vi "GainCurveMeasurement.vi"() -> ()   [LabVIEW 2019]
doc: "Main VI for FLS imaging system."
uses:
  <vilib>/event_ctls.llb/usereventprio.ctl
  <instrlib>/niScope/Acquire/Fetch/niScope Multi Fetch Binary 16.vi
  <instrlib>/niScope/Controls/niScope trigger source.ctl
  <vilib>/Utility/file.llb/Write Delimited Spreadsheet (DBL).vi
  LaguerreDeconLib/DeconEngineClass/LaguerreDeconEngineClass.lvclass
  SubVI/GlobalVariables.vi
  SubVI/LabJack/LJ Pin Setting.ctl
  <vilib>/Utility/error.llb/DialogType.ctl
  <vilib>/Analysis/NI_AALBase.lvlib
  <vilib>/Utility/miscctls.llb/LVMinMaxIncTypeDef.ctl
  <vilib>/Analysis/baseanly.llb/Mean (DBL).vi
  <vilib>/Utility/miscctls.llb/LVPointTypeDef.ctl
  <vilib>/Instr/_visa.llb/VISA Configure Serial Port (Instr).vi
  SubVI/DigitizerConfiguration/FLImDAQ.ctl
panel:
  out "Record Backlog":i32
  out "Fetch Record #":i32
  out "error out 2":errorcluster caption="error out"
  out "error out":errorcluster
  out "Sync Success?":bool
  out "Disclamer":picture
  out "Calibration #":i8
  out "BG #":i8
  in  "TCP Connect":bool
  out "Help":string
  in  "355nm Laser toggle":bool caption="355nm 750Hz"
  in  "Cali&iRF alignment":bool
  in  "Background":bool
  in  "Aiming beam toggle":bool caption="445nm 15Hz 20mA"
  out "Lifetime 3":dbl
  out "Lifetime 2":dbl
  in  "Auto gain ch3":bool=TRUE
  in  "Auto gain ch2":bool=TRUE
  in  "Auto gain ch1":bool=TRUE
  out "Run #":i8
  in  "StopButton":bool caption="Stop"
  out "Aquisition Status:":bool
  in  "StartButton":bool caption="Start"
  in  "Gain 3":dbl min=0.0 max=4.6 step=0.1
  in  "Gain 2":dbl min=0.0 max=4.6 step=0.1
  out "Lifetime 1":dbl
  in  "Gain 1":dbl min=0.0 max=4.6 step=0.1 format="%#_4g"
  in  "Video Source":enum32{"Camera", "FrameGrabber"}(radio)
  out "Case #":string
  out "System Hardware Connection Status":T1
  out "Channel 3":dbl[][](graph)
  out "Channel 2":dbl[][](graph)
  out "Channel 1":dbl[][](graph)
  in  "Tab Control":T2(tab)
  out "Aq L?":bool
  out "ML?":bool
  out "display loop timing(ms)":u32
  out "Aquisition loop timing(ms)":u32
  in  "sine offset":dbl min=0.0 max=4.8 step=0.01
  in  "sine amplitude":dbl
  out "DisplayLoop":i32
  out "processing loop":i32
  out "processing loop timing(ms)":dbl
  in  "V target(1.5)":dbl=1.3 format="%#_13g"
  out "comm loop(ms)":u32
  out "laser EM lamp V":dbl format="%0.6f"
  in  "Show BG":bool
  in  "start Idx":i32
  in  "length":i32=50
  out "SysConfigCluster":T3
  out "LJ Pinout":T4={"Ch1 Bias"="DAC0", "Ch2 Bias"="DAC1", "Ch3 Bias"="DAC2", "355 PWM"="FIO0", "AimingBeam PWM"="FIO2", "Laser Ready"="FIO3", "Interlock"="FIO1", "Laser Start/Stop"="FIO1", "Red LED"="FIO1", "Green LED"="DIO3", "Foot Pedal"="DIO15"}
  out "FLImDAQ":T5={"Digitizer 1"="", "Digitizer 2"="", "Channel"=enum."Channel 0", "trigger source"="VAL_EXTERNAL", "trigger level"=0.5, "trigger delay"=1.35e-07, "min sample rate"=12500000000.0, "min record length"=2500, "vertical range"=1.0, "vertical offset"=-0.25, "Waveform to Avg"=2000} caption="FLIm DAQ Configuration" {"trigger delay" format="%^#.4e"; "trigger level" min=0.0 max=3.5 step=0.5 format="%.2f"; "vertical offset" format="%.4f"; "vertical range" format="%.2f"; "min sample rate" format="%#.2p"}
  out "Dig1 Temp":dbl
  out "Dig2 Temp":dbl
  in  "Sys Reconfig":bool
  out "data out(communcation loop)":string
  out "syctimer data out":string
  out "processing Error Out":errorcluster
  out "aquisition loop Error Out":errorcluster
  out "decon error out":errorcluster
  out "V1":dbl[](array[numeric])
  out "V2":dbl[](array[numeric])
  out "V3":dbl[](array[numeric])
  out "V1 Size":i32
  out "V2 Size":i32
  out "V3 Size":i32
  out "data Size":i32[](array[numeric])
  out "State log":string
  in  "Quit":bool
  in  "Radio Buttons":enum32{"No Selection", "Ch1", "Ch2", "Ch3"}(radio)=enum."Ch1" caption="DeCon Chan"
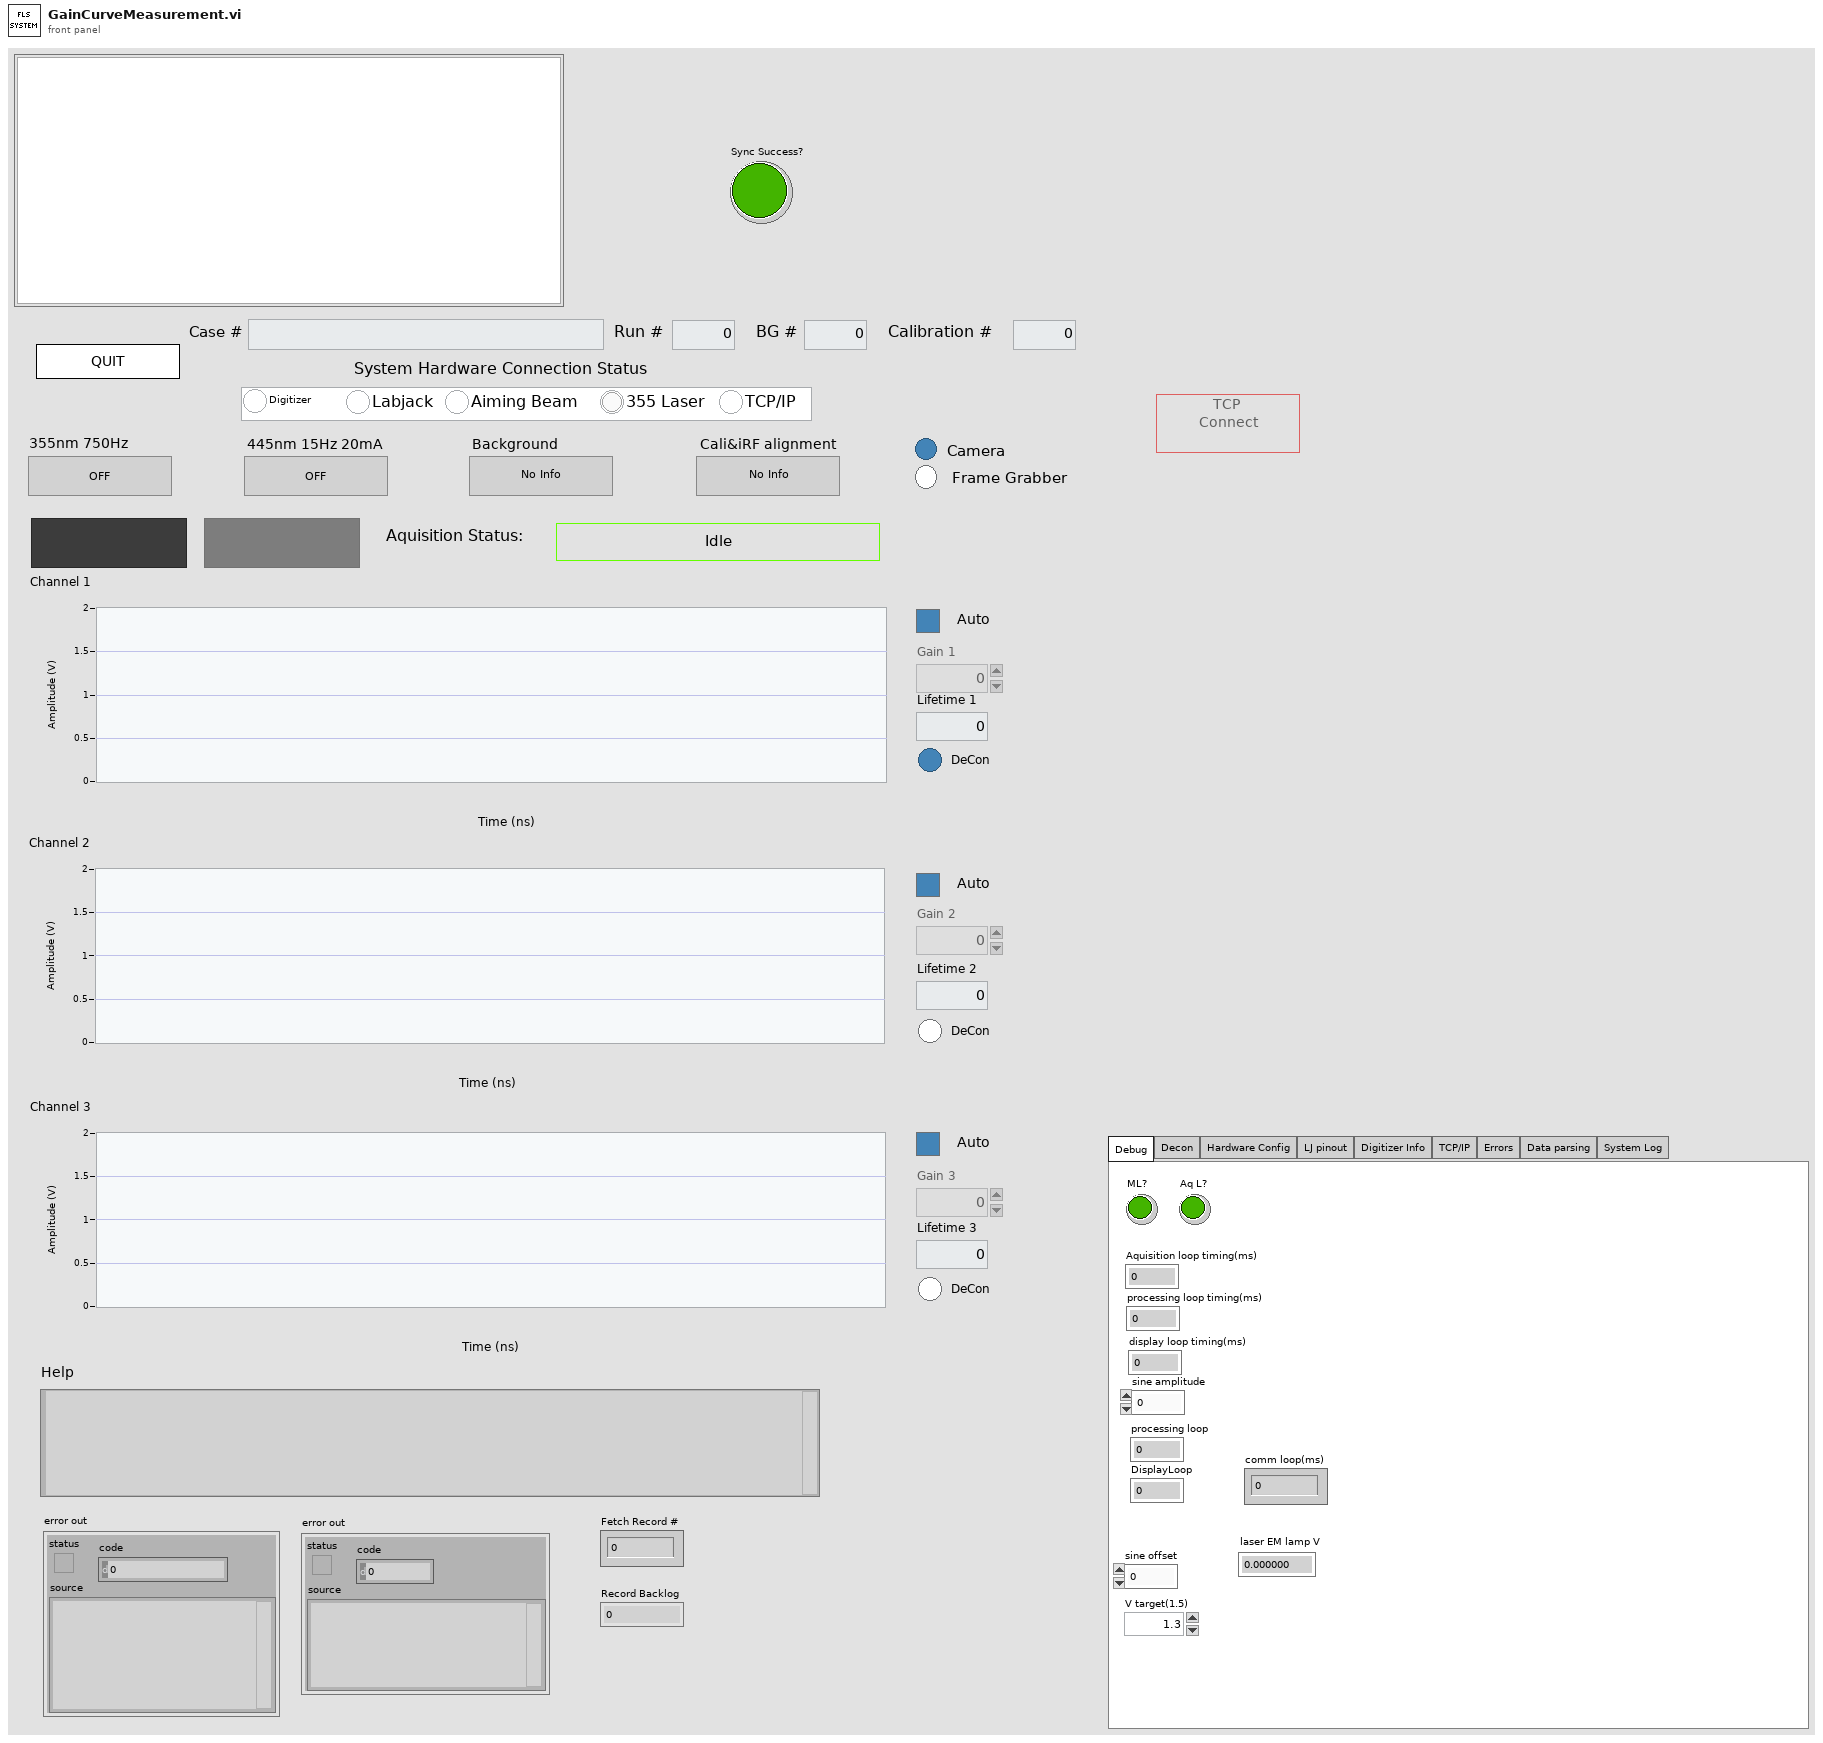
[diagram p1: front panel]
types:
  T1 = cluster{"Digitizer":bool, "Labjack":bool, "Aiming Beam":bool, "355 Laser":bool, "TCP/IP":bool}
  T2 = enum32{"Debug", "Decon", "Hardware Config", "LJ pinout", "Digitizer Info", "TCP/IP", "Errors", "Data parsing", "System Log"}
  T3 = cluster{"Ch1Enable?":bool, "Ch2Enable?":bool, "Ch3Enable?":bool, "Ch1AutoGain?":bool, "Ch2AutoGain?":bool, "Ch3AutoGain?":bool, "AimingBeamEnable?":bool}
  T4 = typedef "LJ Pin Setting.ctl" = cluster{"Ch1 Bias":string, "Ch2 Bias":string, "Ch3 Bias":string, "355 PWM":string, "AimingBeam PWM":string, "Laser Ready":string, "Interlock":string, "Laser Start/Stop":string, "Red LED":string, "Green LED":string, "Foot Pedal":string}
  T5 = typedef "FLImDAQ.ctl" = cluster{"Digitizer 1":refnum<k15>, "Digitizer 2":refnum<k15>, "Channel":enum16{"Channel 0", "Channel 1", "Channel 0&1"}, "trigger source":T6, "trigger level":dbl, "trigger delay":dbl, "min sample rate":dbl, "min record length":i32, "vertical range":dbl, "vertical offset":dbl, "Waveform to Avg":i32}
  T6 = typedef "niScope trigger source.ctl" = string
  T7 = typedef "LVPointTypeDef.ctl" = cluster{"Horizontal":i16, "Vertical":i16}
  T8 = cluster{"CH1":dbl[][], "CH2":dbl[][], "CH3":dbl[][]}
  T9 = cluster{"idx":i32, "CH1&2":dbl[][], "CH3":dbl[][]}
  T10 = enum8{"Enabled", "Disabled", "Disabled and Grayed Out"}
  T11 = enum16{"open", "open or create", "create or replace", "create", "open (read-only)"}
  T12 = enum32{"Invalid", "Standard", "Closed", "Hidden", "Minimized", "Maximized"}
  T13 = enum32{"invalid app kind", "Development System", "Run Time System", "Student Edition", "Embedded LabVIEW", "Evaluation", "Custom"}
  T14 = typedef "usereventprio.ctl" = enum32{"high priority", "normal priority"}
  T15 = enum16{"Standard", "Buffered", "CRLF", "Immediate"}
  T16 = cluster{"Core":cluster{"Current VI Reference":refnum<vi>, "Close Panel on Exit?":bool}, "SysConfigCluster":cluster{"Ch1Enable?":bool, "Ch2Enable?":bool, "Ch3Enable?":bool, "Ch1AutoGain?":bool, "Ch2AutoGain?":bool, "Ch3AutoGain?":bool, "AimingBeamEnable?":bool}, "System Status":cluster{"Digitizer":bool, "Labjack":bool, "Aiming Beam":bool, "355 Laser":bool, "TCP/IP":bool}, "IDs":cluster{"RunID":i8, "BG ID":i8, "Cali ID":i8}, "CaseID":string, "DefaultPath":path, "Pathes":cluster{"DataPath":path, "BG Path":path, "iRFPath":path, "CaliPath":path}, "FLImDAQ":cluster{"resource name":refnum<k15>, "resource name 2":refnum<k15>, "Channel":enum16{"Channel 0", "Channel 1", "Channel 0&1"}, "trigger source":T6, "trigger level":dbl, "trigger delay":dbl, "min sample rate":dbl, "min record length":i32, "vertical range":dbl, "vertical offset":dbl, "Waveform to Avg":i32}, "SysRunning?":bool, "AB Cluster":cluster{"Aiming Beam COM Port":refnum<visa-resource-name>, "Min Current":dbl, "Max Current":dbl, "Default Current":dbl, i32}, "LJ Pinout":T4, "355 PWM setting":cluster{"DIO_EF_CLOCK1_DIVISOR":i16, "DIO_EF_CLOCK1_ROLL_VALUE":i32, "DIO#_EF_INDEX":i16, "DIO#_EF_OPTIONS":i16, "DIO#_EF_CONFIG_A":i32}, "AB PWM setting":cluster{"DIO_EF_CLOCK1_DIVISOR":i16, "DIO_EF_CLOCK1_ROLL_VALUE":i32, "DIO#_EF_INDEX":i16, "DIO#_EF_OPTIONS":i16, "DIO#_EF_CONFIG_A":i32}, "Last Trigger":u32, "niTClk sessions":refnum<k20>[], "Laser start tic":u32, "TCP attempt count":i32, "Ch1Data":dbl[][], "Ch2Data":dbl[][], "Ch3Data":dbl[][], "V1":dbl[], "V2":dbl[], "V3":dbl[], "SlowTimer":u32, "FastTimer":u32, "listener ID":refnum<k5>, "TempPath":path, "LED vi reference":refnum<vi>}
  T17 = typedef "LVCursorListTypeDef.ctl" = cluster{"Name":string, "Color":u32, "Style":u8, "Point Style":u8, "Name Visible":bool, "Allow Drag":bool, "Cursor Mode":u32, "Plot":i32, "Index":i32, "Position":cluster{"X":dbl, "Y":dbl}, "X Scale":u32, "Y Scale":u32, "Watch Plots":i32[], "Watch All Plots":bool, "Plot Area":i32, "Label Offset":cluster{"X":dbl, "Y":dbl}}[]
  T18 = cluster{"Name":string, "Color":u32, "Style":u8, "Point Style":u8, "Name Visible":bool, "Allow Drag":bool, "Cursor Mode":u32, "Plot":i32, "Index":i32, "Position":cluster{"X":dbl, "Y":dbl}, "X Scale":u32, "Y Scale":u32, "Watch Plots":i32[], "Watch All Plots":bool, "Plot Area":i32, "Label Offset":cluster{"X":dbl, "Y":dbl}}
  T19 = cluster{"DataPath":path, "BG Path":path, "iRFPath":path, "CaliPath":path}
  T20 = cluster{"DIO_EF_CLOCK1_DIVISOR":i16, "DIO_EF_CLOCK1_ROLL_VALUE":i32, "DIO#_EF_INDEX":i16, "DIO#_EF_OPTIONS":i16, "DIO#_EF_CONFIG_A":i32}
  T21 = cluster{"Aiming Beam COM Port":refnum<visa-resource-name>, "Min Current":dbl, "Max Current":dbl, "Default Current":dbl, i32}
  T22 = cluster{"resource name":refnum<k15>, "resource name 2":refnum<k15>, "Channel":enum16{"Channel 0", "Channel 1", "Channel 0&1"}, "trigger source":T6, "trigger level":dbl, "trigger delay":dbl, "min sample rate":dbl, "min record length":i32, "vertical range":dbl, "vertical offset":dbl, "Waveform to Avg":i32}
  T23 = cluster{"Current VI Reference":refnum<vi>, "Close Panel on Exit?":bool}
  T24 = cluster{"1D Avg":dbl[], "1D Avg":dbl[], "1D Avg":dbl[]}
  T25 = typedef "DialogType.ctl" = u16
  T26 = cluster{"Ch1 iRF":dbl[], "Ch2 iRF":dbl[], "Ch3 iRF":dbl[]}
  T27 = typedef "LJ PWM Setting.ctl" = cluster{"DIO_EF_CLOCK1_DIVISOR":i16, "DIO_EF_CLOCK1_ROLL_VALUE":i32, "DIO#_EF_INDEX":i16, "DIO#_EF_OPTIONS":i16, "DIO#_EF_CONFIG_A":i32}
  T28 = typedef "AimingBeam.ctl" = cluster{"Aiming Beam COM Port":refnum<visa-resource-name>, "Min Current":dbl, "Max Current":dbl, "Default Current":dbl, "Frequency(Hz)":u32}
  T29 = typedef "LVMinMaxIncTypeDef.ctl" = cluster{"Minimum":dbl, "Maximum":dbl, "Increment":dbl}
  T30 = typedef "LVBoundsTypeDef.ctl" = cluster{"Width":u32, "Height":u32}
  T31 = typedef "imagedata.ctl" = cluster{"image type":i32, "image depth":i32, "image":u8[], "mask":u8[], "colors":u32[], "Rectangle":cluster{"left":i16, "top":i16, "right":i16, "bottom":i16}}
  T32 = cluster{"V1 out":dbl, "V2 out":dbl, "V3 out":dbl}
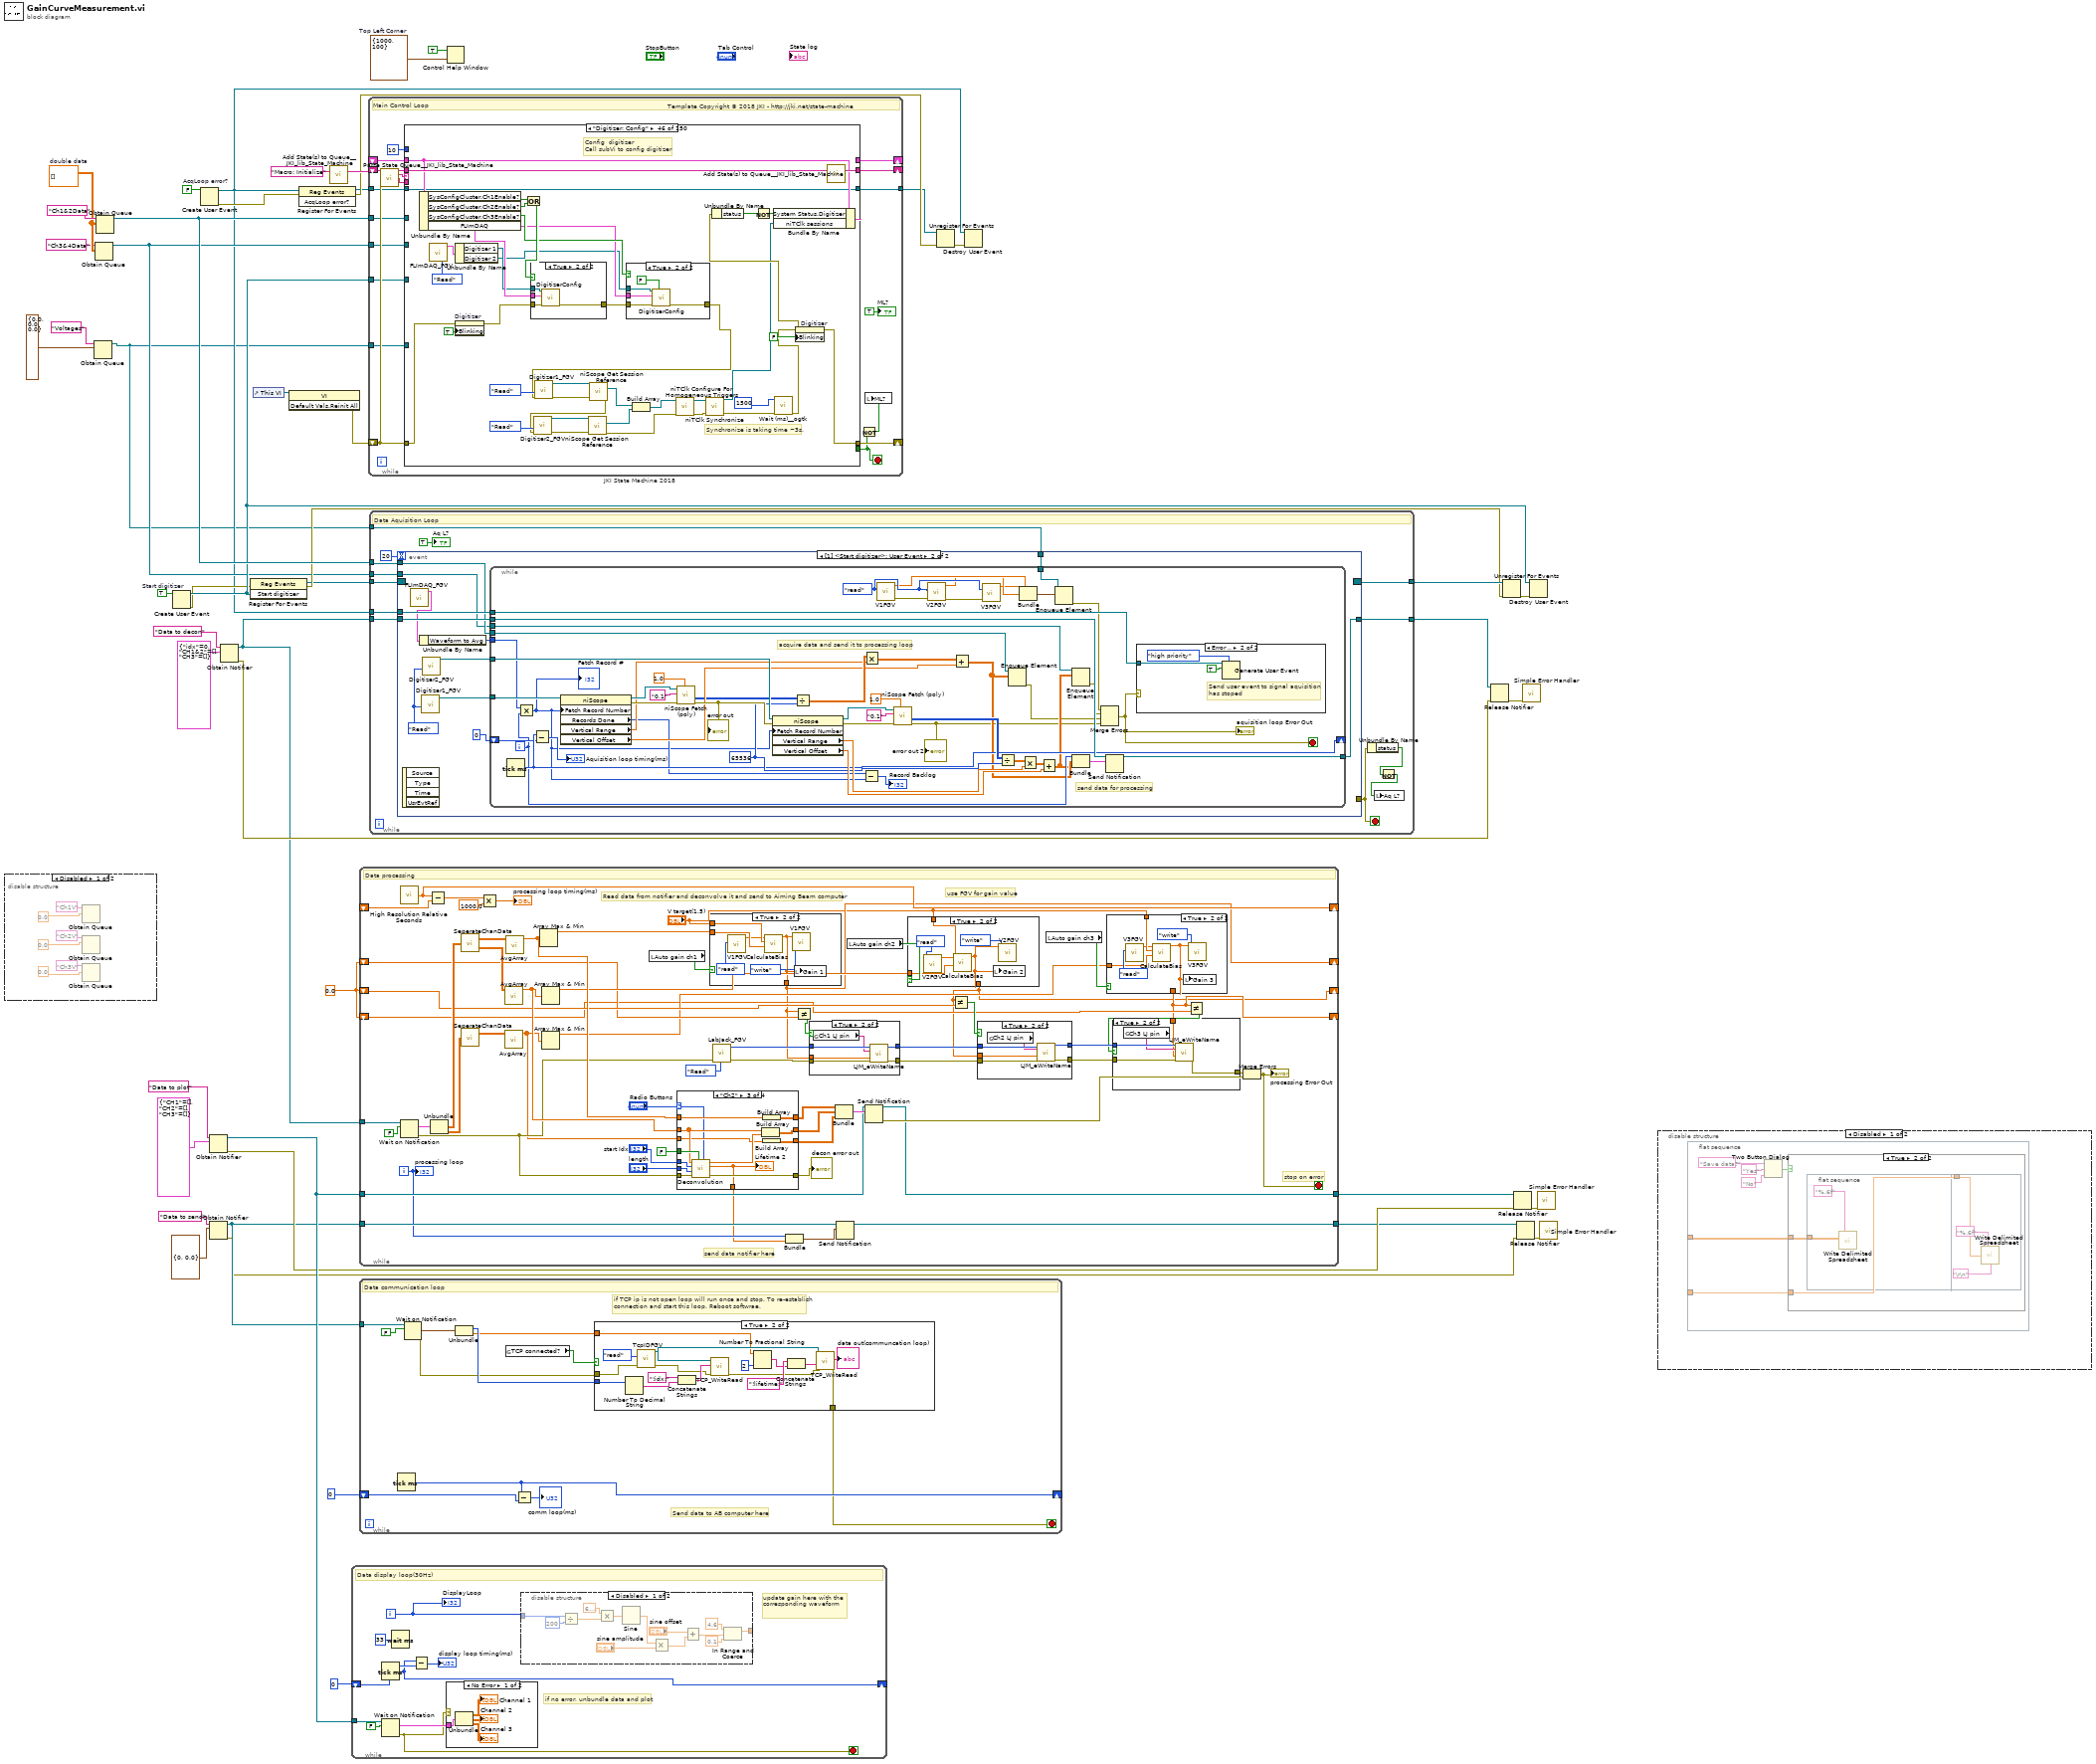
[diagram p0: block diagram]
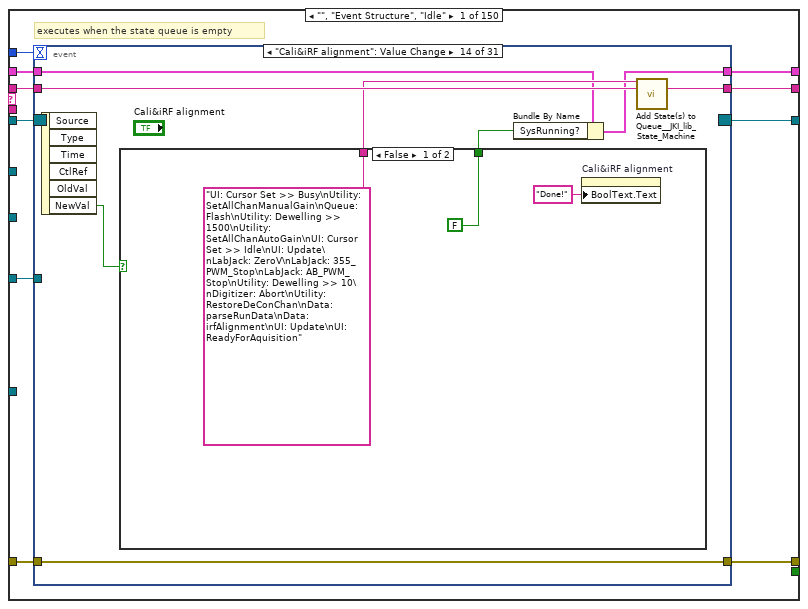
[diagram p3: hidden frame]
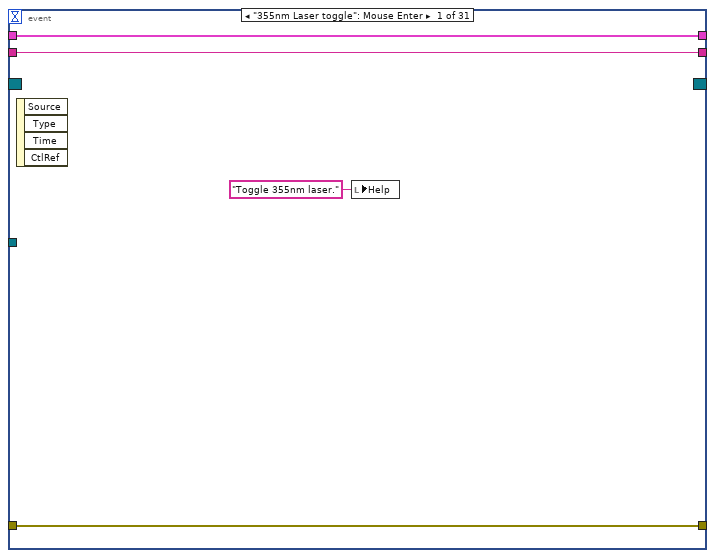
[diagram p4: hidden frame]
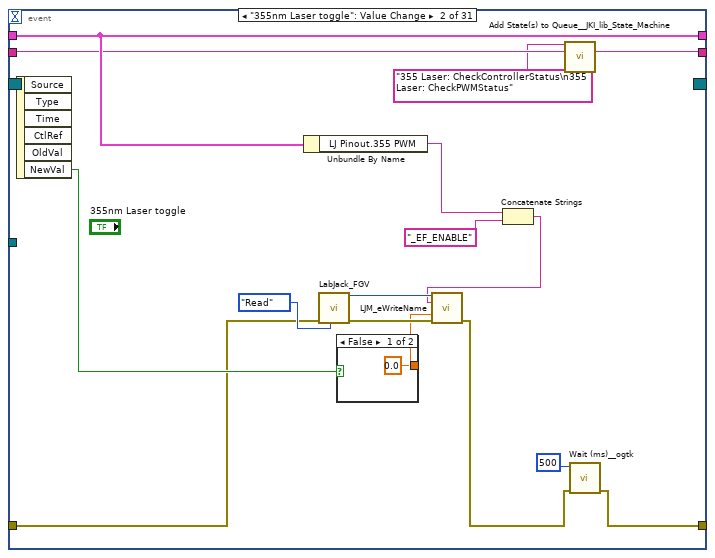
[diagram p5: hidden frame]
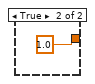
[diagram p6: hidden frame]
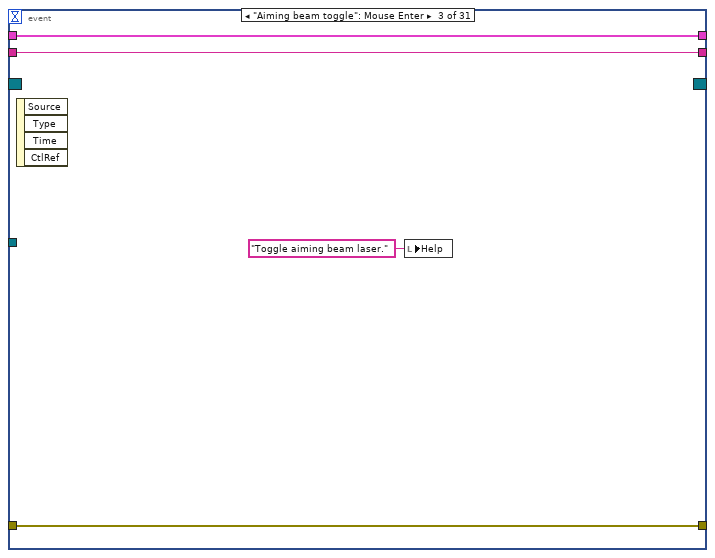
[diagram p7: hidden frame]
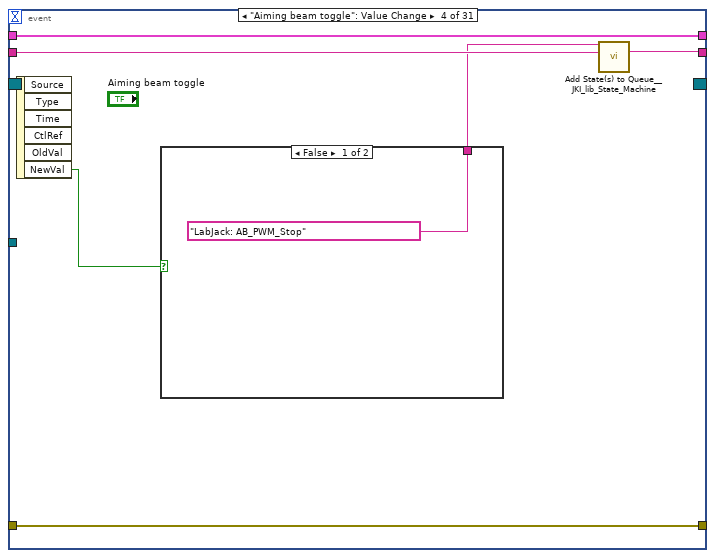
[diagram p8: hidden frame]
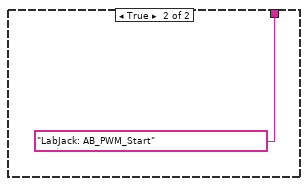
[diagram p9: hidden frame]
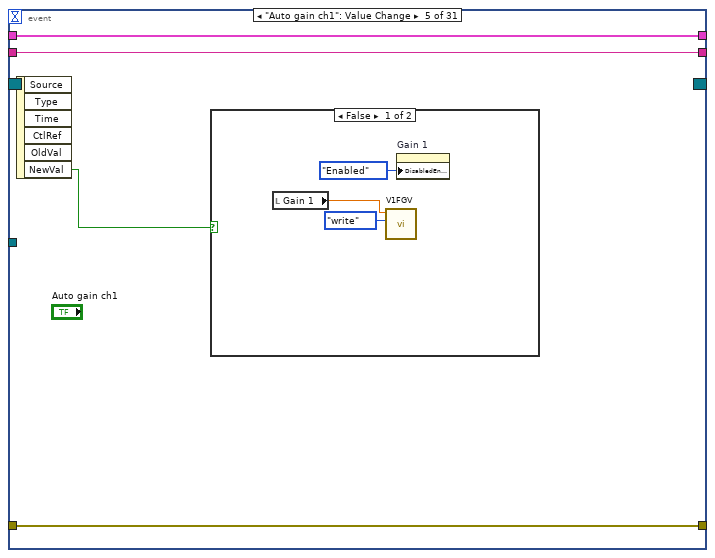
[diagram p10: hidden frame]
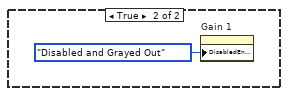
[diagram p11: hidden frame]
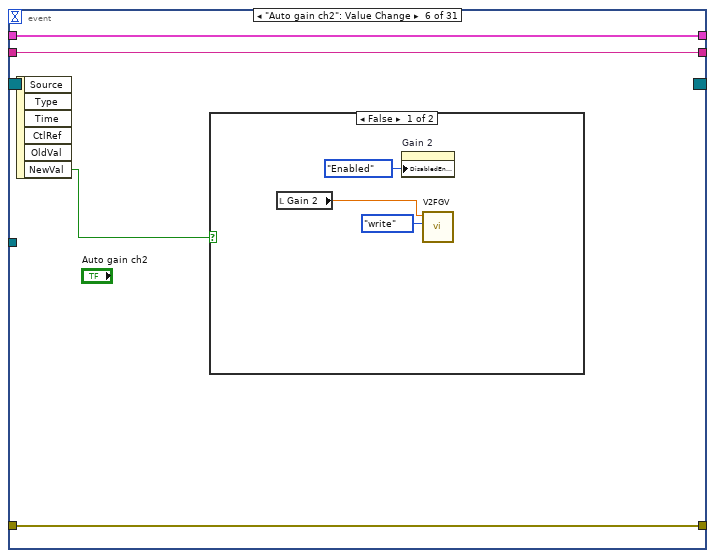
[diagram p12: hidden frame]
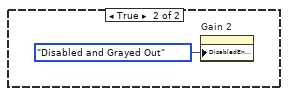
[diagram p13: hidden frame]
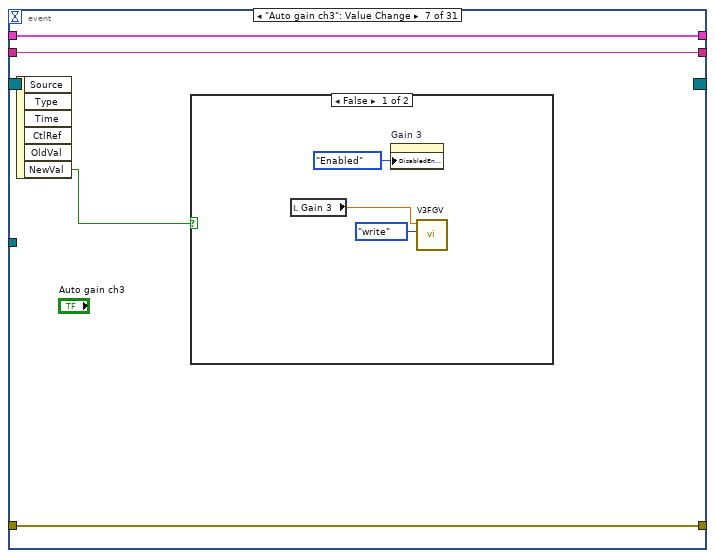
[diagram p14: hidden frame]
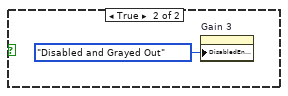
[diagram p15: hidden frame]
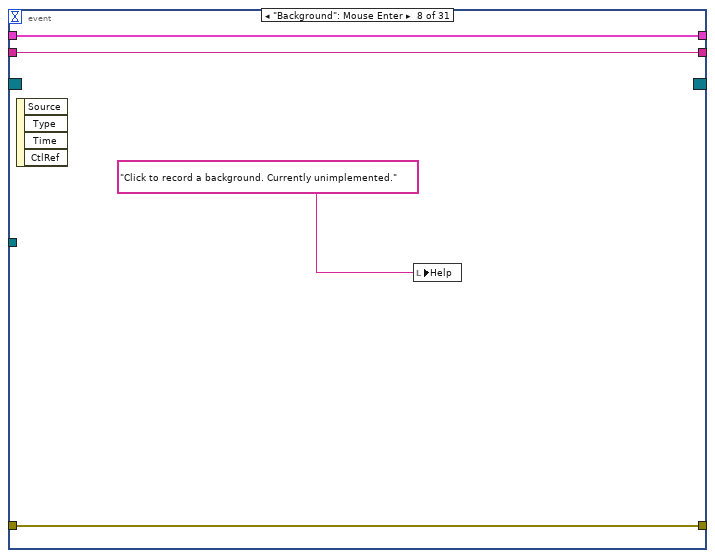
[diagram p16: hidden frame]
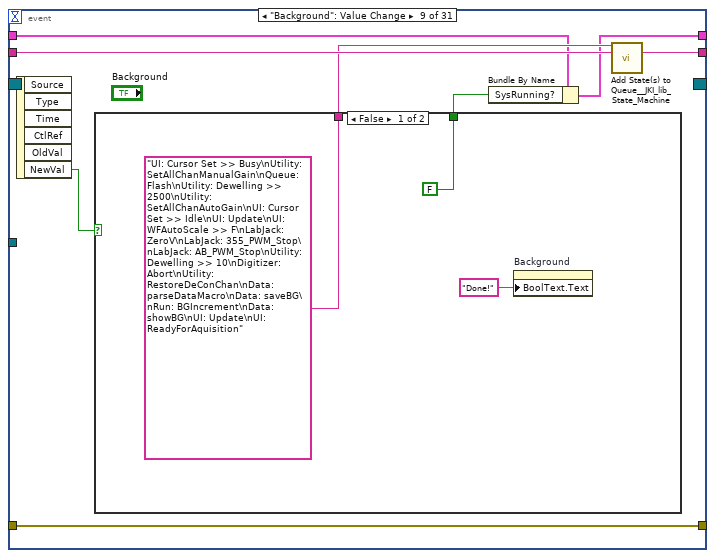
[diagram p17: hidden frame]
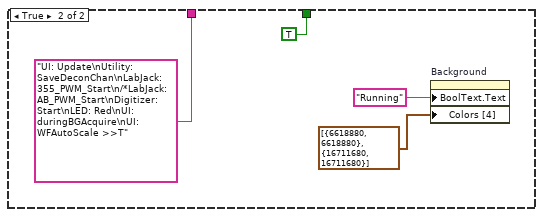
[diagram p18: hidden frame]
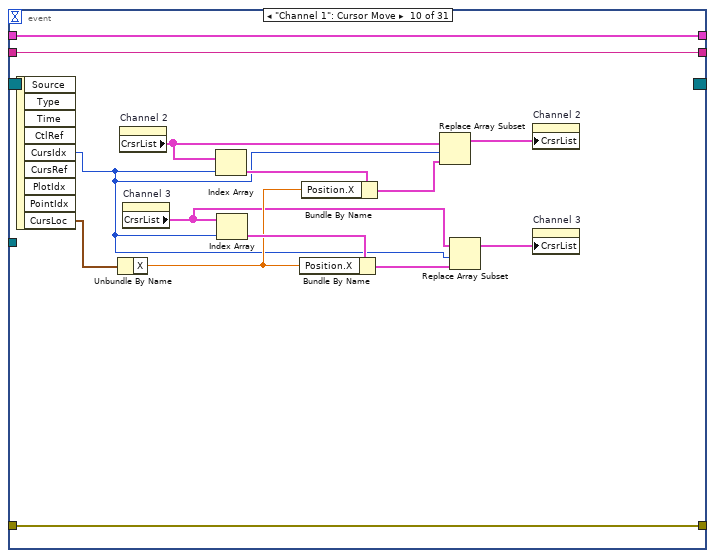
[diagram p19: hidden frame]
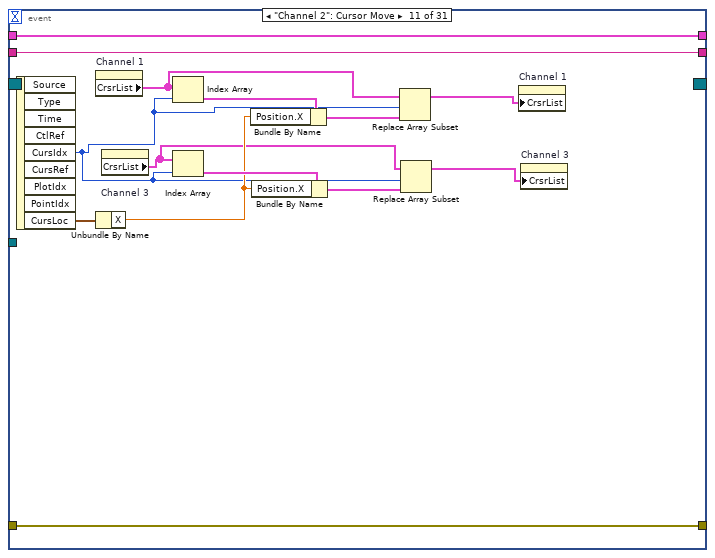
[diagram p20: hidden frame]
diagram:
  w1 = T7 {"Horizontal"=1000, "Vertical"=100}  # Top Left Corner
  w6 = 0.0
  w31 = FALSE  # AcqLoop error?
  w42 = TRUE  # Start digitizer
  w45 = dbl[][] []  # double data
  n1 = disable-structure shown="Disabled" {
    frame Disabled {
      n2 = Obtain Queue(name (unnamed)="Ch1V", element data type=0.0) -> ()  [unwired: 3 in, 3 out]
      n3 = Obtain Queue(name (unnamed)="Ch2V", element data type=0.0) -> ()  [unwired: 3 in, 3 out]
      n4 = Obtain Queue(name (unnamed)="Ch3V", element data type=0.0) -> ()  [unwired: 3 in, 3 out]
    }
    frame Enabled {
    }
  }
  n5 = Obtain Queue(name (unnamed)="Voltages", element data type=cluster{"V1":dbl, "V2":dbl, "V3":dbl} {"V1"=0.0, "V2"=0.0, "V3"=0.0}) -> (queue out=w3:refnum<queue>)  [unwired: 3 in, 2 out]
  n6 = Obtain Queue(name (unnamed)="Ch3&4Data", element data type=w45) -> (queue out=w19:refnum<queue>)  [unwired: 3 in, 2 out]
  n7 = Obtain Queue(name (unnamed)="Ch1&2Data", element data type=w45) -> (queue out=w43:refnum<queue>)  [unwired: 3 in, 2 out]
  n8 = Create User Event(user event datatype=w42) -> (user event=w30:refnum<user-event>, error out=w9:errorcluster)  [unwired: 1 in]
  n9 = Create User Event(user event datatype=w31) -> (user event=w8:refnum<user-event>, error out=w10:errorcluster)  [unwired: 1 in]
  n10 = Obtain Notifier(name (unnamed)="Data to plot", notification data type=T8 {"CH1"=[], "CH2"=[], "CH3"=[]}) -> (notifier out=w23:refnum<notifier>, error out=w20:errorcluster)  [unwired: 2 in, 1 out]
  n11 = Obtain Notifier(name (unnamed)="Data to send", notification data type=cluster{"idx":i32, "lifetime":dbl} {"idx"=0, "lifetime"=0.0}) -> (notifier out=w14:refnum<notifier>, error out=w7:errorcluster)  [unwired: 2 in, 1 out]
  n12 = Obtain Notifier(name (unnamed)="Data to decon", notification data type=T9 {"idx"=0, "CH1&2"=[], "CH3"=[]}) -> (notifier out=w26:refnum<notifier>, error out=w36:errorcluster)  [unwired: 2 in, 1 out]
  n13 = register-events(error in=w9, w30) -> (reference out=w32:refnum<event-registration>, error out=w39:errorcluster)  [unwired: 1 in]
  n14 = control-ref of="This VI"() -> (w47:refnum<vi>)
  n15 = invoke class="VI" method="Default Vals.Reinit All"(reference=w47) -> (error out=w33:errorcluster)  [unwired: 2 in, 2 out]
  n16 = register-events(error in=w10, w8) -> (reference out=w18:refnum<event-registration>, error out=w28:errorcluster)  [unwired: 1 in]
  n17 = call <vilib>:"Add State(s) to Queue__JKI_lib_State_Machine.vi"("State(s) in (\"\")"="Macro: Initialize") -> ("States Out"=w49:string)  [unwired: 14 in]
  n18 = while {
    tunnel: w23 -> [w64]
    shift-right: [w57] -> _
    shift-left: u32 0 ("millisecond timer value") -> [w62]
    i -> [w60]
    stop <- w56 stop-if-true
    # "if no error, unbundle data and plot"
    # "update gain here with the corresponding waveform"
    # "Data display loop(30Hz)"
    n19 = Tick Count (ms)() -> (millisecond timer value=w57:u32)
    n20 = Wait on Notification(notifier=w64, ignore previous (F)=FALSE) -> (notification=w58:T8, error out=w56:errorcluster)  [unwired: 2 in, 2 out]
    n21 = Wait (ms)(milliseconds to wait=u32 33) -> ()  [unwired: 1 out]
    n22 = Subtract(x=w57, y=w62) -> (x-y=→"display loop timing(ms)":u32)
    n23 = case shown="No Error" w56 {
      tunnel: w58 -> [w68 _]
      frame No Error {
        n24 = Unbundle(w68) -> ("CH1"=→"Channel 1":dbl[][], "CH2"=→"Channel 2":dbl[][], "CH3"=→"Channel 3":dbl[][])
      }
      frame Error {
      }
    }
    n25 = disable-structure shown="Disabled" {
      disable-tunnel: w60 -> [w70 _]
      disable-tunnel: [w69 _] -> _
      frame Disabled {
        n26 = Divide(x=w70, y=200) -> (x/y=w80:dbl)
        n27 = Multiply(x=6.283185307179586, y=w80) -> (x*y=w78:dbl)
        n28 = Sine(x=w78) -> (sin(x)=w76:dbl)
        n29 = Multiply(x=w76, y="sine amplitude") -> (x*y=w77:dbl)
        n30 = Add(x="sine offset", y=w77) -> (x+y=w75:dbl)
        n31 = In Range and Coerce(upper limit=4.6, x=w75, lower limit=0.1) -> (coerced(x)=w69:dbl)  [unwired: 1 out]
      }
      frame Enabled {
      }
    }
    "DisplayLoop" <- w60
  }
  n32 = while {
    tunnel: w14 -> [w92]
    shift-right: [w85] -> _
    shift-left: u32 0 -> [w86]
    stop <- w83 stop-if-true
    # "Send data to AB computer here"
    # "if TCP ip is not open loop will run once and stop. To re-establish connection and start this loop. Reboot softwrae."
    # "Data communication loop"
    n33 = Tick Count (ms)() -> (millisecond timer value=w85:u32)
    n34 = Wait on Notification(notifier=w92, ignore previous (F)=FALSE) -> (notification=w90:cluster{"idx":i32, "lifetime":dbl}, error out=w84:errorcluster)  [unwired: 2 in, 2 out]
    n35 = Unbundle(w90) -> ("idx"=w89:i32, "lifetime"=w88:dbl)
    n36 = global read "GlobalVariables.vi" "TCP connected?"() -> (w82:bool)
    n37 = Subtract(x=w85, y=w86) -> (x-y=→"comm loop(ms)":u32)
    n38 = case shown="True" w82 {
      tunnel: w89 -> [_ w101]
      tunnel: w88 -> [_ w100]
      tunnel: w84 -> [w93 w97]
      tunnel: [w93 w94] -> w83
      frame False {
      }
      frame True {
        n39 = Number To Decimal String(number=w101) -> (decimal integer string=w109:string)  [unwired: 1 in]
        n40 = call "TcpIDFGV.vi"("Error In"=w97, "action"=enum16{"write", "read"}."read") -> ("Error Out"=w96:errorcluster, "connection ID out"=w107:refnum<k5>)  [unwired: 8 in]
        n41 = Concatenate Strings("!idx:", w109) -> (w110:string)
        n42 = call "TCP_WriteRead.vi"("error in (no error)"=w96, "data in"=w110, "connectin ID in"=w107) -> ("error out"=w95:errorcluster, "connectin ID out"=w108:refnum<k5>)  [unwired: 4 in, 1 out]
        n43 = Number To Fractional String(number=w100, precision (6)=i16 2) -> (F-format string=w99:string)  [unwired: 2 in]
        n44 = Concatenate Strings("!lifetime:", w99) -> (w106:string)
        n45 = call "TCP_WriteRead.vi"("error in (no error)"=w95, "data in"=w106, "connectin ID in"=w108) -> ("error out"=w94:errorcluster, "data out"=→"data out(communcation loop)":string)  [unwired: 4 in, 1 out]
      }
    }
  }
  n46 = while {
    tunnel: w26 -> [w169]
    shift-right: [w114] -> _
    shift-left: w6 -> [w121]
    tunnel: w23 -> [w161]
    tunnel: [w158] -> w22
    shift-right: [w157] -> _
    shift-left: _ -> [w156]
    shift-right: [w115] -> _
    shift-left: w6 -> [w122]
    shift-right: [w116] -> _
    shift-left: w6 -> [w118]
    tunnel: w14 -> [w134]
    tunnel: [w130] -> w13
    i -> [w133]
    stop <- w129 stop-if-true
    # "use FGV for gain value"
    # "send data notifier here"
    # "stop on error"
    # "Read data from notifier and deconvolve it and send to Aiming Beam computer"
    # "Data processing"
    n47 = call <vilib>:"High Resolution Relative Seconds.vi"() -> ("relative seconds"=w157:dbl)
    n48 = Wait on Notification(notifier=w169, ignore previous (F)=FALSE) -> (notification=w167:T9, error out=w146:errorcluster)  [unwired: 2 in, 2 out]
    n49 = Subtract(x=w157, y=w156) -> (x-y=w155:dbl)
    n50 = Unbundle(w167) -> ("CH1&2"=w136:dbl[][], "CH3"=w135:dbl[][])  [unwired: 1 out]
    n51 = call "SeperateChanData.vi"("Input (Ch1&2)"=w136) -> ("Ch1"=w138:dbl[][], "Ch2"=w143:dbl[][])
    n52 = call "SeperateChanData.vi"("Input (Ch1&2)"=w135) -> ("Ch1"=w166:dbl[][])  [unwired: 1 out]
    n53 = Multiply(x=w155, y=1000.0) -> (x*y=→"processing loop timing(ms)":dbl)
    n54 = call "AvgArray.vi"("2D array"=w143) -> ("1D Avg"=w152:dbl[])  [unwired: 10 in]
    n55 = call "AvgArray.vi"("2D array"=w166) -> ("1D Avg"=w142:dbl[])  [unwired: 10 in]
    n56 = call "AvgArray.vi"("2D array"=w138) -> ("1D Avg"=w159:dbl[])  [unwired: 10 in]
    n57 = Array Max & Min(array=w159) -> (max value=w125:dbl)  [unwired: 3 out]
    n58 = Array Max & Min(array=w152) -> (max value=w123:dbl)  [unwired: 3 out]
    n59 = Array Max & Min(array=w142) -> (max value=w119:dbl)  [unwired: 3 out]
    n60 = local read "Auto gain ch1"() -> (w128:bool)
    n61 = case shown="\"Ch2\"" "Radio Buttons" {
      selector: "Radio Buttons" -> [_ w224 w238 w252]
      tunnel: w159 -> [w223 w232 w244 w257]
      tunnel: w152 -> [w221 w229 w246 w255]
      tunnel: w142 -> [w219 w227 w241 w260]
      tunnel: FALSE -> [_ w237 w251 w265]
      tunnel: w146 -> [w217 w236 w248 w262]
      tunnel: "length" -> [_ w235 w249 w263]
      tunnel: "start Idx" -> [_ w234 w250 w264]
      tunnel: [w217 w233 w247 w261] -> w137
      tunnel: [w222 w230 w242 w256] -> w141
      tunnel: [w220 w228 w243 w254] -> w140
      tunnel: [w218 w226 w240 w258] -> w139
      tunnel: [0.0 ("lifetime (ns)") w225 w239 w253] -> w132
      frame "No Selection", Default {
        n62 = Build Array(w223) -> (w222:dbl[][])
        n63 = Build Array(w221) -> (w220:dbl[][])
        n64 = Build Array(w219) -> (w218:dbl[][])
      }
      frame "Ch1" {
        n65 = call "Deconvolution.vi"("DeconChannel"=w224, "iRF align"=w237, "error in (no error)"=w236, 9:w235, 10:w234, "Waveform"=w232) -> ("error out"=w233:errorcluster, "lifetime (ns)"=w225:dbl, "Fitting"=w231:dbl[])  [unwired: 3 in]
        "Lifetime 1" <- w225
        n66 = Build Array(w232, w231) -> (w230:dbl[][])
        n67 = Build Array(w229) -> (w228:dbl[][])
        n68 = Build Array(w227) -> (w226:dbl[][])
      }
      frame "Ch2" {
        n69 = call "Deconvolution.vi"("DeconChannel"=w238, "iRF align"=w251, "error in (no error)"=w248, 9:w249, 10:w250, "Waveform"=w246) -> ("error out"=w247:errorcluster, "lifetime (ns)"=w239:dbl, "Fitting"=w245:dbl[])  [unwired: 3 in]
        "Lifetime 2" <- w239
        n70 = Build Array(w246, w245) -> (w243:dbl[][])
        n71 = Build Array(w244) -> (w242:dbl[][])
        n72 = Build Array(w241) -> (w240:dbl[][])
      }
      frame "Ch3" {
        n73 = call "Deconvolution.vi"("DeconChannel"=w252, "iRF align"=w265, "error in (no error)"=w262, 9:w263, 10:w264, "Waveform"=w260) -> ("error out"=w261:errorcluster, "lifetime (ns)"=w253:dbl, "Fitting"=w259:dbl[])  [unwired: 3 in]
        "Lifetime 3" <- w253
        n74 = Build Array(w260, w259) -> (w258:dbl[][])
        n75 = Build Array(w257) -> (w256:dbl[][])
        n76 = Build Array(w255) -> (w254:dbl[][])
      }
    }
    "decon error out" <- w137
    n77 = case shown="True" w128 {
      tunnel: [w208 w212] -> w114
      tunnel: w125 -> [_ w214]
      tunnel: "V target(1.5)" -> [_ w213]
      frame False {
        n78 = call "V1FGV.vi"("action"=enum16{"write", "read"}."read") -> ("V1 out"=w208:dbl)  [unwired: 9 in, 1 out]
      }
      frame True {
        n79 = call "V1FGV.vi"("action"=enum16{"write", "read"}."read") -> ("V1 out"=w210:dbl)  [unwired: 9 in, 1 out]
        n80 = call "CalculateBias.vi"("GainV Last"=w214, "Sig Current(V)"=w213, "GainV current"=w210) -> ("V new"=w212:dbl)  [unwired: 8 in]
        n81 = call "V1FGV.vi"("action"=enum16{"write", "read"}."write", "V1 in"=w212) -> ()  [unwired: 8 in, 2 out]
        n82 = local write "Gain 1"(w212) -> ()
      }
    }
    n83 = call "LabJack_FGV.vi"("Operation(Read)"=enum16{"Write", "Read"}."Read" ("Operation"), "error in (no error)"=w146) -> ("error out"=w165:errorcluster, "Read data"=w164:i32)  [unwired: 8 in]
    n84 = Bundle(w133, "lifetime (ns)"=w132) -> (w131:cluster{i32, "lifetime (ns)":dbl})  [unwired: 1 in]
    n85 = Not Equal?(x=w114, y=w121) -> (x != y?=w124:bool)
    n86 = case shown="True" w124 {
      tunnel: w165 -> [w185 w191]
      tunnel: w164 -> [w184 w190]
      tunnel: [w185 w189] -> w151
      tunnel: [w184 w188] -> w148
      tunnel: w114 -> [_ w186]
      frame False {
      }
      frame True {
        n87 = global read "GlobalVariables.vi" "Ch1 LJ pin"() -> (w187:string)
        n88 = call <vilib>:"LJM_eWriteName.vi"("Handle In"=w190, "Name"=w187, "Value"=w186, "error in"=w191) -> ("Handle Out"=w188:i32, "error out"=w189:errorcluster)  [unwired: 10 in]
      }
    }
    n89 = Bundle(w141, w140, w139) -> (w162:cluster{dbl[][], dbl[][], dbl[][]})  [unwired: 1 in]
    n90 = Send Notification(notification=w131, notifier=w134) -> (notifier out=w130:refnum<notifier>)  [unwired: 1 in, 1 out]
    n91 = local read "Auto gain ch2"() -> (w127:bool)
    n92 = Send Notification(notification=w162, notifier=w161) -> (notifier out=w158:refnum<notifier>, error out=w160:errorcluster)  [unwired: 1 in]
    n93 = case shown="True" w127 {
      tunnel: [w200 w202] -> w115
      tunnel: w123 -> [_ w207]
      tunnel: "V target(1.5)" -> [_ w206]
      frame False {
        n94 = call "V2FGV.vi"("action"=enum16{"write", "read"}."read") -> ("V2 out"=w200:dbl)  [unwired: 9 in, 1 out]
      }
      frame True {
        n95 = call "V2FGV.vi"("action"=enum16{"write", "read"}."read") -> ("V2 out"=w204:dbl)  [unwired: 9 in, 1 out]
        n96 = call "CalculateBias.vi"("GainV Last"=w207, "Sig Current(V)"=w206, "GainV current"=w204) -> ("V new"=w202:dbl)  [unwired: 8 in]
        n97 = local write "Gain 2"(w202) -> ()
        n98 = call "V2FGV.vi"("action"=enum16{"write", "read"}."write", "V2 in"=w202) -> ()  [unwired: 8 in, 2 out]
      }
    }
    n99 = Not Equal?(x=w115, y=w122) -> (x != y?=w120:bool)
    n100 = case shown="True" w120 {
      tunnel: w151 -> [w176 w183]
      tunnel: [w176 w182] -> w150
      tunnel: w148 -> [w177 w181]
      tunnel: [w177 w180] -> w147
      tunnel: w115 -> [_ w178]
      frame False {
      }
      frame True {
        n101 = global read "GlobalVariables.vi" "Ch2 LJ pin"() -> (w179:string)
        n102 = call <vilib>:"LJM_eWriteName.vi"("Handle In"=w181, "Name"=w179, "Value"=w178, "error in"=w183) -> ("Handle Out"=w180:i32, "error out"=w182:errorcluster)  [unwired: 10 in]
      }
    }
    n103 = local read "Auto gain ch3"() -> (w126:bool)
    n104 = case shown="True" w126 {
      tunnel: w119 -> [_ w198]
      tunnel: "V target(1.5)" -> [_ w197]
      tunnel: [w192 w194] -> w116
      frame False {
        n105 = call "V3FGV.vi"("action"=enum16{"write", "read"}."read") -> ("V3 out"=w192:dbl)  [unwired: 9 in, 1 out]
      }
      frame True {
        n106 = call "V3FGV.vi"("action"=enum16{"write", "read"}."read") -> ("V3 out"=w196:dbl)  [unwired: 9 in, 1 out]
        n107 = call "CalculateBias.vi"("GainV Last"=w198, "Sig Current(V)"=w197, "GainV current"=w196) -> ("V new"=w194:dbl)  [unwired: 8 in]
        n108 = local write "Gain 3"(w194) -> ()
        n109 = call "V3FGV.vi"("action"=enum16{"write", "read"}."write", "V3 in"=w194) -> ()  [unwired: 8 in, 2 out]
      }
    }
    n110 = Not Equal?(x=w116, y=w118) -> (x != y?=w117:bool)
    n111 = case shown="True" w117 {
      tunnel: w150 -> [w170 w175]
      tunnel: [w170 w174] -> w149
      tunnel: w147 -> [_ w173]
      tunnel: w116 -> [_ w171]
      frame False {
      }
      frame True {
        n112 = global read "GlobalVariables.vi" "Ch3 LJ pin"() -> (w172:string)
        n113 = call <vilib>:"LJM_eWriteName.vi"("Handle In"=w173, "Name"=w172, "Value"=w171, "error in"=w175) -> ("error out"=w174:errorcluster)  [unwired: 10 in, 1 out]
      }
    }
    n114 = Merge Errors(w149, w160) -> (w129:errorcluster)
    "processing Error Out" <- w129
    "processing loop" <- w133
  }
  n115 = while "JKI State Machine 2018" {
    shift-right: [w279] -> _
    shift-left: _ -> [w278]
    shift-right: [w281] -> _
    shift-left: w33 -> [w276]
    shift-right: [w280] -> _
    shift-left: w49 -> [w282]
    tunnel: w43 -> [w275]
    tunnel: w19 -> [w274]
    tunnel: w30 -> [w273]
    tunnel: w18 -> [w272]
    tunnel: [w271] -> w17
    tunnel: w3 -> [w267]
    stop <- w270 stop-if-true
    # "Template Copyright © 2018 JKI - http://jki.net/state-machine"
    # "Main Control Loop"
    n116 = call <vilib>:"Parse State Queue__JKI_lib_State_Machine.vi"("State Queue"=w282, "Error In (no error)"=w276) -> ("Remaining States"=w284:string, "Current State"=w266:string, "Arguments"=w283:string)  [unwired: 11 in]
    n117 = case shown="\"Digitizer: Config\"" w266 {
      selector: w266 -> [_ _ _ _ _ _ _ _ _ _ _ _ _ _ _ _ _ w954 _ _ _ _ _ _ _ _ _ _ _ _ _ _ _ _ _ _ _ _ _ _ _ _ _ _ _ _ _ _ _ _ _ _ _ _ _ _ _ _ _ _ _ _ _ _ _ _ _ _ _ _ _ _ _ _ _ _ _ _ _ _ _ _ _ _ _ _ _ _ _ _ _ _ _ _ _ _ _ _ _ _ _ _ _ _ _ _ _ _ _ _ _ _ _ _ _ _ _ _ _ _ _ _ _ _ _ _ _ _ _ _ _ _ _ _ _ _ _ _ _ _ _ _ _ _ _ _ _ _ _ _]
      tunnel: w284 -> [w294 w570 w603 w609 w635 w661 w685 w708 w724 w759 w787 w822 w827 w896 w938 w947 w952 w958 w983 w991 w1014 w1019 w1028 w1034 w1057 w1072 w1084 w1093 w1115 w1124 w1146 w1153 w1167 w1187 w1210 w1236 w1274 w1279 w1285 w1312 w1339 w1366 w1371 w1376 w1394 w1444 w1466 w1482 w1494 w1510 w1515 w1527 w1569 w1580 w1618 w1629 w1635 w1646 w1658 w1689 w1720 w1733 w1746 w1760 w1774 w1779 w1788 w1795 w1803 w1828 w1843 w1858 w1873 w1878 w1883 w1892 w1904 w1909 w1917 w1925 w1933 w1941 w1946 w1955 w1972 w1988 w2008 w2029 w2037 w2042 w2050 w2058 w2063 w2089 w2122 w2162 w2178 w2192 w2204 w2214 w2227 w2247 w2257 w2273 w2283 w2293 w2307 w2317 w2327 w2337 w2347 w2357 w2362 w2369 w2376 w2386 w2404 w2422 w2430 w2437 w2445 w2450 w2457 w2463 w2469 w2477 w2490 w2497 w2509 w2579 w2590 w2611 w2619 w2625 w2631 w2646 w2691 w2699 w2705 w2710 w2716 w2721 w2731 w2739 w2747 w2752 w2757 w2762 w2775 w2788]
      tunnel: w283 -> [_ _ _ _ _ _ _ _ _ _ _ _ _ _ _ _ _ _ _ _ _ _ _ _ _ _ _ _ _ w1121 _ _ _ _ _ _ _ _ _ _ _ _ _ _ _ _ _ _ _ _ _ _ _ _ _ _ _ _ w1656 _ _ _ _ _ _ _ _ _ w1796 _ _ _ _ _ _ _ _ _ _ _ _ _ _ _ _ _ _ _ _ _ _ _ _ _ _ _ _ _ _ _ _ _ _ _ _ _ _ _ _ _ _ _ _ _ _ w2377 _ _ _ _ _ _ _ _ _ _ _ w2492 w2503 _ _ _ w2615 _ _ _ _ _ _ _ _ _ w2726 _ _ _ _ _ _ _]
      tunnel: w278 -> [w292 w567 _ w606 w627 w651 w676 w700 w720 w756 w777 w819 w824 w854 w935 w942 w949 w956 w976 w988 w1012 w1016 w1024 w1031 w1054 w1069 w1074 w1087 w1113 w1122 w1133 w1150 w1155 w1174 w1199 w1228 w1270 w1276 w1282 w1289 w1317 w1343 w1368 w1373 w1387 w1434 w1463 w1467 w1491 w1507 w1512 w1516 w1558 w1573 w1597 w1627 w1632 w1639 w1654 w1672 w1703 w1728 w1741 w1752 w1765 w1776 w1783 w1789 w1800 w1816 w1831 w1847 w1862 w1875 w1880 w1890 w1902 w1906 w1911 w1918 w1928 w1936 w1943 w1952 w1957 w1975 w2003 w2011 w2034 w2039 w2043 w2051 w2060 w2069 w2120 w2158 w2168 w2190 w2202 w2212 w2225 w2243 w2249 w2269 w2281 w2291 w2305 w2315 w2325 w2335 w2345 w2355 w2359 w2366 w2373 w2383 w2402 w2419 w2427 w2434 w2442 w2447 w2455 w2461 w2466 w2475 w2487 w2495 w2505 w2576 w2587 w2595 w2616 w2622 w2628 w2639 w2687 w2696 w2702 w2707 w2713 w2718 w2728 w2736 w2744 w2749 w2754 w2759 w2772 w2785]
      tunnel: [w291 w568 w601 w607 w624 w659 w674 w697 w722 w737 w764 w800 w825 w889 w904 w943 w950 w960 w980 errorcluster {"status"=FALSE, "code"=0, "source"=""} ("error out") w1011 w1017 w1026 w1032 w1055 w1070 w1078 w1090 w1105 w1118 w1134 w1151 w1165 w1185 w1208 w1227 w1272 w1277 w1283 w1290 w1318 w1344 w1369 w1374 w1384 w1425 w1457 w1471 w1492 w1498 w1513 w1519 w1549 w1571 w1585 w1621 w1633 w1644 w1648 w1663 w1694 w1723 w1736 w1751 w1764 w1777 w1781 w1791 w1798 w1818 w1833 w1848 w1863 w1876 w1881 w1884 w1899 w1907 w1915 w1923 w1931 w1939 w1944 w1948 w1960 w1983 w2002 w2023 w2032 w2040 w2048 w2056 w2061 w2071 w2117 w2160 w2166 w2180 w2196 w2206 w2215 w2245 w2248 w2263 w2275 w2286 w2298 w2309 w2320 w2329 w2339 w2349 w2360 w2367 w2374 w2384 w2401 w2420 w2428 w2435 w2443 w2448 w2453 w2460 w2467 w2473 w2488 w2493 w2506 w2577 w2586 w2597 w2617 w2623 w2629 w2635 w2681 w2697 w2703 w2708 w2714 w2719 w2729 w2737 w2745 w2750 w2755 w2760 w2773 w2786] -> w281
      tunnel: w276 -> [w290 w568 w601 w607 w625 w659 w674 w697 w722 w725 w773 w789 w825 w889 w906 w944 w950 w959 w980 w984 w1011 w1017 w1026 w1032 w1055 w1070 w1079 w1089 w1101 w1117 w1135 w1151 w1165 w1185 w1208 w1226 w1272 w1277 w1283 w1294 w1322 w1348 w1369 w1374 w1382 w1428 w1456 w1470 w1492 w1500 w1513 w1518 w1552 w1578 w1590 w1620 w1633 w1641 w1651 w1662 w1693 w1722 w1735 w1750 w1763 w1777 w1780 w1792 w1797 w1817 w1832 w1849 w1864 w1876 w1881 w1886 w1894 w1907 w1915 w1923 w1931 w1939 w1944 w1949 w1967 w1982 w2001 w2022 w2031 w2040 w2048 w2056 w2061 w2087 w2117 w2160 w2165 w2179 w2195 w2205 w2220 w2245 w2252 w2262 w2274 w2285 w2297 w2308 w2319 w2328 w2338 w2348 w2360 w2367 w2374 w2384 w2401 w2420 w2428 w2435 w2443 w2448 w2453 w2460 w2467 w2473 w2488 w2494 w2507 w2577 w2586 w2609 w2617 w2623 w2629 w2641 w2680 w2697 w2703 w2708 w2714 w2719 w2729 w2737 w2745 w2750 w2755 w2760 w2773 w2786]
      tunnel: [w293 w569 w602 w608 w634 w660 w684 w707 w723 w758 w786 w821 w826 w895 w937 w946 w951 w957 w982 w990 w1013 w1018 w1027 w1033 w1056 w1071 w1083 w1092 w1114 w1123 w1145 w1152 w1166 w1186 w1209 w1235 w1273 w1278 w1284 w1311 w1338 w1365 w1370 w1375 w1393 w1443 w1465 w1481 w1493 w1509 w1514 w1526 w1568 w1579 w1617 w1628 w1634 w1645 w1657 w1688 w1719 w1732 w1745 w1759 w1773 w1778 w1787 w1794 w1802 w1827 w1842 w1857 w1872 w1877 w1882 w1891 w1903 w1908 w1916 w1924 w1932 w1940 w1945 w1954 w1971 w1987 w2007 w2028 w2036 w2041 w2049 w2057 w2062 w2088 w2121 w2161 w2177 w2191 w2203 w2213 w2226 w2246 w2256 w2272 w2282 w2292 w2306 w2316 w2326 w2336 w2346 w2356 w2361 w2368 w2375 w2385 w2403 w2421 w2429 w2436 w2444 w2449 w2456 w2462 w2468 w2476 w2489 w2496 w2508 w2578 w2589 w2610 w2618 w2624 w2630 w2645 w2690 w2698 w2704 w2709 w2715 w2720 w2730 w2738 w2746 w2751 w2756 w2761 w2774 w2787] -> w280
      tunnel: [_ _ _ _ _ _ _ _ _ _ _ _ _ _ _ _ _ _ _ _ TRUE _ _ _ _ _ _ _ _ _ _ _ _ _ _ _ _ _ _ _ _ _ _ _ _ _ _ _ _ _ _ _ _ _ _ _ _ _ _ _ _ _ _ _ _ _ _ _ _ _ _ _ _ _ _ _ _ _ _ _ _ _ _ _ _ _ _ _ _ _ _ _ _ _ _ _ _ _ _ _ _ _ _ _ _ _ _ _ _ _ _ _ _ _ _ _ _ _ _ _ _ _ _ _ _ _ _ _ _ _ _ _ _ _ _ _ _ _ _ _ _ _ _ _ _ _ _ _ _ _] -> w270
      tunnel: [w289 w567 w575 w606 w628 w651 w676 w700 w720 w756 w777 w819 w824 w854 w935 w942 w949 w956 w981 w988 w1012 w1016 w1024 w1031 w1054 w1069 w1075 w1088 w1113 w1122 w1133 w1150 w1156 w1175 w1200 w1229 w1271 w1276 w1282 w1289 w1317 w1343 w1368 w1373 w1387 w1435 w1463 w1468 w1491 w1508 w1512 w1517 w1558 w1577 w1597 w1627 w1632 w1642 w1654 w1672 w1703 w1728 w1741 w1752 w1765 w1776 w1784 w1789 w1800 w1816 w1831 w1847 w1862 w1875 w1880 w1890 w1902 w1906 w1912 w1919 w1929 w1937 w1943 w1953 w1958 w1981 w1990 w2024 w2035 w2039 w2044 w2052 w2060 w2070 w2120 w2158 w2168 w2190 w2202 w2212 w2225 w2243 w2250 w2269 w2281 w2291 w2305 w2315 w2325 w2335 w2345 w2355 w2359 w2366 w2373 w2383 w2402 w2419 w2427 w2434 w2442 w2447 w2455 w2461 w2466 w2475 w2487 w2495 w2505 w2576 w2587 w2596 w2616 w2622 w2628 w2640 w2687 w2696 w2702 w2707 w2713 w2718 w2728 w2736 w2744 w2749 w2754 w2759 w2772 w2785] -> w279
      tunnel: 10 ("Timeout") -> [w288 _ _ _ _ _ _ _ _ _ _ _ _ _ _ _ _ _ _ _ _ _ _ _ _ _ _ _ _ _ _ _ _ _ _ _ _ _ _ _ _ _ _ _ _ _ _ _ _ _ _ _ _ _ _ _ _ _ _ _ _ _ _ _ _ _ _ _ _ _ _ _ _ _ _ _ _ _ _ _ _ _ _ _ _ _ _ _ _ _ _ _ _ _ _ _ _ _ _ _ _ _ _ _ _ _ _ _ _ _ _ _ _ _ _ _ _ _ _ _ _ _ _ _ _ _ _ _ _ _ _ _ _ _ _ _ _ _ _ _ _ _ _ _ _ _ _ _ _ _]
      tunnel: w275 -> [_ _ _ _ w632 _ _ _ _ _ _ _ _ _ _ _ _ _ _ _ _ _ _ _ _ _ _ _ _ _ _ _ _ _ _ _ _ _ _ _ _ _ _ _ _ _ _ _ _ _ _ _ _ _ _ _ _ _ _ _ _ _ _ _ _ _ _ _ _ _ _ _ _ _ _ w1887 w1898 _ _ _ _ _ _ _ _ _ _ _ _ _ _ _ _ _ _ _ _ _ _ _ _ _ _ _ _ _ _ _ _ _ _ _ _ _ _ _ _ _ _ _ _ _ _ _ _ _ _ _ _ _ _ _ _ _ _ _ _ _ _ _ _ _ _ _ _ _ _ _ _ _]
      tunnel: w274 -> [_ _ _ _ w631 _ _ _ _ _ _ _ _ _ _ _ _ _ _ _ _ _ _ _ _ _ _ _ _ _ _ _ _ _ _ _ _ _ _ _ _ _ _ _ _ _ _ _ _ _ _ _ _ _ _ _ _ _ _ _ _ _ _ _ _ _ _ _ _ _ _ _ _ _ _ w1888 w1897 _ _ _ _ _ _ _ _ _ _ _ _ _ _ _ _ _ _ _ _ _ _ _ _ _ _ _ _ _ _ _ _ _ _ _ _ _ _ _ _ _ _ _ _ _ _ _ _ _ _ _ _ _ _ _ _ _ _ _ _ _ _ _ _ _ _ _ _ _ _ _ _ _]
      tunnel: w273 -> [w287 _ _ _ _ _ _ _ _ _ _ _ _ _ _ _ _ _ _ _ _ _ _ _ _ _ _ _ _ _ _ _ _ _ _ _ _ _ _ _ _ _ _ _ _ _ w1459 _ _ _ _ _ _ _ _ _ _ _ _ _ _ _ _ _ _ _ _ _ _ _ _ _ _ _ _ _ _ _ _ _ _ _ _ _ _ _ _ _ _ _ _ _ _ _ _ _ _ _ _ _ _ _ _ _ _ _ _ _ _ _ _ _ _ _ _ _ _ _ _ _ _ _ _ _ _ _ _ _ _ _ _ _ _ _ _ _ _ _ _ _ _ _ _ _ _ _ _ _ _ _]
      tunnel: w272 -> [w286 w566 w586 w605 w633 w658 w683 w706 w721 w757 w785 w820 w823 w894 w936 w941 w948 w953 w968 w987 w1010 w1015 w1025 w1030 w1046 w1068 w1073 w1085 w1100 w1116 w1144 w1149 w1164 w1184 w1207 w1225 w1269 w1275 w1281 w1288 w1316 w1342 w1367 w1372 w1377 w1405 w1464 w1480 w1490 w1495 w1511 w1525 w1567 w1570 w1616 w1619 w1631 w1638 w1647 w1659 w1690 w1721 w1734 w1749 w1762 w1775 w1786 w1793 w1801 w1826 w1841 w1844 w1859 w1874 w1879 w1889 w1896 w1905 w1914 w1922 w1926 w1934 w1942 w1947 w1956 w1976 w1991 w2012 w2030 w2038 w2046 w2054 w2059 w2067 w2119 w2159 w2176 w2189 w2201 w2211 w2224 w2244 w2251 w2271 w2280 w2290 w2304 w2314 w2324 w2334 w2344 w2354 w2358 w2365 w2372 w2382 w2400 w2418 w2426 w2433 w2438 w2446 w2452 w2459 w2465 w2471 w2482 w2491 w2502 w2575 w2588 w2599 w2612 w2620 w2626 w2638 w2689 w2694 w2700 w2706 w2712 w2717 w2727 w2735 w2743 w2748 w2753 w2758 w2771 w2784]
      tunnel: [w285 w566 w586 w605 w633 w658 w683 w706 w721 w757 w785 w820 w823 w894 w936 w941 w948 w953 w968 w987 w1010 w1015 w1025 w1030 w1046 w1068 w1073 w1085 w1100 w1116 w1144 w1149 w1164 w1184 w1207 w1225 w1269 w1275 w1281 w1288 w1316 w1342 w1367 w1372 w1377 w1405 w1464 w1480 w1490 w1495 w1511 w1525 w1567 w1570 w1616 w1619 w1631 w1638 w1647 w1659 w1690 w1721 w1734 w1749 w1762 w1775 w1786 w1793 w1801 w1826 w1841 w1844 w1859 w1874 w1879 w1889 w1896 w1905 w1914 w1922 w1926 w1934 w1942 w1947 w1956 w1976 w1991 w2012 w2030 w2038 w2046 w2054 w2059 w2067 w2119 w2159 w2176 w2189 w2201 w2211 w2224 w2244 w2251 w2271 w2280 w2290 w2304 w2314 w2324 w2334 w2344 w2354 w2358 w2365 w2372 w2382 w2400 w2418 w2426 w2433 w2438 w2446 w2452 w2459 w2465 w2471 w2482 w2491 w2502 w2575 w2588 w2599 w2612 w2620 w2626 w2638 w2689 w2694 w2700 w2706 w2712 w2717 w2727 w2735 w2743 w2748 w2753 w2758 w2771 w2784] -> w271
      tunnel: w267 -> [_ _ _ _ w626 _ _ _ _ _ _ _ _ _ _ _ _ _ _ _ _ _ _ _ _ _ _ _ _ _ _ _ _ _ _ _ _ _ _ _ _ _ _ _ _ _ _ _ _ _ _ _ _ _ _ _ _ _ _ _ _ _ _ _ _ _ _ _ _ _ _ _ _ _ _ _ w1895 _ _ _ _ _ _ _ _ _ _ _ _ _ _ _ _ _ _ _ _ _ _ _ _ _ _ _ _ _ _ _ _ _ _ _ _ _ _ _ _ _ _ _ _ _ _ _ _ _ _ _ _ _ _ _ _ _ _ _ _ _ _ _ _ _ _ _ _ _ _ _ _ _]
      frame "", "Event Structure", "Idle" {
        # "executes when the state queue is empty"
        n118 = event shown="[13] \"Cali&iRF alignment\": Value Change" {
          selector: w286 -> [_ _ _ _ _ _ _ _ _ _ _ _ _ _ _ _ _ _ _ _ _ _ _ _ _ _ _ _ _ _ _]
          dyn-events: [_ _ _ _ _ _ _ _ _ _ _ _ _ _ _ _ _ _ _ _ _ _ _ _ _ _ _ _ _ _ _] -> w285
          timeout: w288 -> [_ _ _ _ _ _ _ _ _ _ _ _ _ _ _ _ _ _ _ _ _ _ _ _ _ _ _ _ _ _ _]
          tunnel: w294 -> [w298 w304 w320 w323 w332 w338 w346 w356 w363 w385 w399 w413 w417 w424 w437 w442 w447 w452 w455 w461 w471 w478 w486 w502 w514 w521 w525 w529 w536 w544 w560]
          tunnel: [w298 w303 w320 w322 w332 w338 w346 w356 w362 w385 w399 w413 w417 w423 w437 w442 w447 w451 w454 w461 w472 w478 w487 w502 w515 w521 w525 w528 w537 w543 w561] -> w293
          tunnel: w292 -> [w296 w307 w318 w325 w331 w339 w347 w354 w358 w383 w397 w411 w415 w419 w435 w440 w445 w448 w456 w459 w467 w476 w479 w500 w509 w519 w523 w530 w535 w541 w558]
          tunnel: [w297 w300 w319 w326 w330 w337 w345 w355 w364 w384 w398 w412 w416 w425 w436 w441 w446 w450 w457 w460 w468 w477 w485 w501 w510 w520 w524 w531 w538 w542 w559] -> w291
          tunnel: w290 -> [w297 w305 w319 w326 w330 w337 w345 w355 w364 w384 w398 w412 w416 w425 w436 w441 w446 w450 w457 w460 w468 w477 w485 w501 w513 w520 w524 w531 w538 w542 w559]
          tunnel: [w296 w307 w318 w325 w331 w339 w347 w354 w359 w383 w397 w411 w415 w420 w435 w440 w445 w448 w456 w459 w469 w476 w480 w500 w516 w519 w523 w530 w535 w541 w558] -> w289
          tunnel: w287 -> [_ _ _ _ _ _ _ _ _ _ _ _ _ _ _ _ _ _ _ _ _ _ _ _ _ _ _ _ _ _ _]
          event "355nm Laser toggle": Mouse Enter {
            n119 = event-data() -> ()  [unwired: 1 in, 4 out]
            n120 = local write "Help"("Toggle 355nm laser." ("Help")) -> ()
          }
          event "355nm Laser toggle": Value Change {
            n121 = event-data() -> ("NewVal"=w306:bool)  [unwired: 1 in, 5 out]
            n122 = Unbundle By Name(w307) -> ("LJ Pinout.355 PWM"=w311:string)
            n123 = call "LabJack_FGV.vi"("Operation(Read)"=enum16{"Write", "Read"}."Read" ("Operation"), "error in (no error)"=w305) -> ("error out"=w312:errorcluster, "Read data"=w313:i32)  [unwired: 8 in]
            n124 = case shown="False" w306 {
              tunnel: [0.0 ("Value") 1.0 ("Value")] -> w309
              frame False {
              }
              frame True {
              }
            }
            n125 = Concatenate Strings(w311, "_EF_ENABLE" ("string")) -> (w308:string)
            n126 = call <vilib>:"LJM_eWriteName.vi"("Handle In"=w313, "Name"=w308, "Value"=w309, "error in"=w312) -> ("error out"=w301:errorcluster)  [unwired: 10 in, 1 out]
            n127 = call <vilib>:"Add State(s) to Queue__JKI_lib_State_Machine.vi"("State(s) in Front (\"\")"="355 Laser: CheckControllerStatus\n355 Laser: CheckPWMStatus" ("State(s) in Front (\"\")"), "State(s) in (\"\")"=w304) -> ("States Out"=w303:string)  [unwired: 13 in]
            n128 = call <userlib>:"Wait (ms)__ogtk.vi"("error in (no error)"=w301, "milliseconds to wait"=u32 500) -> ("error out"=w300:errorcluster)  [unwired: 8 in, 1 out]
          }
          event "Aiming beam toggle": Mouse Enter {
            n129 = event-data() -> ()  [unwired: 1 in, 4 out]
            n130 = local write "Help"("Toggle aiming beam laser." ("Help")) -> ()
          }
          event "Aiming beam toggle": Value Change {
            n131 = event-data() -> ("NewVal"=w324:bool)  [unwired: 1 in, 5 out]
            n132 = case shown="False" w324 {
              tunnel: ["LabJack: AB_PWM_Stop" ("State(s) in Front (\"\")") "LabJack: AB_PWM_Start" ("State(s) in Front (\"\")")] -> w321
              frame False {
              }
              frame True {
              }
            }
            n133 = call <vilib>:"Add State(s) to Queue__JKI_lib_State_Machine.vi"("State(s) in Front (\"\")"=w321, "State(s) in (\"\")"=w323) -> ("States Out"=w322:string)  [unwired: 13 in]
          }
          event "Auto gain ch1": Value Change {
            n134 = event-data() -> ("NewVal"=w329:bool)  [unwired: 1 in, 5 out]
            n135 = case shown="False" w329 {
              frame False {
                n136 = local read "Gain 1"() -> (w333:dbl)
                n137 = call "V1FGV.vi"("action"=enum16{"write", "read"}."write", "V1 in"=w333) -> ()  [unwired: 8 in, 2 out]
                n138 = property on="Gain 1" class="DigNum (strict)"("DisabledEnum"=T10."Enabled" ("Disabled")) -> ()  [unwired: 2 in, 2 out]
              }
              frame True {
                n139 = property on="Gain 1" class="DigNum (strict)"("DisabledEnum"=T10."Disabled and Grayed Out" ("Disabled")) -> ()  [unwired: 2 in, 2 out]
              }
            }
          }
          event "Auto gain ch2": Value Change {
            n140 = event-data() -> ("NewVal"=w340:bool)  [unwired: 1 in, 5 out]
            n141 = case shown="False" w340 {
              frame False {
                n142 = local read "Gain 2"() -> (w341:dbl)
                n143 = property on="Gain 2" class="DigNum (strict)"("DisabledEnum"=T10."Enabled" ("Disabled")) -> ()  [unwired: 2 in, 2 out]
                n144 = call "V2FGV.vi"("action"=enum16{"write", "read"}."write", "V2 in"=w341) -> ()  [unwired: 8 in, 2 out]
              }
              frame True {
                n145 = property on="Gain 2" class="DigNum (strict)"("DisabledEnum"=T10."Disabled and Grayed Out" ("Disabled")) -> ()  [unwired: 2 in, 2 out]
              }
            }
          }
          event "Auto gain ch3": Value Change {
            n146 = event-data() -> ("NewVal"=w348:bool)  [unwired: 1 in, 5 out]
            n147 = case shown="False" w348 {
              frame False {
                n148 = local read "Gain 3"() -> (w349:dbl)
                n149 = property on="Gain 3" class="DigNum (strict)"("DisabledEnum"=T10."Enabled" ("Disabled")) -> ()  [unwired: 2 in, 2 out]
                n150 = call "V3FGV.vi"("action"=enum16{"write", "read"}."write", "V3 in"=w349) -> ()  [unwired: 8 in, 2 out]
              }
              frame True {
                n151 = property on="Gain 3" class="DigNum (strict)"("DisabledEnum"=T10."Disabled and Grayed Out" ("Disabled")) -> ()  [unwired: 2 in, 2 out]
              }
            }
          }
          event "Background": Mouse Enter {
            n152 = event-data() -> ()  [unwired: 1 in, 4 out]
            n153 = local write "Help"("Click to record a background. Currently unimplemented." ("Help")) -> ()
          }
          event "Background": Value Change {
            n154 = event-data() -> ("NewVal"=w360:bool)  [unwired: 1 in, 5 out]
            n155 = case shown="False" w360 {
              tunnel: ["UI: Cursor Set >> Busy\nUtility: SetAllChanManualGain\nQueue: Flash\nUtility: Dewelling >> 2500\nUtility: SetAllChanAutoGain\nUI: Cursor Set >> Idle\nUI: Update\nUI: WFAutoScale >> F\nLabJack: ZeroV\nLabJack: 355_PWM_Stop\nLabJack: AB_PWM_Stop\nUtility: Dewelling >> 10\nDigitizer: Abort\nUtility: RestoreDeConChan\nData: parseDataMacro\nData: saveBG\nRun: BGIncrement\nData: showBG\nUI: Update\nUI: ReadyForAquisition" "UI: Update\nUtility: SaveDeconChan\nLabJack: 355_PWM_Start\n/*LabJack: AB_PWM_Start\nDigitizer: Start\nLED: Red\nUI: duringBGAcquire\nUI: WFAutoScale >>T"] -> w361
              tunnel: [FALSE TRUE] -> w357
              frame False {
                n156 = property on="Background" class="Bool (strict)"("BoolText.Text"="Done!" ("Boolean Text.Text")) -> ()  [unwired: 2 in, 2 out]
              }
              frame True {
                n157 = property on="Background" class="Bool (strict)"("BoolText.Text"="Running" ("Boolean Text.Text"), "Colors [4]"=cluster{u32, u32}[] [{6618880, 6618880}, {16711680, 16711680}]) -> ()  [unwired: 2 in, 2 out]
              }
            }
            n158 = Bundle By Name(cluster=w358, "SysRunning?"=w357) -> (w359:T16)
            n159 = call <vilib>:"Add State(s) to Queue__JKI_lib_State_Machine.vi"("State(s) in Front (\"\")"=w361, "State(s) in (\"\")"=w363) -> ("States Out"=w362:string)  [unwired: 13 in]
          }
          event "Channel 1": Cursor Move {
            n160 = event-data() -> ("CursIdx"=w374:i32, "CursLoc"=w381:cluster{"X":dbl, "Y":dbl})  [unwired: 1 in, 7 out]
            n161 = Unbundle By Name(w381) -> ("X"=w379:dbl)
            n162 = property on="Channel 2" class="WFGraph (strict)"() -> ("CrsrList"=w378:T17)  [unwired: 2 in, 2 out]
            n163 = property on="Channel 3" class="WFGraph (strict)"() -> ("CrsrList"=w375:T17)  [unwired: 2 in, 2 out]
            n164 = Index Array(array=w378, index=w374) -> (element=w382:T18)
            n165 = Index Array(array=w375, index=w374) -> (element=w380:T18)
            n166 = Bundle By Name(cluster=w380, "Position.X"=w379) -> (w373:T18)
            n167 = Bundle By Name(cluster=w382, "Position.X"=w379) -> (w377:T18)
            n168 = Replace Array Subset(array=w378, new element=w377, index=w374) -> (w376:T17)
            n169 = Replace Array Subset(array=w375, new element=w373, index=w374) -> (w372:T17)
            n170 = property on="Channel 2" class="WFGraph (strict)"("CrsrList"=w376) -> ()  [unwired: 2 in, 2 out]
            n171 = property on="Channel 3" class="WFGraph (strict)"("CrsrList"=w372) -> ()  [unwired: 2 in, 2 out]
          }
          event "Channel 2": Cursor Move {
            n172 = event-data() -> ("CursIdx"=w390:i32, "CursLoc"=w396:cluster{"X":dbl, "Y":dbl})  [unwired: 1 in, 7 out]
            n173 = property on="Channel 1" class="WFGraph (strict)"() -> ("CrsrList"=w388:T17)  [unwired: 2 in, 2 out]
            n174 = Unbundle By Name(w396) -> ("X"=w393:dbl)
            n175 = property on="Channel 3" class="WFGraph (strict)"() -> ("CrsrList"=w391:T17)  [unwired: 2 in, 2 out]
            n176 = Index Array(array=w388, index=w390) -> (element=w395:T18)
            n177 = Index Array(array=w391, index=w390) -> (element=w394:T18)
            n178 = Bundle By Name(cluster=w395, "Position.X"=w393) -> (w392:T18)
            n179 = Bundle By Name(cluster=w394, "Position.X"=w393) -> (w389:T18)
            n180 = Replace Array Subset(array=w388, new element=w392, index=w390) -> (w387:T17)
            n181 = Replace Array Subset(array=w391, new element=w389, index=w390) -> (w386:T17)
            n182 = property on="Channel 1" class="WFGraph (strict)"("CrsrList"=w387) -> ()  [unwired: 2 in, 2 out]
            n183 = property on="Channel 3" class="WFGraph (strict)"("CrsrList"=w386) -> ()  [unwired: 2 in, 2 out]
          }
          event "Channel 3": Cursor Move {
            n184 = event-data() -> ("CursIdx"=w403:i32, "CursLoc"=w410:cluster{"X":dbl, "Y":dbl})  [unwired: 1 in, 7 out]
            n185 = Unbundle By Name(w410) -> ("X"=w407:dbl)
            n186 = property on="Channel 1" class="WFGraph (strict)"() -> ("CrsrList"=w406:T17)  [unwired: 2 in, 2 out]
            n187 = property on="Channel 2" class="WFGraph (strict)"() -> ("CrsrList"=w404:T17)  [unwired: 2 in, 2 out]
            n188 = Index Array(array=w406, index=w403) -> (element=w409:T18)
            n189 = Index Array(array=w404, index=w403) -> (element=w408:T18)
            n190 = Bundle By Name(cluster=w409, "Position.X"=w407) -> (w405:T18)
            n191 = Bundle By Name(cluster=w408, "Position.X"=w407) -> (w402:T18)
            n192 = Replace Array Subset(array=w406, new element=w405, index=w403) -> (w401:T17)
            n193 = Replace Array Subset(array=w404, new element=w402, index=w403) -> (w400:T17)
            n194 = property on="Channel 1" class="WFGraph (strict)"("CrsrList"=w401) -> ()  [unwired: 2 in, 2 out]
            n195 = property on="Channel 2" class="WFGraph (strict)"("CrsrList"=w400) -> ()  [unwired: 2 in, 2 out]
          }
          event "Cali&iRF alignment": Mouse Enter {
            n196 = event-data() -> ()  [unwired: 1 in, 4 out]
            n197 = local write "Help"("Click to run system intensity calibration and irf alignment" ("Help")) -> ()
          }
          event "Cali&iRF alignment": Value Change {
            n198 = event-data() -> ("NewVal"=w421:bool)  [unwired: 1 in, 5 out]
            n199 = case shown="False" w421 {
              tunnel: ["UI: Cursor Set >> Busy\nUtility: SetAllChanManualGain\nQueue: Flash\nUtility: Dewelling >> 1500\nUtility: SetAllChanAutoGain\nUI: Cursor Set >> Idle\nUI: Update\nLabJack: ZeroV\nLabJack: 355_PWM_Stop\nLabJack: AB_PWM_Stop\nUtility: Dewelling >> 10\nDigitizer: Abort\nUtility: RestoreDeConChan\nData: parseRunData\nData: irfAlignment\nUI: Update\nUI: ReadyForAquisition" "UI: Update\nUtility: SaveDeconChan\nLabJack: 355_PWM_Start\n/*LabJack: AB_PWM_Start\nDigitizer: Start\nLED: Red\nUI: duringIRFAlign"] -> w422
              tunnel: [FALSE TRUE] -> w418
              frame False {
                n200 = property on="Cali&iRF alignment" class="Bool (strict)"("BoolText.Text"="Done!" ("Boolean Text.Text")) -> ()  [unwired: 2 in, 2 out]
              }
              frame True {
                n201 = property on="Cali&iRF alignment" class="Bool (strict)"("BoolText.Text"="Running" ("Boolean Text.Text"), "Colors [4]"=cluster{u32, u32}[] [{6618880, 6618880}, {16711680, 16711680}]) -> ()  [unwired: 2 in, 2 out]
              }
            }
            n202 = Bundle By Name(cluster=w419, "SysRunning?"=w418) -> (w420:T16)
            n203 = call <vilib>:"Add State(s) to Queue__JKI_lib_State_Machine.vi"("State(s) in Front (\"\")"=w422, "State(s) in (\"\")"=w424) -> ("States Out"=w423:string)  [unwired: 13 in]
          }
          event "Gain 1": Value Change {
            n204 = event-data() -> ()  [unwired: 1 in, 6 out]
            n205 = call "V1FGV.vi"("action"=enum16{"write", "read"}."write", "V1 in"="Gain 1") -> ()  [unwired: 8 in, 2 out]
          }
          event "Gain 2": Value Change {
            n206 = event-data() -> ()  [unwired: 1 in, 6 out]
            n207 = call "V2FGV.vi"("action"=enum16{"write", "read"}."write", "V2 in"="Gain 2") -> ()  [unwired: 8 in, 2 out]
          }
          event "Gain 3": Value Change {
            n208 = event-data() -> ()  [unwired: 1 in, 6 out]
            n209 = call "V3FGV.vi"("action"=enum16{"write", "read"}."write", "V3 in"="Gain 3") -> ()  [unwired: 8 in, 2 out]
          }
          event "Quit": Value Change {
            # "Exit Button Value Change (pressed) Event\n(when pressed.  quite)"
            n210 = event-data() -> ()  [unwired: 1 in, 1 out]
            n211 = call <vilib>:"Add State(s) to Queue__JKI_lib_State_Machine.vi"("State(s) in Front (\"\")"="LED: Off\nMacro: Exit", "State(s) in (\"\")"=w452) -> ("States Out"=w451:string)  [unwired: 13 in]
          }
          event "Show BG": Value Change {
            n212 = event-data() -> ()  [unwired: 1 in, 6 out]
            n213 = call <vilib>:"Add State(s) to Queue__JKI_lib_State_Machine.vi"("State(s) in Front (\"\")"="Data: showBG" ("State(s) in Front (\"\")"), "State(s) in (\"\")"=w455) -> ("States Out"=w454:string)  [unwired: 13 in]
          }
          event "StartButton": Mouse Enter {
            n214 = event-data() -> ()  [unwired: 1 in, 4 out]
            n215 = local write "Help"("Press to start aquisition." ("Help")) -> ()
          }
          event "StartButton": Value Change {
            # "start PWM before acquisition"
            # "Initialize both digitizer aquisition and\n send user event to trigger aquisition loop"
            n216 = event-data() -> ()  [unwired: 1 in, 6 out]
            n217 = Unbundle By Name(w467) -> ("System Status.TCP/IP"=w466:bool)
            n218 = case shown="True" w466 {
              tunnel: ["" "TCP: sendRunNum\nTCP: sendVideoSource\nTCP: startRun"] -> w464
              frame False {
              }
              frame True {
              }
            }
            n219 = local write "StartButton"(FALSE ("StartButton")) -> ()
            n220 = Bundle By Name(cluster=w467, "SysRunning?"=TRUE) -> (w469:T16)
            n221 = call <vilib>:"Add State(s) to Queue__JKI_lib_State_Machine.vi"("State(s) in Front (\"\")"="UI: Update\nLabJack: 355_PWM_Start\nLabJack: AB_PWM_Start\nDigitizer: Start\nUI: DuringAquisition\nLED: Red", "State(s) in (\"\")"=w464) -> ("States Out"=w463:string)  [unwired: 13 in]
            n222 = call <vilib>:"Add State(s) to Queue__JKI_lib_State_Machine.vi"("State(s) in Front (\"\")"=w463, "State(s) in (\"\")"=w471) -> ("States Out"=w472:string)  [unwired: 13 in]
          }
          event "StopButton": Mouse Enter {
            n223 = event-data() -> ()  [unwired: 1 in, 4 out]
            n224 = local write "Help"("Press to stop data aquisition." ("Help")) -> ()
          }
          event "StopButton": Value Change {
            # "if system is running, send stop command, if not do nothing."
            # "stop aquisition\nupdate UI"
            n225 = event-data() -> ()  [unwired: 1 in, 6 out]
            n226 = Unbundle By Name(w479) -> ("SysRunning?"=w481:bool, "System Status.TCP/IP"=w484:bool)
            n227 = case shown="True" w481 {
              tunnel: w484 -> [_ w496]
              tunnel: ["" w495] -> w483
              tunnel: w479 -> [w488 w492]
              tunnel: [w488 w491] -> w480
              frame False {
              }
              frame True {
                n228 = case shown="True" w496 {
                  tunnel: ["" "TCP: stopRun"] -> w494
                  frame False {
                  }
                  frame True {
                  }
                }
                n229 = Bundle By Name(cluster=w492, "SysRunning?"=FALSE) -> (w491:T16)
                n230 = call <vilib>:"Add State(s) to Queue__JKI_lib_State_Machine.vi"("State(s) in Front (\"\")"=w494, "State(s) in (\"\")"="UI: Cursor Set >> Busy\nUI: Update\nUI: ReadyForAquisition\nLabJack: 355_PWM_Stop\nLabJack: AB_PWM_Stop\nDigitizer: Abort\nData: parseDataMacro\nData: saveRunData\nUI: Cursor Set>>Idle") -> ("States Out"=w495:string)  [unwired: 13 in]
              }
            }
            n231 = local write "StopButton"(FALSE ("StopButton")) -> ()
            n232 = call <vilib>:"Add State(s) to Queue__JKI_lib_State_Machine.vi"("State(s) in Front (\"\")"=w483, "State(s) in (\"\")"=w486) -> ("States Out"=w487:string)  [unwired: 13 in]
          }
          event "Sys Reconfig": Mouse Enter {
            n233 = event-data() -> ()  [unwired: 1 in, 4 out]
            n234 = local write "Help"("Click to reconfig digitizer settings." ("Help")) -> ()
          }
          event "Sys Reconfig": Value Change {
            # "everytime the user change data aquisition setting, need to reinitilize decon engine and realign iRF.\ncheck whether data length has changed, if changed, reinitialize Decon engine\nreset BG ready, need a new BG"
            # "update DAQ FGV"
            n235 = event-data() -> ()  [unwired: 1 in, 6 out]
            n236 = call "SystemConfigEditorV6.vi"("error in"=w513) -> ("error out"=w511:errorcluster, "FLImDAQ out"=w506:T5)  [unwired: 1 in]
            n237 = Unbundle By Name(w509) -> ("FLImDAQ.min record length"=w508:i32)
            n238 = Unbundle By Name(w506) -> ("min record length"=w507:i32)
            n239 = call "FLImDAQ_FGV.vi"(6:enum16{"Write", "Read"}."Write" ("Operation"), "error in (no error)"=w511, "Write data"=w506) -> ("error out"=w510:errorcluster, "Read data"=w505:T5)  [unwired: 7 in]
            n240 = Equal?(x=w508, y=w507) -> (x = y?=w504:bool)
            n241 = case shown="False" w504 {
              tunnel: ["UI: Cursor Set >> Busy\nDigitizer: Config\nDeconEngine: InitializeCh1\nDeconEngine: InitializeCh2\nDeconEngine: InitializeCh3\nUI: CaliAndiRFNotReady\n/*UI iRF not ready\nUI: Update\nUI: Cursor Set >> Idle" "UI: Cursor Set >> Busy\nDigitizer: Config\nUI: Update\nUI: Cursor Set >> Idle"] -> w503
              frame False {
              }
              frame True {
              }
            }
            n242 = Bundle By Name(cluster=w509, "FLImDAQ"=w505) -> (w516:T16)
            n243 = call <vilib>:"Add State(s) to Queue__JKI_lib_State_Machine.vi"("State(s) in Front (\"\")"=w503, "State(s) in (\"\")"=w514) -> ("States Out"=w515:string)  [unwired: 13 in]
          }
          event "System Hardware Connection Status", "StartButton", "StopButton", "355nm Laser toggle", "Aiming beam toggle", "Cali&iRF alignment", "Background", "Sys Reconfig": Mouse Leave {
            n244 = event-data() -> ()  [unwired: 1 in, 4 out]
            n245 = invoke on="Help" class="Str" method="Reinit To Default"() -> ()  [unwired: 3 in, 3 out]
          }
          event "System Hardware Connection Status.Digitizer": Mouse Enter {
            n246 = event-data() -> ()  [unwired: 1 in, 4 out]
            n247 = local write "Help"("Status of hardware connections. TCP/IP is optional." ("Help")) -> ()
          }
          event "TCP Connect": Value Change {
            n248 = event-data() -> ("NewVal"=w526:bool)  [unwired: 1 in, 5 out]
            n249 = case shown="False" w526 {
              tunnel: ["TCP: Close\nUI: Update" ("State(s) in Front (\"\")") "TCP: Initialize\nTCP: SendSettingMacro\nUI: Update" ("State(s) in Front (\"\")")] -> w527
              frame False {
              }
              frame True {
              }
            }
            n250 = call <vilib>:"Add State(s) to Queue__JKI_lib_State_Machine.vi"("State(s) in Front (\"\")"=w527, "State(s) in (\"\")"=w529) -> ("States Out"=w528:string)  [unwired: 13 in]
          }
          event User Event {
            # "if aquisition loop is error out. Stop digitizer, update front panel indicator, stop both laser and parse and save data"
            n251 = event-data() -> ()  [unwired: 1 in, 5 out]
            n252 = property on="StopButton" class="Bool (strict)"("Val(Sgnl)"=TRUE ("Value (Signaling)")) -> ()  [unwired: 2 in, 2 out]
            n253 = call <vilib>:"Add State(s) to Queue__JKI_lib_State_Machine.vi"("State(s) in (\"\")"=w536) -> ("States Out"=w537:string)  [unwired: 14 in]
          }
          event Panel Close? {
            # "Discard the event because we'll close the front panel ourselves in Macro: Exit"
            # "Close Panel button (pressed) Event\n(this executes Macro: Exit to terminate the VI)"
            n254 = event-data() -> ()  [unwired: 1 in, 1 out]
            n255 = event-data("Discard?"=TRUE) -> ()  [unwired: 1 in, 1 out]
            n256 = call <vilib>:"Add State(s) to Queue__JKI_lib_State_Machine.vi"("State(s) in Front (\"\")"="Macro: Exit", "State(s) in (\"\")"=w544) -> ("States Out"=w543:string)  [unwired: 13 in]
          }
          event Timeout {
            # "check system status every 2s"
            n257 = event-data() -> ()  [unwired: 1 in, 1 out]
            n258 = Unbundle By Name(w558) -> ("SlowTimer"=w557:u32, "FastTimer"=w545:u32)
            n259 = Tick Count (ms)() -> (millisecond timer value=w546:u32)
            n260 = Subtract(x=w546, y=w557) -> (x-y=w551:u32)
            n261 = Subtract(x=w546, y=w545) -> (x-y=w547:u32)
            n262 = Greater?(x=w551, y=u32 2000) -> (0:w552:bool)
            n263 = Greater?(x=w547, y=u32 100) -> (0:w549:bool)
            n264 = case shown="True" w552 {
              tunnel: ["" "SystemStatus: SlowSysStatusMacro" ("State(s) in Front (\"\")")] -> w553
              frame False {
              }
              frame True {
              }
            }
            n265 = case shown="True" w549 {
              tunnel: ["" "SystemStatus: FastSysStatusMacro" ("State(s) in Front (\"\")")] -> w548
              frame False {
              }
              frame True {
              }
            }
            n266 = call <vilib>:"Add State(s) to Queue__JKI_lib_State_Machine.vi"("State(s) in Front (\"\")"="LabJack: checkPedal" ("State(s) in Front (\"\")"), "State(s) in (\"\")"=w553, "State(s) at Back (\"\")"=w548) -> ("States Out"=w555:string)  [unwired: 12 in]
            n267 = call <vilib>:"Add State(s) to Queue__JKI_lib_State_Machine.vi"("State(s) in Front (\"\")"=w555, "State(s) in (\"\")"=w560) -> ("States Out"=w561:string)  [unwired: 13 in]
          }
        }
      }
      frame "---------- Data ----------" {
        # "Do not put any code in this frame.\n(It is a separator no-op. You can make a copy of this frame to create a new Data frame)"
        n268 = call <vilib>:"Add State(s) to Queue__JKI_lib_State_Machine.vi"("State(s) in (\"\")"=w570) -> ("States Out"=w569:string)  [unwired: 14 in]
      }
      frame "Data: Initialize" {
        w571 = cluster{"RunID":i8, "BG ID":i8, "Cali ID":i8} {"RunID"=1, "BG ID"=1, "Cali ID"=1}  # IDs
        w572 = refnum<vi> refnum  # LED vi reference
        w573 = path ""  # TempPath
        w574 = T19 {"DataPath"=path "", "BG Path"=path "", "iRFPath"=path "", "CaliPath"=path ""}  # Pathes
        w576 = dbl[] []  # V3
        w577 = dbl[] []  # V2
        w578 = dbl[] []  # V1
        w580 = u32 0  # FastTimer
        w581 = u32 0  # SlowTimer
        w582 = dbl[][] []  # Ch3Data
        w583 = dbl[][] []  # Ch2Data
        w584 = dbl[][] []  # Ch1Data
        w587 = T1 {"Digitizer"=FALSE, "Labjack"=FALSE, "Aiming Beam"=FALSE, "355 Laser"=FALSE, "TCP/IP"=FALSE}  # System Status
        w588 = T20 {"DIO_EF_CLOCK1_DIVISOR"=16, "DIO_EF_CLOCK1_ROLL_VALUE"=25000, "DIO#_EF_INDEX"=0, "DIO#_EF_OPTIONS"=1, "DIO#_EF_CONFIG_A"=6250}  # AB PWM setting
        w589 = T4 {"Ch1 Bias"="TDA11", "Ch2 Bias"="DAC10", "Ch3 Bias"="DAC0", "355 PWM"="FIO0", "AimingBeam PWM"="FIO2", "Laser Ready"="FIO3", "Interlock"="FIO1", "Laser Start/Stop"="FIO1", "Red LED"="FIO1", "Green LED"="FIO1", "Foot Pedal"="DIO15"}  # LJ Pinout
        w590 = 0  # TCP attempt count
        w591 = u32 0  # Laser start tic
        w592 = refnum<k20>[] []  # niTClk sessions
        w593 = u32 0  # Last Trigger
        w594 = T20 {"DIO_EF_CLOCK1_DIVISOR"=16, "DIO_EF_CLOCK1_ROLL_VALUE"=25000, "DIO#_EF_INDEX"=0, "DIO#_EF_OPTIONS"=1, "DIO#_EF_CONFIG_A"=6250}  # 355 PWM setting
        w595 = T21 {"Aiming Beam COM Port"="COM3", "Min Current"=0.0, "Max Current"=63.0, "Default Current"=20.0, 0}  # AB Cluster
        w596 = T22 {"resource name"="", "resource name 2"="", "Channel"=enum."Channel 0", "trigger source"="VAL_EXTERNAL", "trigger level"=0.5, "trigger delay"=1.35e-07, "min sample rate"=12500000000.0, "min record length"=2500, "vertical range"=1.0, "vertical offset"=-0.25, "Waveform to Avg"=2000}  # FLImDAQ
        w597 = FALSE  # SysRunning?
        w585 = path ""  # DefaultPath
        w598 = ""  # CaseID
        w599 = T3 {"Ch1Enable?"=FALSE, "Ch2Enable?"=FALSE, "Ch3Enable?"=FALSE, "Ch1AutoGain?"=FALSE, "Ch2AutoGain?"=FALSE, "Ch3AutoGain?"=FALSE, "AimingBeamEnable?"=FALSE}  # SysConfigCluster
        w600 = T23 {"Current VI Reference"=refnum, "Close Panel on Exit?"=FALSE}  # Core
        # "Initialize the shift-register data, here.\n(data names are defined by what you wire into the bundle function)"
        n269 = Bundle("Core"=w600, "SysConfigCluster"=w599, "System Status"=w587, "IDs"=w571, "CaseID"=w598, "DefaultPath"=w585, "Pathes"=w574, "FLImDAQ"=w596, "SysRunning?"=w597, "AB Cluster"=w595, "LJ Pinout"=w589, "355 PWM setting"=w594, "AB PWM setting"=w588, "Last Trigger"=w593, "niTClk sessions"=w592, "Laser start tic"=w591, "TCP attempt count"=w590, "Ch1Data"=w584, "Ch2Data"=w583, "Ch3Data"=w582, "V1"=w578, "V2"=w577, "V3"=w576, "SlowTimer"=w581, "FastTimer"=w580, "listener ID"=refnum<k5> refnum, "TempPath"=w573, "LED vi reference"=w572) -> (w575:T16)  [unwired: 1 in]
        n270 = call <vilib>:"Add State(s) to Queue__JKI_lib_State_Machine.vi"("State(s) in (\"\")"=w603) -> ("States Out"=w602:string)  [unwired: 14 in]
      }
      frame "Data: parseDataMacro" {
        # "Sometimes it takes some time to parse run data"
        # "Parse data macro.\n(Set curse busy, parse data, then set cursor idle)"
        n271 = call <vilib>:"Add State(s) to Queue__JKI_lib_State_Machine.vi"("State(s) in Front (\"\")"="UI: Cursor Set >> Busy\nData: parseRunData\nUI: Cursor Set >> Idle" ("State(s) in Front (\"\")"), "State(s) in (\"\")"=w609) -> ("States Out"=w608:string)  [unwired: 13 in]
      }
      frame "Data: parseRunData" {
        # "flash queue"
        # "Ch3&4"
        # "Ch1&2"
        # "Flash data from queue and save it in structure\n()"
        n272 = Flush Queue(queue=w632, error in (no error)=w625) -> (remaining elements=w630:cluster{"double data":dbl[][]}[], error out=w623:errorcluster)  [unwired: 1 out]
        n273 = Flush Queue(queue=w626, error in (no error)=w625) -> (remaining elements=w620:cluster{"V1":dbl, "V2":dbl, "V3":dbl}[], error out=w621:errorcluster)  [unwired: 1 out]
        n274 = Flush Queue(queue=w631, error in (no error)=w625) -> (remaining elements=w629:cluster{"double data":dbl[][]}[], error out=w622:errorcluster)  [unwired: 1 out]
        n275 = for {
          tunnel: w629 -> [w642] mode=indexing
          tunnel: [w641] -> w610 mode=concatenating
          n276 = Unbundle By Name(w642) -> ("double data"=w640:dbl[][])
          n277 = call "SeperateChanData.vi"("Input (Ch1&2)"=w640) -> ("Ch1"=w641:dbl[][])  [unwired: 1 out]
        }
        n278 = for {
          tunnel: w620 -> [w639] mode=indexing
          tunnel: [w638] -> w615 mode=indexing
          tunnel: [w637] -> w614 mode=indexing
          tunnel: [w636] -> w613 mode=indexing
          n279 = Unbundle By Name(w639) -> ("V1"=w638:dbl, "V2"=w637:dbl, "V3"=w636:dbl)
        }
        "V1" <- w615
        "V2" <- w614
        "V3" <- w613
        n280 = for {
          tunnel: w630 -> [w646] mode=indexing
          tunnel: [w644] -> w612 mode=concatenating
          tunnel: [w643] -> w611 mode=concatenating
          n281 = Unbundle By Name(w646) -> ("double data"=w645:dbl[][])
          n282 = call "SeperateChanData.vi"("Input (Ch1&2)"=w645) -> ("Ch1"=w644:dbl[][], "Ch2"=w643:dbl[][])
        }
        n283 = Array Size(array=w615) -> (size(s)=→"V1 Size":i32)
        n284 = Array Size(array=w614) -> (size(s)=→"V2 Size":i32)
        n285 = Array Size(array=w613) -> (size(s)=→"V3 Size":i32)
        n286 = Bundle By Name(cluster=w627, "Ch1Data"=w612, "Ch2Data"=w611, "Ch3Data"=w610, "V1"=w615, "V2"=w614, "V3"=w613) -> (w628:T16)
        n287 = Array Size(array=w610) -> (size(s)=→"data Size":i32[])
        n288 = Merge Errors(w623, w622, w621) -> (w624:errorcluster)
        n289 = call <vilib>:"Add State(s) to Queue__JKI_lib_State_Machine.vi"("State(s) in (\"\")"=w635) -> ("States Out"=w634:string)  [unwired: 14 in]
      }
      frame "Data: loadLastUseiRF" {
        # "Load last use iRF.\n()"
        n290 = Unbundle By Name(w651) -> ("TempPath"=w650:path)
        n291 = Build Path(base path=w650, name or relative path="iRF.tdms") -> (appended path=w656:path)
        n292 = TDMS Open(11:w656) -> (0:w654:errorcluster, 3:w655:refnum<k34>)  [unwired: 6 in]
        n293 = TDMS Read(0:w655, 11:w654, 12:dbl[][] []) -> (4:w648:refnum<k34>, 10:w652:dbl[][], 15:w647:errorcluster)  [unwired: 5 in, 3 out]
        n294 = case shown="No Error" w647 {
          tunnel: w652 -> [w664 _]
          tunnel: ["UI: CaliAndiRFLoaded" ("State(s) in Front (\"\")") ""] -> w649
          frame No Error {
            n295 = Index Array(array=w664, index (row)=0) -> (element=w667:dbl[])  [unwired: 1 in]
            n296 = Index Array(array=w664, index (row)=1) -> (element=w666:dbl[])  [unwired: 1 in]
            n297 = Index Array(array=w664, index (row)=2) -> (element=w665:dbl[])  [unwired: 1 in]
            n298 = Bundle(w667, w666, w665) -> (w663:cluster{dbl[], dbl[], dbl[]})  [unwired: 1 in]
            n299 = global write "GlobalVariables.vi" "LastUseiRF"(w663) -> ()
          }
          frame Error {
          }
        }
        n300 = TDMS Close(8:w647, 11:w648) -> ()  [unwired: 2 out]
        n301 = call <vilib>:"Add State(s) to Queue__JKI_lib_State_Machine.vi"("State(s) in Front (\"\")"=w649, "State(s) in (\"\")"=w661) -> ("States Out"=w660:string)  [unwired: 13 in]
      }
      frame "Data: loadLastUseCali" {
        # "Load last use calibration.\n()"
        n302 = Unbundle By Name(w676) -> ("TempPath"=w675:path)
        n303 = Build Path(base path=w675, name or relative path="Calibration.tdms") -> (appended path=w681:path)
        n304 = TDMS Open(11:w681) -> (0:w679:errorcluster, 3:w680:refnum<k34>)  [unwired: 6 in]
        n305 = TDMS Read(0:w680, 11:w679, 12:dbl[][] []) -> (4:w672:refnum<k34>, 10:w677:dbl[][], 15:w673:errorcluster)  [unwired: 5 in, 3 out]
        n306 = TDMS Close(8:w673, 11:w672) -> ()  [unwired: 2 out]
        n307 = case shown="Error .." w673 {
          tunnel: w677 -> [w690 _]
          frame No Error {
            n308 = Index Array(array=w690, index (row)=0) -> (element=w689:dbl[])  [unwired: 1 in]
            n309 = Index Array(array=w690, index (row)=1) -> (element=w688:dbl[])  [unwired: 1 in]
            n310 = Index Array(array=w690, index (row)=2) -> (element=w686:dbl[])  [unwired: 1 in]
            n311 = Bundle(w689, w688, w686) -> (w687:cluster{dbl[], dbl[], dbl[]})  [unwired: 1 in]
            n312 = global write "GlobalVariables.vi" "LastUseCaliData"(w687) -> ()
          }
          frame Error {
          }
        }
        n313 = call <vilib>:"Add State(s) to Queue__JKI_lib_State_Machine.vi"("State(s) in (\"\")"=w685) -> ("States Out"=w684:string)  [unwired: 14 in]
      }
      frame "Data: loadLastUseBG" {
        # "check data size here. If not the same as current setting, return error."
        # "Load last use BG.\n()"
        n314 = Unbundle By Name(w700) -> ("TempPath"=w699:path)
        n315 = Build Path(base path=w699, name or relative path="Background.tdms") -> (appended path=w704:path)
        n316 = TDMS Open(11:w704) -> (0:w702:errorcluster, 3:w703:refnum<k34>)  [unwired: 6 in]
        n317 = TDMS Read(0:w703, 11:w702, 12:dbl[][] []) -> (4:w695:refnum<k34>, 10:w698:dbl[][], 15:w694:errorcluster)  [unwired: 5 in, 3 out]
        n318 = TDMS Close(8:w694, 11:w695) -> ()  [unwired: 2 out]
        n319 = case shown="Error .." w694 {
          tunnel: w698 -> [w710 _]
          tunnel: ["UI: BGLoaded" ("State(s) in Front (\"\")") ""] -> w696
          frame No Error {
            w711 = enum16{"write", "read"}."write" ("action")
            # "If no error, check size match"
            n320 = Index Array(array=w710, index (row)=0) -> (element=w714:dbl[])  [unwired: 1 in]
            n321 = Index Array(array=w710, index (row)=1) -> (element=w713:dbl[])  [unwired: 1 in]
            n322 = Index Array(array=w710, index (row)=2) -> (element=w712:dbl[])  [unwired: 1 in]
            n323 = call "BG3FGV.vi"("action"=w711, "BG1 in"=w712) -> ()  [unwired: 8 in, 2 out]
            n324 = call "BG1FGV.vi"("action"=w711, "BG1 in"=w714) -> ()  [unwired: 8 in, 2 out]
            n325 = call "BG2FGV.vi"("action"=w711, "BG1 in"=w713) -> ()  [unwired: 8 in, 2 out]
          }
          frame Error {
            # "If error set BG all 0, update UI"
          }
        }
        n326 = call <vilib>:"Add State(s) to Queue__JKI_lib_State_Machine.vi"("State(s) in Front (\"\")"=w696, "State(s) in (\"\")"=w708) -> ("States Out"=w707:string)  [unwired: 13 in]
      }
      frame "Data: loadLastUseMacro" {
        # "Load last use BG and Cali and iRF.\n(It is a separator no-op. You can make a copy of this frame to create a new Data frame)"
        n327 = call <vilib>:"Add State(s) to Queue__JKI_lib_State_Machine.vi"("State(s) in Front (\"\")"="Data: loadLastUseBG\nData: loadLastUseCali\nData: loadLastUseiRF" ("State(s) in Front (\"\")"), "State(s) in (\"\")"=w724) -> ("States Out"=w723:string)  [unwired: 13 in]
      }
      frame "Data: saveCalibration" {
        w736 = T11."create or replace" ("operation (0:open)")
        w741 = string[] ["Ch1", "Ch2", "Ch3"] ("channel name(s) in (Untitled)")
        w740 = "Calibration" ("group name in (Untitled)")
        w726 = "Calibration" ("default name")
        # "Average data and save calibration file\n(It is a separator no-op. You can make a copy of this frame to create a new Data frame)"
        n328 = Unbundle By Name(w756) -> ("Ch1Data"=w755:dbl[][], "Ch2Data"=w754:dbl[][], "Ch3Data"=w753:dbl[][], "Pathes.CaliPath"=w728:path, "TempPath"=w748:path, "IDs.Cali ID"=w727:i8)
        n329 = Build Path(base path=w748, name or relative path=w726) -> (appended path=w745:path)
        n330 = Format Value(string ("")=w726, format string="%02d", value (0)=w727) -> (output string=w731:string)
        n331 = call "AvgArray.vi"("2D array"=w755) -> ("1D Avg"=w735:dbl[])  [unwired: 10 in]
        n332 = call "AvgArray.vi"("2D array"=w754) -> ("1D Avg"=w734:dbl[])  [unwired: 10 in]
        n333 = call "AvgArray.vi"("2D array"=w753) -> ("1D Avg"=w733:dbl[])  [unwired: 10 in]
        n334 = Build Path(base path=w728, name or relative path=w731) -> (appended path=w729:path)
        n335 = TDMS Open(8:w725, 10:w736, 11:w745) -> (0:w747:errorcluster, 3:w744:refnum<k34>)  [unwired: 4 in]
        n336 = TDMS Open(8:w725, 10:w736, 11:w729) -> (0:w751:errorcluster, 3:w752:refnum<k34>)  [unwired: 4 in]
        n337 = Build Array(w735, w734, w733) -> (w742:dbl[][])
        n338 = Bundle("1D Avg"=w735, "1D Avg"=w734, "1D Avg"=w733) -> (w732:T24)  [unwired: 1 in]
        n339 = TDMS Write(0:w744, 5:w740, 7:w741, 9:w742, 11:w747) -> (4:w743:refnum<k34>, 15:w746:errorcluster)  [unwired: 1 in, 2 out]
        n340 = TDMS Write(0:w752, 5:w740, 7:w741, 9:w742, 11:w751) -> (4:w750:refnum<k34>, 15:w749:errorcluster)  [unwired: 1 in, 2 out]
        n341 = global write "GlobalVariables.vi" "LastUseCaliData"(w732) -> ()
        n342 = TDMS Close(8:w746, 11:w743) -> (0:w738:errorcluster)  [unwired: 1 out]
        n343 = TDMS Close(8:w749, 11:w750) -> (0:w739:errorcluster)  [unwired: 1 out]
        n344 = Merge Errors(w739, w738) -> (w737:errorcluster)
        n345 = call <vilib>:"Add State(s) to Queue__JKI_lib_State_Machine.vi"("State(s) in (\"\")"=w759) -> ("States Out"=w758:string)  [unwired: 14 in]
      }
      frame "Data: saveiRF" {
        w784 = enum16{"write", "read"}."read" ("action")
        # "Get iRF from decon stracture and save it on disk.\n(It is a separator no-op. You can make a copy of this frame to create a new Data frame)"
        n346 = Unbundle By Name(w777) -> ("TempPath"=w776:path)
        n347 = call "Ch1DeconEngineFGV.vi"("action"=w784) -> ("Error Out"=w782:errorcluster, "Ch1DeconEngine out"=w783:refnum<class "LaguerreDeconEngineClass.lvclass">)  [unwired: 9 in]
        n348 = call "Ch2DeconEngineFGV.vi"("action"=w784) -> ("Error Out"=w780:errorcluster, "Ch2DeconEngine out"=w781:refnum<class "LaguerreDeconEngineClass.lvclass">)  [unwired: 9 in]
        n349 = call "Ch3DeconEngineFGV.vi"("action"=w784) -> ("Error Out"=w778:errorcluster, "Ch3DeconEngine out"=w779:refnum<class "LaguerreDeconEngineClass.lvclass">)  [unwired: 9 in]
        n350 = Build Path(base path=w776, name or relative path="iRF" ("default name")) -> (appended path=w774:path)
        n351 = call "getIRF.vi"("error in (no error)"=w782, "LaguerreDeconEngineClass in"=w783) -> ("iRF"=w763:dbl[])  [unwired: 7 in, 2 out]
        n352 = call "getIRF.vi"("error in (no error)"=w780, "LaguerreDeconEngineClass in"=w781) -> ("iRF"=w762:dbl[])  [unwired: 7 in, 2 out]
        n353 = call "getIRF.vi"("error in (no error)"=w778, "LaguerreDeconEngineClass in"=w779) -> ("iRF"=w761:dbl[])  [unwired: 7 in, 2 out]
        n354 = Build Array(w763, w762, w761) -> (w769:dbl[][])
        n355 = TDMS Open(8:w773, 10:T11."create or replace" ("operation (0:open)"), 11:w774) -> (0:w770:errorcluster, 3:w771:refnum<k34>)  [unwired: 4 in]
        n356 = Bundle("iRF"=w763, "iRF"=w762, "iRF"=w761) -> (w760:cluster{"iRF":dbl[], "iRF":dbl[], "iRF":dbl[]})  [unwired: 1 in]
        n357 = global write "GlobalVariables.vi" "LastUseiRF"(w760) -> ()
        n358 = TDMS Write(0:w771, 5:"iRF" ("group name in (Untitled)"), 7:string[] ["Ch1", "Ch2", "Ch3"] ("channel name(s) in (Untitled)"), 9:w769, 11:w770) -> (4:w766:refnum<k34>, 15:w765:errorcluster)  [unwired: 1 in, 2 out]
        n359 = TDMS Close(8:w765, 11:w766) -> (0:w764:errorcluster)  [unwired: 1 out]
        n360 = call <vilib>:"Add State(s) to Queue__JKI_lib_State_Machine.vi"("State(s) in (\"\")"=w787) -> ("States Out"=w786:string)  [unwired: 14 in]
      }
      frame "Data: saveBG" {
        w793 = "Background" ("name or relative path")
        w803 = T11."create or replace" ("operation (0:open)")
        w798 = string[] ["Ch1", "Ch2", "Ch3"] ("channel name(s) in (Untitled)")
        w796 = "Background" ("group name in (Untitled)")
        w816 = enum16{"write", "read"}."write" ("action")
        # "Save BG and pass it to FGV.\n(save BG to disk and set it to FGV)"
        n361 = Unbundle By Name(w819) -> ("Ch1Data"=w818:dbl[][], "Ch2Data"=w817:dbl[][], "Ch3Data"=w815:dbl[][], "Pathes.BG Path"=w788:path, "TempPath"=w791:path, "IDs.BG ID"=w794:i8)
        n362 = Format Value(string ("")=w793, format string="%02d", value (0)=w794) -> (output string=w792:string)
        n363 = Build Path(base path=w788, name or relative path=w792) -> (appended path=w790:path)
        n364 = Build Path(base path=w791, name or relative path=w793) -> (appended path=w799:path)
        n365 = call "AvgArray.vi"("2D array"=w818) -> ("1D Avg"=w812:dbl[])  [unwired: 10 in]
        n366 = call "AvgArray.vi"("2D array"=w817) -> ("1D Avg"=w811:dbl[])  [unwired: 10 in]
        n367 = call "AvgArray.vi"("2D array"=w815) -> ("1D Avg"=w810:dbl[])  [unwired: 10 in]
        n368 = TDMS Open(8:w789, 10:w803, 11:w790) -> (0:w813:errorcluster, 3:w814:refnum<k34>)  [unwired: 4 in]
        n369 = call "BG1FGV.vi"("action"=w816, "BG1 in"=w812) -> ()  [unwired: 8 in, 2 out]
        n370 = call "BG2FGV.vi"("action"=w816, "BG1 in"=w811) -> ()  [unwired: 8 in, 2 out]
        n371 = call "BG3FGV.vi"("action"=w816, "BG1 in"=w810) -> ()  [unwired: 8 in, 2 out]
        n372 = TDMS Open(8:w789, 10:w803, 11:w799) -> (0:w806:errorcluster, 3:w807:refnum<k34>)  [unwired: 4 in]
        n373 = Build Array(w812, w811, w810) -> (w797:dbl[][])
        n374 = TDMS Write(0:w814, 5:w796, 7:w798, 9:w797, 11:w813) -> (4:w809:refnum<k34>, 15:w808:errorcluster)  [unwired: 1 in, 2 out]
        n375 = TDMS Write(0:w807, 5:w796, 7:w798, 9:w797, 11:w806) -> (4:w805:refnum<k34>, 15:w804:errorcluster)  [unwired: 1 in, 2 out]
        n376 = TDMS Close(8:w808, 11:w809) -> (0:w802:errorcluster)  [unwired: 1 out]
        n377 = TDMS Close(8:w804, 11:w805) -> (0:w801:errorcluster)  [unwired: 1 out]
        n378 = Merge Errors(w802, w801) -> (w800:errorcluster)
        n379 = call <vilib>:"Add State(s) to Queue__JKI_lib_State_Machine.vi"("State(s) in (\"\")"=w822) -> ("States Out"=w821:string)  [unwired: 14 in]
      }
      frame "Data: showBG" {
        # "Show BG in seperate window.\n()"
        n380 = call "showBG.vi"() -> ()  [unwired: 12 in]
        n381 = call <vilib>:"Add State(s) to Queue__JKI_lib_State_Machine.vi"("State(s) in (\"\")"=w827) -> ("States Out"=w826:string)  [unwired: 14 in]
      }
      frame "Data: irfAlignment" {
        w876 = enum16{"write", "read"}."write" ("action")
        w890 = enum16{"write", "read"}."read" ("action")
        # "do iRF alignment in this state\n(It is a separator no-op. You can make a copy of this frame to create a new Data frame)"
        n382 = Unbundle By Name(w854) -> ("Ch1Data"=w893:dbl[][], "Ch2Data"=w892:dbl[][], "Ch3Data"=w891:dbl[][])
        n383 = local read "length"() -> (w840:i32)
        n384 = local read "start Idx"() -> (w841:i32)
        n385 = call "Ch3DeconEngineFGV.vi"("Error In"=w889, "action"=w890) -> ("Error Out"=w883:errorcluster, "Ch3DeconEngine out"=w884:refnum<class "LaguerreDeconEngineClass.lvclass">)  [unwired: 8 in]
        n386 = call "Ch1DeconEngineFGV.vi"("Error In"=w889, "action"=w890) -> ("Error Out"=w887:errorcluster, "Ch1DeconEngine out"=w888:refnum<class "LaguerreDeconEngineClass.lvclass">)  [unwired: 8 in]
        n387 = call "Ch2DeconEngineFGV.vi"("Error In"=w889, "action"=w890) -> ("Error Out"=w885:errorcluster, "Ch2DeconEngine out"=w886:refnum<class "LaguerreDeconEngineClass.lvclass">)  [unwired: 8 in]
        n388 = call "AvgArray.vi"("2D array"=w891) -> ("1D Avg"=w828:dbl[])  [unwired: 10 in]
        n389 = call "AvgArray.vi"("2D array"=w892) -> ("1D Avg"=w829:dbl[])  [unwired: 10 in]
        n390 = call "AvgArray.vi"("2D array"=w893) -> ("1D Avg"=w830:dbl[])  [unwired: 10 in]
        n391 = call "RemoveDCBG.vi"(8:w840, "Channel"=w841, "WF in"=w828) -> ("DC"=w833:dbl, "WF out"=w842:dbl[])  [unwired: 6 in, 1 out]
        n392 = call "RemoveDCBG.vi"(8:w840, "Channel"=w841, "WF in"=w829) -> ("DC"=w835:dbl, "WF out"=w843:dbl[])  [unwired: 6 in, 1 out]
        n393 = call "RemoveDCBG.vi"(8:w840, "Channel"=w841, "WF in"=w830) -> ("DC"=w838:dbl, "WF out"=w844:dbl[])  [unwired: 6 in, 1 out]
        n394 = call "computeIRFAlignment.vi"("error in (no error)"=w883, "fIRF temp"=w842, "LaguerreDeconEngineClass in"=w884) -> ("error out"=w881:errorcluster, "LaguerreDeconEngineClass out"=w882:refnum<class "LaguerreDeconEngineClass.lvclass">)  [unwired: 6 in, 1 out]
        n395 = call "computeIRFAlignment.vi"("error in (no error)"=w885, "fIRF temp"=w843, "LaguerreDeconEngineClass in"=w886) -> ("error out"=w877:errorcluster, "LaguerreDeconEngineClass out"=w878:refnum<class "LaguerreDeconEngineClass.lvclass">)  [unwired: 6 in, 1 out]
        n396 = call "computeIRFAlignment.vi"("error in (no error)"=w887, "fIRF temp"=w844, "LaguerreDeconEngineClass in"=w888) -> ("error out"=w879:errorcluster, "LaguerreDeconEngineClass out"=w880:refnum<class "LaguerreDeconEngineClass.lvclass">)  [unwired: 6 in, 1 out]
        n397 = call "Ch1DeconEngineFGV.vi"("Error In"=w879, "action"=w876, "Ch1DeconEngine in"=w880) -> ("Error Out"=w874:errorcluster, "Ch1DeconEngine out"=w875:refnum<class "LaguerreDeconEngineClass.lvclass">)  [unwired: 7 in]
        n398 = call "Ch2DeconEngineFGV.vi"("Error In"=w877, "action"=w876, "Ch2DeconEngine in"=w878) -> ("Error Out"=w864:errorcluster, "Ch2DeconEngine out"=w865:refnum<class "LaguerreDeconEngineClass.lvclass">)  [unwired: 7 in]
        n399 = call "Ch3DeconEngineFGV.vi"("Error In"=w881, "action"=w876, "Ch3DeconEngine in"=w882) -> ("Error Out"=w858:errorcluster, "Ch3DeconEngine out"=w859:refnum<class "LaguerreDeconEngineClass.lvclass">)  [unwired: 7 in]
        n400 = call "setfIRF.vi"("error in (no error)"=w858, "fIRF"=w842, "LaguerreDeconEngineClass in"=w859) -> ("error out"=w862:errorcluster, "LaguerreDeconEngineClass out"=w863:refnum<class "LaguerreDeconEngineClass.lvclass">)  [unwired: 7 in]
        n401 = call "setfIRF.vi"("error in (no error)"=w864, "fIRF"=w843, "LaguerreDeconEngineClass in"=w865) -> ("error out"=w868:errorcluster, "LaguerreDeconEngineClass out"=w869:refnum<class "LaguerreDeconEngineClass.lvclass">)  [unwired: 7 in]
        n402 = call "setfIRF.vi"("error in (no error)"=w874, "fIRF"=w844, "LaguerreDeconEngineClass in"=w875) -> ("error out"=w872:errorcluster, "LaguerreDeconEngineClass out"=w873:refnum<class "LaguerreDeconEngineClass.lvclass">)  [unwired: 7 in]
        n403 = call "computeLCs.vi"("error in (no error)"=w862, "LaguerreDeconClass in"=w863) -> ("error out"=w860:errorcluster, "LaguerreDeconClass out"=w861:refnum<class "LaguerreDeconEngineClass.lvclass">)  [unwired: 8 in]
        n404 = call "computeLCs.vi"("error in (no error)"=w868, "LaguerreDeconClass in"=w869) -> ("error out"=w866:errorcluster, "LaguerreDeconClass out"=w867:refnum<class "LaguerreDeconEngineClass.lvclass">)  [unwired: 8 in]
        n405 = call "computeLCs.vi"("error in (no error)"=w872, "LaguerreDeconClass in"=w873) -> ("error out"=w870:errorcluster, "LaguerreDeconClass out"=w871:refnum<class "LaguerreDeconEngineClass.lvclass">)  [unwired: 8 in]
        n406 = Unbundle By Name(w854) -> ("V1"=w853:dbl[], "V2"=w852:dbl[], "V3"=w851:dbl[])
        n407 = call-poly <vilib>:"Mean.vi"("X"=w853) -> ("mean"=w850:dbl)  [unwired: 1 out]
        n408 = call "getFitting.vi"("error in (no error)"=w860, "LaguerreDeconEngineClass in"=w861) -> ("Fitting"=w831:dbl[])  [unwired: 7 in, 2 out]
        n409 = call "getFitting.vi"("error in (no error)"=w866, "LaguerreDeconEngineClass in"=w867) -> ("Fitting"=w834:dbl[])  [unwired: 7 in, 2 out]
        n410 = call "getFitting.vi"("error in (no error)"=w870, "LaguerreDeconEngineClass in"=w871) -> ("Fitting"=w837:dbl[])  [unwired: 7 in, 2 out]
        n411 = Add(x=w838, y=w837) -> (x+y=w839:dbl[])
        n412 = Add(x=w835, y=w834) -> (x+y=w836:dbl[])
        n413 = call-poly <vilib>:"Mean.vi"("X"=w852) -> ("mean"=w849:dbl)  [unwired: 1 out]
        n414 = Add(x=w833, y=w831) -> (x+y=w832:dbl[])
        n415 = Build Array(w830, w839) -> (w857:dbl[][])
        n416 = Build Array(w829, w836) -> (w856:dbl[][])
        n417 = call-poly <vilib>:"Mean.vi"("X"=w851) -> ("mean"=w848:dbl)  [unwired: 1 out]
        n418 = Build Array(w828, w832) -> (w855:dbl[][])
        n419 = Bundle("mean"=w850, "mean"=w849, "mean"=w848) -> (w847:cluster{"mean":dbl, "mean":dbl, "mean":dbl})  [unwired: 1 in]
        n420 = call "Calib_and_iRFAlign_confirm.vi"("Cluster"=w847, "Ch3 Data"=w855, "Ch2 Data"=w856, "Ch1 Data"=w857) -> ("Save?"=w846:bool)  [unwired: 7 in]
        n421 = case shown="True" w846 {
          tunnel: ["" "Data: saveCalibration\nData: saveiRF\nRun: CaliIncrement"] -> w845
          frame False {
          }
          frame True {
          }
        }
        n422 = call <vilib>:"Add State(s) to Queue__JKI_lib_State_Machine.vi"("State(s) in Front (\"\")"=w845, "State(s) in (\"\")"=w896) -> ("States Out"=w895:string)  [unwired: 13 in]
      }
      frame "Data: saveRunData" {
        (unwired) i16 0 ("width (-)")
        # "Save FLIm data to disk.\n(Save to LV tdms file format)"
        n423 = Unbundle By Name(w935) -> ("Pathes.DataPath"=w934:path, "CaseID"=w902:string, "IDs.RunID"=w901:i8, "Ch1Data"=w928:dbl[][], "Ch2Data"=w924:dbl[][], "Ch3Data"=w920:dbl[][], "V1"=w916:dbl[], "V2"=w913:dbl[], "V3"=w911:dbl[])
        n424 = Format Value(string ("")=w902, format string="%02d", value (0)=w901) -> (output string=w899:string)
        n425 = Build Path(base path=w934, name or relative path=w899) -> (appended path=w933:path)
        n426 = TDMS Open(8:w906, 10:T11."open or create" ("operation (0:open)"), 11:w933) -> (0:w930:errorcluster, 3:w931:refnum<k34>)  [unwired: 4 in]
        n427 = TDMS Write(0:w931, 5:"CH1Data" ("group name in (Untitled)"), 9:w928, 11:w930) -> (4:w927:refnum<k34>, 15:w926:errorcluster)  [unwired: 2 in, 2 out]
        n428 = TDMS Write(0:w927, 5:"Ch2Data" ("group name in (Untitled)"), 9:w924, 11:w926) -> (4:w922:refnum<k34>, 15:w921:errorcluster)  [unwired: 2 in, 2 out]
        n429 = TDMS Write(0:w922, 5:"Ch3Data" ("group name in (Untitled)"), 9:w920, 11:w921) -> (4:w919:refnum<k34>, 15:w918:errorcluster)  [unwired: 2 in, 2 out]
        n430 = TDMS Write(0:w919, 5:"Ch1V" ("group name in (Untitled)"), 9:w916, 11:w918) -> (4:w905:refnum<k34>, 15:w915:errorcluster)  [unwired: 2 in, 2 out]
        n431 = TDMS Write(0:w905, 5:"Ch2V" ("group name in (Untitled)"), 9:w913, 11:w915) -> (4:w910:refnum<k34>, 15:w909:errorcluster)  [unwired: 2 in, 2 out]
        n432 = TDMS Write(0:w910, 5:"Ch3V" ("group name in (Untitled)"), 9:w911, 11:w909) -> (4:w908:refnum<k34>, 15:w907:errorcluster)  [unwired: 2 in, 2 out]
        n433 = TDMS Close(8:w907, 11:w908) -> (0:w904:errorcluster)  [unwired: 1 out]
        n434 = case shown="No Error" w904 {
          tunnel: [w939 ""] -> w903
          frame No Error {
            w939 = "Run: Increment"  # Run: Increment
          }
          frame Error {
          }
        }
        n435 = call <vilib>:"Add State(s) to Queue__JKI_lib_State_Machine.vi"("State(s) in Front (\"\")"=w903, "State(s) in (\"\")"=w938) -> ("States Out"=w937:string)  [unwired: 13 in]
      }
      frame "Data: Cleanup" {
        # "Cleanup any data and references, here.\n(this is called automatically, by the Macro: Exit)"
        n436 = Unbundle By Name(w942) -> ("Core.Current VI Reference"=w945:refnum<vi>)
        n437 = Close Reference(reference=w945, error in (no error)=w944) -> (error out=w943:errorcluster)
        n438 = call <vilib>:"Add State(s) to Queue__JKI_lib_State_Machine.vi"("State(s) in (\"\")"=w947) -> ("States Out"=w946:string)  [unwired: 14 in]
      }
      frame "---------- Core ----------" {
        # "Do not put any code in this frame.\n(it is a separator no-op)"
        n439 = call <vilib>:"Add State(s) to Queue__JKI_lib_State_Machine.vi"("State(s) in (\"\")"=w952) -> ("States Out"=w951:string)  [unwired: 14 in]
      }
      frame Default {
        w963 = 42 items=["No error", "Argument error", "Memory is full", "Out of zone", "End of file", "File already open", "Generic file I/O error", "File not found", "File permission error", "Disk is full", "Duplicate path", "Too many files open", "System feature not enabled", "Resource file not found", "Cannot add resource", "Resource not found", "Image not found", "Image memory error", "Pen does not exist", "Config type invalid", "Config token not found", "Config parse error", "Config memory error", "Bad external code format", "Bad external code offset", "External code not present", "Null window", "Destroy window error", "Null menu", "Print aborted", "Bad print record", "Print driver error", "Windows error during printing", "Memory error during printing", "Print dialog error", "Generic print error", "Invalid device refnum", "Device not found", "Device parameter error", "Device unit error", "Cannot open device", "Device call aborted", "Generic error", "Cancelled by user", "Object ID too low", "Object ID too high", "Object not in heap", "Unknown heap", "Unknown object (invalid DefProc)", "Unknown object (DefProc not in table)", "Message out of range", "Invalid (null) method", "Unknown message", "Manager call not supported", "Bad address", "Network operation in progress", "Network operation timed out", "Connection is busy", "Network attribute not supported", "Network error", "Address in use", "System out of memory", "Connection aborted", "Connection refused", "Not connected", "Already connected", "Connection closed", "Initialization error (interapplication manager)", "Bad occurrence", "Wait on unbound occurrence handler", "Occurrence queue overflow", "Datalog type conflict", "Unused", "Unrecognized type (interapplication manager)", "Memory corrupt", "Failed to make temporary DLL", "Old CIN version", "Drag socket not found", "Failed to load drop-object", "Failed to register OLE object", "Failed to release OLE object", "Format specifier type mismatch", "Unknown format specifier", "Too few format specifiers", "Too many format specifiers", "Scan failed", "Newer CIN version", "Error converting to variant", "Runtime menu error", "Password tampered", "Variant attribute not found", "Incompatible variant data type", "Event data is not available", "Event Store is not present", "Occurrence is not found", "Event Queue is not created", "Event info is not available", "Refnum passed is NULL", "Error retrieving Class GUID", "Error retrieving CoClass GUID", "Error retrieving TypeLib GUID.", "Bad built application magic bytes.", "Specific driver is different from the specific driver associated with the Logical Name.", "There is no session opened to the class driver.", "Max Error", "MAX - Error with config objects", "MAX - Error loading configuration", "MAX - Group not supported"]
        # "Current State"
        # "Do not delete, rename, or modify this frame.\n(this is used to capture unhandled states and typos)"
        # "Handle mistyped state name (developer tool)"
        n440 = Format Into String(format string="Software Exception: Unhandled State \"%s\"." ("message"), error in=w959, w954) -> (resulting string=w962:string, error out=w961:errorcluster)  [unwired: 1 in]
        n441 = call <vilib>:"Error Cluster From Error Code.vi"("show call chain? (False)"=TRUE, "error in (no error)"=w961, "error message (\"\")"=w962, "error code (0)"=w963) -> ("error out"=w960:errorcluster)  [unwired: 5 in]
        n442 = call <vilib>:"Add State(s) to Queue__JKI_lib_State_Machine.vi"("State(s) in (\"\")"=w958) -> ("States Out"=w957:string)  [unwired: 14 in]
      }
      frame "Initialize Core Data" {
        # "Build default path based on the location of project"
        # "Do not delete, rename, or modify this frame.\n(this is used to determine panel behavior on exit)"
        # "originally closed?"
        # "exe?"
        # "If panel starts closed or is an EXE, then close it when we exit"
        n443 = call <vilib>:"Application Directory.vi"() -> ("Application Directory"=w965:path)
        n444 = property class="App"() -> ("App.Kind"=w979:T13)  [unwired: 2 in, 2 out]
        n445 = property class="VI"() -> ("FP.State"=w973:T12)  [unwired: 2 in, 2 out]
        n446 = control-ref of="Current VI Reference"() -> (w974:refnum<vi>)
        n447 = Equal?(x=w973, y=T12."Closed" ("Front Panel Window:State")) -> (x = y?=w971:bool)
        n448 = Equal?(x=w979, y=T13."Run Time System" ("Application:Kind")) -> (x = y?=w977:bool)
        n449 = Build Path(base path=w965, name or relative path="Data") -> (appended path=w969:path)
        n450 = Build Path(base path=w965, name or relative path="SystemTemp") -> (appended path=w966:path)
        n451 = Or(x=w971, y=w977) -> (x .or. y?=w975:bool)
        n452 = Bundle By Name(cluster=w976, "Core.Current VI Reference"=w974, "Core.Close Panel on Exit?"=w975, "DefaultPath"=w969, "TempPath"=w966) -> (w981:T16)
        n453 = call <vilib>:"Add State(s) to Queue__JKI_lib_State_Machine.vi"("State(s) in (\"\")"=w983) -> ("States Out"=w982:string)  [unwired: 14 in]
      }
      frame "Error Handler" {
        # "Unhandled Error -- Display it"
        # "Handle any errors here.\nYou can also output any states to clean-up after errors occur"
        # "Clear error"
        n454 = Unbundle By Name(w984) -> ("code"=w986:i32)
        n455 = case shown="5002" w986 {
          tunnel: ["Macro: Exit" w996 w1002] -> w985
          tunnel: w984 -> [w992 _ _]
          frame Default {
            w994 = T25 2 items=["no dialog", "OK message", "continue or stop message", "OK message + warnings", "continue/stop + warnings"] ("type of dialog (OK msg:1)")
            n456 = call <vilib>:"General Error Handler.vi"("type of dialog (OK msg:1)"=w994, "error in (no error)"=w992) -> ()  [unwired: 9 in, 5 out]
          }
          frame 5002 {
            n457 = Two Button Dialog(message="Laser interlock open! Please close interlock and try again! ", 1:"Safely Shutdown" ("F button name (\"Cancel\")"), 2:"OK" ("T button name (\"OK\")")) -> (T button?=w997:bool)
            n458 = case shown="False" w997 {
              tunnel: ["Macro: Exit" "355 Laser: CheckControllerStatus"] -> w996
              frame False {
              }
              frame True {
              }
            }
          }
          frame 5001 {
            n459 = Two Button Dialog(message="Unable to connect to imaging computer, do you want to run data aquisiton along? ", 1:"No" ("F button name (\"Cancel\")"), 2:"Yes" ("T button name (\"OK\")")) -> (T button?=w1003:bool)
            n460 = case shown="True" w1003 {
              tunnel: ["Macro: Exit" ""] -> w1002
              frame False {
              }
              frame True {
              }
            }
          }
        }
        n461 = call <vilib>:"Add State(s) to Queue__JKI_lib_State_Machine.vi"("State(s) in Front (\"\")"=w985, "State(s) in (\"\")"=w991) -> ("States Out"=w990:string)  [unwired: 13 in]
      }
      frame "Exit" {
        # "Do not put any code in this frame.\n(No errors that occur here will be handled.)"
        n462 = call <vilib>:"Add State(s) to Queue__JKI_lib_State_Machine.vi"("State(s) in (\"\")"=w1014) -> ("States Out"=w1013:string)  [unwired: 14 in]
      }
      frame "---------- Macro ----------" {
        # "Do not put any code in this frame.\n(It is a separator no-op. You can make a copy of this frame to create a new Macro frame)"
        n463 = call <vilib>:"Add State(s) to Queue__JKI_lib_State_Machine.vi"("State(s) in (\"\")"=w1019) -> ("States Out"=w1018:string)  [unwired: 14 in]
      }
      frame "Macro: Initialize" {
        # "load Labjack setting 1st as it contaisn laser pin infortmation"
        # "start laser 1st, need 7.5s for laser to get ready"
        # "Initialization Macro\n(This is called once, when the VI starts)"
        n464 = call <vilib>:"Add State(s) to Queue__JKI_lib_State_Machine.vi"("State(s) in Front (\"\")"="UI: showDisclaimer\nUI: Cursor Set >> Busy\nGraph: AddCursors\nData: Initialize\nInitialize Core Data\nUI: Initialize\nUI: Front Panel State >> Open\nUI: Update\nMacro: LoadSysConfig\nLabJack: Open\nLabJack: SetDefaultSub\nLED: Yellow\nLED: OpenVIRef\nLED: Breath >> True\nUI: Update\n355 Laser: Laser enable/disable\n355 Laser: Dewelling>>500\n355 Laser: CheckControllerStatus\nUI: Update\nLabJack: 355_PWM_Config\nLabJack: AB_PWM_Config\nTCP: Initialize\nTCP: SyncTime\nUI: Update\n", "State(s) in (\"\")"="Digitizer: Initialize\nDigitizer: Config\nUI: Update\nAimingBeam: Initialize\nAimingBeam: Set Status>>Enable\nAimingBeam: Set Current\nUI: Update\n355 Laser: Check Dewelling\nUI: Cursor Set >> Idle\nCase: GetID\nUI: Update\nTCP: SendSettingMacro\nCase: CreatFileStruct\nUI: Update\nData: loadLastUseMacro\nDeconEngine: InitilizeMacro\nUI: ReadyForAquisition\nLED: Breath >> False") -> ("States Out"=w1020:string)  [unwired: 13 in]
        n465 = call <vilib>:"Add State(s) to Queue__JKI_lib_State_Machine.vi"("State(s) in Front (\"\")"=w1020, "State(s) in (\"\")"=w1028) -> ("States Out"=w1027:string)  [unwired: 13 in]
        "Help" <- "Hover over controls to see help!" ("Help")
      }
      frame "Macro: LoadSysConfig" {
        # "System configuration Macro\n(Load configurations for different component of the system)"
        n466 = call <vilib>:"Add State(s) to Queue__JKI_lib_State_Machine.vi"("State(s) in Front (\"\")"="SysConfig: Load Sys Config\nSysConfig: Load Digitizer Setting\nSysConfig: Load AB setting\nSysConfig: Load LJ Pinout\nSysConfig: Load 355 PWM\nSysConfig: Load AB PWM", "State(s) in (\"\")"=w1034) -> ("States Out"=w1033:string)  [unwired: 13 in]
      }
      frame "Macro: Exit" {
        # "close LJ last"
        # "check whether hardware is initilized, if so close, if not do nothing"
        # "Exit Macro, close all hardware\n(This is called once, when the VI exits)"
        n467 = Unbundle By Name(w1054) -> ("System Status.TCP/IP"=w1042:bool, "System Status.Digitizer"=w1050:bool, "System Status.Aiming Beam"=w1049:bool, "System Status.355 Laser"=w1048:bool, "System Status.Labjack"=w1038:bool, "Core.Close Panel on Exit?"=w1043:bool)
        n468 = case shown="True" w1050 {
          tunnel: ["" "Digitizer: Close"] -> w1045
          frame False {
          }
          frame True {
          }
        }
        n469 = case shown="True" w1042 {
          tunnel: ["" "TCP: Close"] -> w1044
          frame False {
          }
          frame True {
          }
        }
        n470 = case shown="True" w1038 {
          tunnel: ["" "LabJack: SetDefaultAndClose"] -> w1035
          frame False {
          }
          frame True {
          }
        }
        n471 = case shown="True" w1049 {
          tunnel: ["" "AimingBeam: Set Status >> Disable\nAimingBeam: Close"] -> w1037
          frame False {
          }
          frame True {
          }
        }
        n472 = case shown="True" w1048 {
          tunnel: ["" "355 Laser: Close\n355 Laser: CheckControllerStatus"] -> w1036
          frame False {
          }
          frame True {
          }
        }
        n473 = Select(t="UI: Front Panel State >> Close", s=w1043, f="") -> (s? t:f=w1039:string)
        n474 = call <vilib>:"Add State(s) to Queue__JKI_lib_State_Machine.vi"("State(s) in Front (\"\")"=w1044, "State(s) in (\"\")"=w1045, "State(s) at Back (\"\")"=w1037) -> ("States Out"=w1047:string)  [unwired: 12 in]
        n475 = call <vilib>:"Add State(s) to Queue__JKI_lib_State_Machine.vi"("State(s) in Front (\"\")"=w1047, "State(s) in (\"\")"=w1036, "State(s) at Back (\"\")"=w1035) -> ("States Out"=w1041:string)  [unwired: 12 in]
        n476 = call <vilib>:"Add State(s) to Queue__JKI_lib_State_Machine.vi"("State(s) in Front (\"\")"=w1041, "State(s) in (\"\")"="UI: Update\nUI: Reset\nLED: CloseVIRef\nQueue: Destory\nData: Cleanup\nExit", "State(s) at Back (\"\")"=w1039) -> ("States Out"=w1051:string)  [unwired: 12 in]
        n477 = call <vilib>:"Add State(s) to Queue__JKI_lib_State_Machine.vi"("State(s) in Front (\"\")"=w1051, "State(s) in (\"\")"=w1057) -> ("States Out"=w1056:string)  [unwired: 13 in]
      }
      frame "---------- AimingBeam ----------" {
        # "Template Separator\n(You can make a copy of, or modify, this frame)"
        n478 = call <vilib>:"Add State(s) to Queue__JKI_lib_State_Machine.vi"("State(s) in (\"\")"=w1072) -> ("States Out"=w1071:string)  [unwired: 14 in]
      }
      frame "AimingBeam: Initialize" {
        # "set aiming beam button color"
        # "Open COM port for Aiming Beam\n(Require USB connection)"
        n479 = Unbundle By Name(w1074) -> ("AB Cluster.Aiming Beam COM Port"=w1082:refnum<visa-resource-name>)
        n480 = call-poly "VISA Configure Serial Port"("VISA resource name"=w1082, "Enable Termination\nChar (T)"=TRUE ("Enable Termination\nChar (T)"), "baud rate (9600)"=u32 9600, "error in (no error)"=w1079) -> ("error out"=w1078:errorcluster)  [unwired: 10 in, 1 out]
        n481 = Unbundle By Name(w1078) -> ("status"=w1077:bool)
        n482 = Not(x=w1077) -> (.not. x?=w1076:bool)
        n483 = Bundle By Name(cluster=w1074, "System Status.Aiming Beam"=w1076) -> (w1075:T16)
        n484 = call <vilib>:"Add State(s) to Queue__JKI_lib_State_Machine.vi"("State(s) in (\"\")"=w1084) -> ("States Out"=w1083:string)  [unwired: 14 in]
      }
      frame "AimingBeam: Close" {
        # "Close Aiming Beam COM port\n(Require USB connection to Aiming Beam Laser)"
        n485 = Unbundle By Name(w1087) -> ("AB Cluster.Aiming Beam COM Port"=w1091:refnum<visa-resource-name>)
        n486 = VISA Close(VISA resource name=w1091, error in (no error)=w1089) -> (error out=w1090:errorcluster)
        n487 = Bundle By Name(cluster=w1087, "System Status.Aiming Beam"=FALSE) -> (w1088:T16)
        n488 = call <vilib>:"Add State(s) to Queue__JKI_lib_State_Machine.vi"("State(s) in (\"\")"=w1093) -> ("States Out"=w1092:string)  [unwired: 14 in]
      }
      frame "AimingBeam: Set Current" {
        # "Set Aiming Beam Current\n(You can make a copy of, or modify, this frame)"
        n489 = Unbundle By Name(w1113) -> ("AB Cluster.Aiming Beam COM Port"=w1106:refnum<visa-resource-name>, "AB Cluster.Max Current"=w1102:dbl, "AB Cluster.Default Current"=w1104:dbl, "AB Cluster.Min Current"=w1103:dbl)
        n490 = In Range and Coerce(upper limit=w1102, x=w1104, lower limit=w1103) -> (coerced(x)=w1099:dbl)  [unwired: 1 out]
        n491 = property on="Aiming beam toggle" class="Bool (strict)"() -> ("Caption.Text"=w1094:string)  [unwired: 2 in, 2 out]
        n492 = Number To Fractional String(number=w1099, precision (6)=i16 2) -> (F-format string=w1107:string)  [unwired: 2 in]
        n493 = Concatenate Strings("slc:", w1107, "\r", "\n") -> (w1110:string)
        n494 = Number To Decimal String(number=w1099, width (-)=i16 2) -> (decimal integer string=w1098:string)
        n495 = VISA Write(VISA resource name=w1106, write buffer=w1110, error in (no error)=w1101) -> (error out=w1105:errorcluster)  [unwired: 2 out]
        n496 = Concatenate Strings(w1094, w1098, "mA" ("string")) -> (w1096:string)
        n497 = property on="Aiming beam toggle" class="Bool (strict)"("Caption.Text"=w1096) -> ()  [unwired: 2 in, 2 out]
        n498 = call <vilib>:"Add State(s) to Queue__JKI_lib_State_Machine.vi"("State(s) in (\"\")"=w1115) -> ("States Out"=w1114:string)  [unwired: 14 in]
      }
      frame "AimingBeam: Set Status" {
        # "Enable Aiming Beam\n(Usage: \"AimingBeam: Set >> Enable|Disable\")"
        n499 = Unbundle By Name(w1122) -> ("AB Cluster.Aiming Beam COM Port"=w1119:refnum<visa-resource-name>)
        n500 = case shown="\"Enable\"" w1121 {
          tunnel: [w1125 w1129] -> w1120
          frame "Disable", Default {
            n501 = Concatenate Strings("cof", "\r", "\n") -> (w1125:string)
          }
          frame "Enable" {
            n502 = Concatenate Strings("con", "\r", "\n") -> (w1129:string)
          }
        }
        n503 = VISA Write(VISA resource name=w1119, write buffer=w1120, error in (no error)=w1117) -> (error out=w1118:errorcluster)  [unwired: 2 out]
        n504 = call <vilib>:"Add State(s) to Queue__JKI_lib_State_Machine.vi"("State(s) in (\"\")"=w1124) -> ("States Out"=w1123:string)  [unwired: 14 in]
      }
      frame "AimingBeam: GetPWMStatus" {
        # "Get aiming beam PWM status\n()"
        n505 = Unbundle By Name(w1133) -> ("LJ Pinout.AimingBeam PWM"=w1142:string)
        n506 = call "LabJack_FGV.vi"("Operation(Read)"=enum16{"Write", "Read"}."Read" ("Operation"), "error in (no error)"=w1135) -> ("error out"=w1139:errorcluster, "Read data"=w1140:i32)  [unwired: 8 in]
        n507 = Concatenate Strings(w1142, "_EF_ENABLE" ("string")) -> (w1138:string)
        n508 = call <vilib>:"LJM_eReadName.vi"("Handle In"=w1140, "Name"=w1138, "error in"=w1139) -> ("Value"=w1137:dbl, "error out"=w1134:errorcluster)  [unwired: 10 in, 1 out]
        n509 = Greater Than 0?(x=w1137) -> (x > 0?=w1136:bool)
        n510 = case shown="False" w1136 {
          frame False {
            # "PWM is off\nset color to dark green"
            n511 = local write "Aiming beam toggle"(FALSE ("Aimging beam")) -> ()
          }
          frame True {
            # "PWM is on\nset color to light green"
            n512 = local write "Aiming beam toggle"(TRUE ("Aimging beam")) -> ()
          }
        }
        n513 = call <vilib>:"Add State(s) to Queue__JKI_lib_State_Machine.vi"("State(s) in (\"\")"=w1146) -> ("States Out"=w1145:string)  [unwired: 14 in]
      }
      frame "---------- Case ----------" {
        # "Template Separator\n(You can make a copy of, or modify, this frame)"
        n514 = call <vilib>:"Add State(s) to Queue__JKI_lib_State_Machine.vi"("State(s) in (\"\")"=w1153) -> ("States Out"=w1152:string)  [unwired: 14 in]
      }
      frame "Case: getCaliID" {
        # "Get Calibration file #\n(You can make a copy of, or modify, this frame)"
        n515 = Unbundle By Name(w1155) -> ("Pathes.CaliPath"=w1158:path)
        n516 = call <vilib>:"Recursive File List.vi"("pattern"="*.tdms", "Treat LLBs as Folders?"=FALSE, "Folder Path"=w1158) -> ("All Files in Dir"=w1163:path[])  [unwired: 4 in, 4 out]
        n517 = for {
          tunnel: w1163 -> [w1173] mode=indexing
          tunnel: [w1172] -> w1162 mode=indexing
          tunnel: "Calibration" -> [w1169]
          n518 = Strip Path(path=w1173) -> (name=w1170:string)  [unwired: 1 out]
          n519 = Search and Replace String(input string=w1170, search string=w1169) -> (result string=w1168:string)  [unwired: 6 in, 3 out]
          n520 = Scan From String(format string="%d" ("string"), input string=w1168) -> (output 1=w1172:i32)  [unwired: 3 in, 3 out]
        }
        n521 = Array Max & Min(array=w1162) -> (max value=w1161:i32)  [unwired: 3 out]
        n522 = Increment(x=w1161) -> (x+1=w1154:i32)
        n523 = Bundle By Name(cluster=w1155, "IDs.Cali ID"=w1154) -> (w1156:T16)
        n524 = call <vilib>:"Add State(s) to Queue__JKI_lib_State_Machine.vi"("State(s) in (\"\")"=w1167) -> ("States Out"=w1166:string)  [unwired: 14 in]
      }
      frame "Case: getBGID" {
        # "Get background #\n(You can make a copy of, or modify, this frame)"
        n525 = Unbundle By Name(w1174) -> ("Pathes.BG Path"=w1182:path)
        n526 = call <vilib>:"Recursive File List.vi"("pattern"="*.tdms", "Treat LLBs as Folders?"=FALSE, "Folder Path"=w1182) -> ("All Files in Dir"=w1178:path[])  [unwired: 4 in, 4 out]
        n527 = for {
          tunnel: w1178 -> [w1193] mode=indexing
          tunnel: [w1192] -> w1179 mode=indexing
          tunnel: "Background" ("name or relative path") -> [w1189]
          n528 = Strip Path(path=w1193) -> (name=w1190:string)  [unwired: 1 out]
          n529 = Search and Replace String(input string=w1190, search string=w1189) -> (result string=w1188:string)  [unwired: 6 in, 3 out]
          n530 = Scan From String(format string="%d" ("string"), input string=w1188) -> (output 1=w1192:i32)  [unwired: 3 in, 3 out]
        }
        n531 = Array Max & Min(array=w1179) -> (max value=w1180:i32)  [unwired: 3 out]
        n532 = Increment(x=w1180) -> (x+1=w1176:i32)
        n533 = Bundle By Name(cluster=w1174, "IDs.BG ID"=w1176) -> (w1175:T16)
        n534 = call <vilib>:"Add State(s) to Queue__JKI_lib_State_Machine.vi"("State(s) in (\"\")"=w1187) -> ("States Out"=w1186:string)  [unwired: 14 in]
      }
      frame "Case: getRunID" {
        # "Check folder for run ID\n(You can make a copy of, or modify, this frame)"
        n535 = Unbundle By Name(w1199) -> ("Pathes.DataPath"=w1198:path, "CaseID"=w1194:string)
        n536 = Build Array("Background" ("name or relative path"), "Calibration") -> (w1206:string[])
        n537 = call <vilib>:"Recursive File List.vi"("Folders to Exclude"=w1206, "pattern"="*.tdms", "Treat LLBs as Folders?"=FALSE, "Folder Path"=w1198) -> ("All Files in Dir"=w1195:path[])  [unwired: 3 in, 4 out]
        n538 = for {
          tunnel: w1195 -> [w1216] mode=indexing
          tunnel: [w1215] -> w1202 mode=indexing
          tunnel: w1194 -> [w1212]
          n539 = Strip Path(path=w1216) -> (name=w1213:string)  [unwired: 1 out]
          n540 = Search and Replace String(input string=w1213, search string=w1212) -> (result string=w1211:string)  [unwired: 6 in, 3 out]
          n541 = Scan From String(format string="%d" ("string"), input string=w1211) -> (output 1=w1215:i32)  [unwired: 3 in, 3 out]
        }
        n542 = Array Max & Min(array=w1202) -> (max value=w1203:i32)  [unwired: 3 out]
        n543 = Increment(x=w1203) -> (x+1=w1201:i32)
        n544 = Bundle By Name(cluster=w1199, "IDs.RunID"=w1201) -> (w1200:T16)
        n545 = call <vilib>:"Add State(s) to Queue__JKI_lib_State_Machine.vi"("State(s) in (\"\")"=w1210) -> ("States Out"=w1209:string)  [unwired: 14 in]
      }
      frame "Case: CreatFileStruct" {
        # "Creat case file structure"
        n546 = Unbundle By Name(w1228) -> ("DefaultPath"=w1234:path, "CaseID"=w1219:string)
        n547 = Build Path(base path=w1234, name or relative path=w1219) -> (appended path=w1233:path)
        n548 = call <vilib>:"Check if File or Folder Exists.vi"("error in (no error)"=w1226, "path"=w1233) -> ("error out"=w1230:errorcluster, "file or folder exists?"=w1232:bool, "dup path"=w1231:path)  [unwired: 7 in]
        n549 = case shown="True" w1232 {
          tunnel: w1231 -> [w1251 w1259]
          tunnel: w1230 -> [w1249 w1254]
          tunnel: [w1243 w1259] -> w1224
          tunnel: [w1247 w1261] -> w1227
          tunnel: [u32 1 u32 0] -> w1218
          tunnel: [w1245 w1264] -> w1223
          tunnel: "Background" ("name or relative path") -> [w1244 w1256]
          tunnel: "Calibration" -> [w1242 w1255]
          tunnel: [w1238 w1257] -> w1220
          tunnel: w1219 -> [_ _]
          tunnel: ["" "Case: getRunID\nCase: getBGID\nCase: getCaliID"] -> w1217
          frame False {
            # "Folder not exist. Creat folders."
            n550 = Create Folder(path (use dialog)=w1251, error in=w1249) -> (created path=w1243:path, error out=w1240:errorcluster)  [unwired: 1 in, 1 out]
            n551 = Build Path(base path=w1243, name or relative path=w1242) -> (appended path=w1241:path)
            n552 = Build Path(base path=w1243, name or relative path=w1244) -> (appended path=w1250:path)
            n553 = Create Folder(path (use dialog)=w1250, error in=w1240) -> (created path=w1245:path, error out=w1246:errorcluster)  [unwired: 1 in, 1 out]
            n554 = Create Folder(path (use dialog)=w1241, error in=w1240) -> (created path=w1238:path, error out=w1239:errorcluster)  [unwired: 1 in, 1 out]
            n555 = Merge Errors(w1246, w1239) -> (w1247:errorcluster)
          }
          frame True {
            # "Folder exsit, check file #"
            n556 = Build Path(base path=w1259, name or relative path=w1255) -> (appended path=w1260:path)
            n557 = Build Path(base path=w1259, name or relative path=w1256) -> (appended path=w1265:path)
            n558 = call <vilib>:"Check if File or Folder Exists.vi"("path"=w1260) -> ("file or folder exists?"=w1258:bool, "dup path"=w1257:path)  [unwired: 8 in, 1 out]
            n559 = call <vilib>:"Check if File or Folder Exists.vi"("path"=w1265) -> ("file or folder exists?"=w1263:bool, "dup path"=w1264:path)  [unwired: 8 in, 1 out]
            n560 = And(x=w1263, y=w1258) -> (x .and. y?=w1262:bool)
            n561 = case shown="False" w1262 {
              tunnel: w1254 -> [_ w1267]
              tunnel: [errorcluster {"status"=TRUE, "code"=5003, "source"="File structure error."} ("error out") w1267] -> w1261
              frame False {
              }
              frame True {
              }
            }
          }
        }
        n562 = Bundle By Name(cluster=w1228, "Pathes.DataPath"=w1224, "Pathes.BG Path"=w1223, "Pathes.CaliPath"=w1220, "IDs.RunID"=w1218, "IDs.BG ID"=w1218, "IDs.Cali ID"=w1218) -> (w1229:T16)
        n563 = call <vilib>:"Add State(s) to Queue__JKI_lib_State_Machine.vi"("State(s) in Front (\"\")"=w1217, "State(s) in (\"\")"=w1236) -> ("States Out"=w1235:string)  [unwired: 13 in]
      }
      frame "Case: GetID" {
        # "Template Separator\n(You can make a copy of, or modify, this frame)"
        n564 = call "set_subjectID.vi"() -> ("subject_id"=w1268:string)  [unwired: 10 in]
        n565 = Bundle By Name(cluster=w1270, "CaseID"=w1268) -> (w1271:T16)
        n566 = call <vilib>:"Add State(s) to Queue__JKI_lib_State_Machine.vi"("State(s) in (\"\")"=w1274) -> ("States Out"=w1273:string)  [unwired: 14 in]
      }
      frame "---------- DeconEngine ----------" {
        # "start data aquisition and then set irfAligh to ture and decon channel to 1,2 and 3."
        # "Template Separator\n(You can make a copy of, or modify, this frame)"
        n567 = call <vilib>:"Add State(s) to Queue__JKI_lib_State_Machine.vi"("State(s) in (\"\")"=w1279) -> ("States Out"=w1278:string)  [unwired: 14 in]
      }
      frame "DeconEngine: InitilizeMacro" {
        # "start data aquisition and then set irfAligh to ture and decon channel to 1,2 and 3."
        # "Initilize Decon Engine for all channel\n(You can make a copy of, or modify, this frame)"
        n568 = call <vilib>:"Add State(s) to Queue__JKI_lib_State_Machine.vi"("State(s) in Front (\"\")"="DeconEngine: InitializeCh1\nDeconEngine: InitializeCh2\nDeconEngine: InitializeCh3" ("State(s) in Front (\"\")"), "State(s) in (\"\")"=w1285) -> ("States Out"=w1284:string)  [unwired: 13 in]
      }
      frame "DeconEngine: InitializeCh1" {
        w1310 = refnum<class "LaguerreDeconEngineClass.lvclass"> refnum  # Ch1DeconObj
        # "Initilize Laguerre Deconvolution engine Object\n(You can make a copy of, or modify, this frame)"
        n569 = global read "GlobalVariables.vi" "LastUseiRF"() -> (w1287:T26)
        n570 = call "FLImDAQ_FGV.vi"(6:enum16{"Write", "Read"}."Read" ("Operation"), "error in (no error)"=w1294) -> ("error out"=w1305:errorcluster, "Read data"=w1304:T5)  [unwired: 8 in]
        n571 = call "setLaguerreOrder.vi"("error in (no error)"=w1305, "LaguerreOrder"=u32 12, "LaguerreDeconClass in"=w1310) -> ("error out"=w1307:errorcluster, "LaguerreDeconClass out"=w1308:refnum<class "LaguerreDeconEngineClass.lvclass">)  [unwired: 7 in]
        n572 = Unbundle By Name(w1304) -> ("min record length"=w1303:i32)
        n573 = Unbundle By Name(w1287) -> ("Ch1 iRF"=w1286:dbl[])
        n574 = call "setDataLength.vi"("error in (no error)"=w1307, "dataLength"=w1303, "LaguerreDeconClass in"=w1308) -> ("error out"=w1302:errorcluster, "LaguerreDeconClass out"=w1301:refnum<class "LaguerreDeconEngineClass.lvclass">)  [unwired: 7 in]
        n575 = call "setIRF.vi"("error in (no error)"=w1302, "iRF"=w1286, "LaguerreDeconClass in"=w1301) -> ("error out"=w1299:errorcluster, "LaguerreDeconClass out"=w1300:refnum<class "LaguerreDeconEngineClass.lvclass">)  [unwired: 7 in]
        n576 = call "computeAlpha.vi"("error in (no error)"=w1299, "LaguerreDeconClass in"=w1300) -> ("error out"=w1297:errorcluster, "LaguerreDeconClass out"=w1298:refnum<class "LaguerreDeconEngineClass.lvclass">)  [unwired: 8 in]
        n577 = call "dataInitilize.vi"("error in (no error)"=w1297, "LaguerreDeconClass in"=w1298) -> ("error out"=w1295:errorcluster, "LaguerreDeconClass out"=w1296:refnum<class "LaguerreDeconEngineClass.lvclass">)  [unwired: 8 in]
        n578 = call "computeDeconMatrix.vi"("error in (no error)"=w1295, "LaguerreDeconClass in"=w1296) -> ("error out"=w1291:errorcluster, "LaguerreDeconClass out"=w1293:refnum<class "LaguerreDeconEngineClass.lvclass">)  [unwired: 8 in]
        n579 = call "Ch1DeconEngineFGV.vi"("Error In"=w1291, "action"=enum16{"write", "read"}."write", "Ch1DeconEngine in"=w1293) -> ("Error Out"=w1290:errorcluster)  [unwired: 7 in, 1 out]
        n580 = call <vilib>:"Add State(s) to Queue__JKI_lib_State_Machine.vi"("State(s) in (\"\")"=w1312) -> ("States Out"=w1311:string)  [unwired: 14 in]
      }
      frame "DeconEngine: InitializeCh2" {
        w1337 = refnum<class "LaguerreDeconEngineClass.lvclass"> refnum  # Ch2DeconObj
        # "Initilize Laguerre Deconvolution engine Object\n(You can make a copy of, or modify, this frame)"
        n581 = global read "GlobalVariables.vi" "LastUseiRF"() -> (w1314:T26)
        n582 = call "FLImDAQ_FGV.vi"(6:enum16{"Write", "Read"}."Read" ("Operation"), "error in (no error)"=w1322) -> ("error out"=w1315:errorcluster, "Read data"=w1332:T5)  [unwired: 8 in]
        n583 = call "setLaguerreOrder.vi"("error in (no error)"=w1315, "LaguerreOrder"=u32 12, "LaguerreDeconClass in"=w1337) -> ("error out"=w1334:errorcluster, "LaguerreDeconClass out"=w1335:refnum<class "LaguerreDeconEngineClass.lvclass">)  [unwired: 7 in]
        n584 = Unbundle By Name(w1332) -> ("min record length"=w1331:i32)
        n585 = Unbundle By Name(w1314) -> ("Ch2 iRF"=w1313:dbl[])
        n586 = call "setDataLength.vi"("error in (no error)"=w1334, "dataLength"=w1331, "LaguerreDeconClass in"=w1335) -> ("error out"=w1330:errorcluster, "LaguerreDeconClass out"=w1329:refnum<class "LaguerreDeconEngineClass.lvclass">)  [unwired: 7 in]
        n587 = call "setIRF.vi"("error in (no error)"=w1330, "iRF"=w1313, "LaguerreDeconClass in"=w1329) -> ("error out"=w1327:errorcluster, "LaguerreDeconClass out"=w1328:refnum<class "LaguerreDeconEngineClass.lvclass">)  [unwired: 7 in]
        n588 = call "computeAlpha.vi"("error in (no error)"=w1327, "LaguerreDeconClass in"=w1328) -> ("error out"=w1325:errorcluster, "LaguerreDeconClass out"=w1326:refnum<class "LaguerreDeconEngineClass.lvclass">)  [unwired: 8 in]
        n589 = call "dataInitilize.vi"("error in (no error)"=w1325, "LaguerreDeconClass in"=w1326) -> ("error out"=w1323:errorcluster, "LaguerreDeconClass out"=w1324:refnum<class "LaguerreDeconEngineClass.lvclass">)  [unwired: 8 in]
        n590 = call "computeDeconMatrix.vi"("error in (no error)"=w1323, "LaguerreDeconClass in"=w1324) -> ("error out"=w1319:errorcluster, "LaguerreDeconClass out"=w1321:refnum<class "LaguerreDeconEngineClass.lvclass">)  [unwired: 8 in]
        n591 = call "Ch2DeconEngineFGV.vi"("Error In"=w1319, "action"=enum16{"write", "read"}."write", "Ch2DeconEngine in"=w1321) -> ("Error Out"=w1318:errorcluster)  [unwired: 7 in, 1 out]
        n592 = call <vilib>:"Add State(s) to Queue__JKI_lib_State_Machine.vi"("State(s) in (\"\")"=w1339) -> ("States Out"=w1338:string)  [unwired: 14 in]
      }
      frame "DeconEngine: InitializeCh3" {
        w1364 = refnum<class "LaguerreDeconEngineClass.lvclass"> refnum  # Ch3DeconObj
        # "Initilize Laguerre Deconvolution engine Object\n(You can make a copy of, or modify, this frame)"
        n593 = call "FLImDAQ_FGV.vi"(6:enum16{"Write", "Read"}."Read" ("Operation"), "error in (no error)"=w1348) -> ("error out"=w1359:errorcluster, "Read data"=w1358:T5)  [unwired: 8 in]
        n594 = global read "GlobalVariables.vi" "LastUseiRF"() -> (w1341:T26)
        n595 = call "setLaguerreOrder.vi"("error in (no error)"=w1359, "LaguerreOrder"=u32 12, "LaguerreDeconClass in"=w1364) -> ("error out"=w1361:errorcluster, "LaguerreDeconClass out"=w1362:refnum<class "LaguerreDeconEngineClass.lvclass">)  [unwired: 7 in]
        n596 = Unbundle By Name(w1358) -> ("min record length"=w1357:i32)
        n597 = Unbundle By Name(w1341) -> ("Ch3 iRF"=w1340:dbl[])
        n598 = call "setDataLength.vi"("error in (no error)"=w1361, "dataLength"=w1357, "LaguerreDeconClass in"=w1362) -> ("error out"=w1356:errorcluster, "LaguerreDeconClass out"=w1355:refnum<class "LaguerreDeconEngineClass.lvclass">)  [unwired: 7 in]
        n599 = call "setIRF.vi"("error in (no error)"=w1356, "iRF"=w1340, "LaguerreDeconClass in"=w1355) -> ("error out"=w1353:errorcluster, "LaguerreDeconClass out"=w1354:refnum<class "LaguerreDeconEngineClass.lvclass">)  [unwired: 7 in]
        n600 = call "computeAlpha.vi"("error in (no error)"=w1353, "LaguerreDeconClass in"=w1354) -> ("error out"=w1351:errorcluster, "LaguerreDeconClass out"=w1352:refnum<class "LaguerreDeconEngineClass.lvclass">)  [unwired: 8 in]
        n601 = call "dataInitilize.vi"("error in (no error)"=w1351, "LaguerreDeconClass in"=w1352) -> ("error out"=w1349:errorcluster, "LaguerreDeconClass out"=w1350:refnum<class "LaguerreDeconEngineClass.lvclass">)  [unwired: 8 in]
        n602 = call "computeDeconMatrix.vi"("error in (no error)"=w1349, "LaguerreDeconClass in"=w1350) -> ("error out"=w1345:errorcluster, "LaguerreDeconClass out"=w1347:refnum<class "LaguerreDeconEngineClass.lvclass">)  [unwired: 8 in]
        n603 = call "Ch3DeconEngineFGV.vi"("Error In"=w1345, "action"=enum16{"write", "read"}."write", "Ch3DeconEngine in"=w1347) -> ("Error Out"=w1344:errorcluster)  [unwired: 7 in, 1 out]
        n604 = call <vilib>:"Add State(s) to Queue__JKI_lib_State_Machine.vi"("State(s) in (\"\")"=w1366) -> ("States Out"=w1365:string)  [unwired: 14 in]
      }
      frame "DeconEngine: iRFAlign" {
        # "Template Separator\n(You can make a copy of, or modify, this frame)"
        n605 = call <vilib>:"Add State(s) to Queue__JKI_lib_State_Machine.vi"("State(s) in (\"\")"=w1371) -> ("States Out"=w1370:string)  [unwired: 14 in]
      }
      frame "---------- Digitizer ----------" {
        # "Template Separator\n(You can make a copy of, or modify, this frame)"
        n606 = call <vilib>:"Add State(s) to Queue__JKI_lib_State_Machine.vi"("State(s) in (\"\")"=w1376) -> ("States Out"=w1375:string)  [unwired: 14 in]
      }
      frame "Digitizer: Initialize" {
        # "Initialize digitizer.\nInitialize both digitizer and update status."
        n607 = Unbundle By Name(w1387) -> ("SysConfigCluster.Ch1Enable?"=w1392:bool, "SysConfigCluster.Ch2Enable?"=w1391:bool, "SysConfigCluster.Ch3Enable?"=w1389:bool)
        n608 = call "FLImDAQ_FGV.vi"(6:enum16{"Write", "Read"}."Read" ("Operation"), "error in (no error)"=w1382) -> ("error out"=w1381:errorcluster, "Read data"=w1380:T5)  [unwired: 8 in]
        n609 = property on="Digitizer" class="Bool (strict)"("Blinking"=TRUE) -> ()  [unwired: 2 in, 2 out]
        n610 = Unbundle By Name(w1380) -> ("Digitizer 1"=w1379:refnum<k15>, "Digitizer 2"=w1378:refnum<k15>)
        n611 = Or(x=w1392, y=w1391) -> (x .or. y?=w1390:bool)
        n612 = case shown="True" w1389 {
          tunnel: w1381 -> [w1395 w1397]
          tunnel: [w1395 w1399] -> w1385
          tunnel: w1378 -> [_ w1398]
          frame False {
          }
          frame True {
            n613 = call <instrlib>:"niScope Initialize.vi"("resource name"=w1398, "reset device"=TRUE, "error in"=w1397) -> ("error out"=w1399:errorcluster)  [unwired: 11 in, 1 out]
          }
        }
        n614 = case shown="True" w1390 {
          tunnel: w1381 -> [w1400 w1402]
          tunnel: [w1400 w1404] -> w1386
          tunnel: w1379 -> [_ w1403]
          frame False {
          }
          frame True {
            n615 = call <instrlib>:"niScope Initialize.vi"("resource name"=w1403, "reset device"=TRUE, "error in"=w1402) -> ("error out"=w1404:errorcluster)  [unwired: 11 in, 1 out]
          }
        }
        n616 = Merge Errors(w1386, w1385) -> (w1384:errorcluster)
        n617 = call <vilib>:"Add State(s) to Queue__JKI_lib_State_Machine.vi"("State(s) in (\"\")"=w1394) -> ("States Out"=w1393:string)  [unwired: 14 in]
      }
      frame "Digitizer: Config" {
        # "Synchronize is taking time ~3s."
        # "Config  digitizer\nCall subVi to config digitizer"
        n618 = Unbundle By Name(w1434) -> ("SysConfigCluster.Ch1Enable?"=w1442:bool, "SysConfigCluster.Ch2Enable?"=w1441:bool, "SysConfigCluster.Ch3Enable?"=w1439:bool, "FLImDAQ"=w1436:T22)
        n619 = call "FLImDAQ_FGV.vi"(6:enum16{"Write", "Read"}."Read" ("Operation")) -> ("Read data"=w1424:T5)  [unwired: 9 in, 1 out]
        n620 = Unbundle By Name(w1424) -> ("Digitizer 1"=w1427:refnum<k15>, "Digitizer 2"=w1426:refnum<k15>)
        n621 = property on="Digitizer" class="Bool (strict)"(error in=w1428, "Blinking"=TRUE) -> (error out=w1430:errorcluster)  [unwired: 1 in, 1 out]
        n622 = Or(x=w1442, y=w1441) -> (x .or. y?=w1440:bool)
        n623 = case shown="True" w1440 {
          tunnel: w1436 -> [_ w1455]
          tunnel: w1430 -> [w1451 w1454]
          tunnel: [w1451 w1453] -> w1437
          tunnel: w1427 -> [_ w1452]
          frame False {
          }
          frame True {
            n624 = call "DigitizerConfig.vi"("error in (no error)"=w1454, "FLImDAQ"=w1455, "IVI Refnum in"=w1452) -> ("error out"=w1453:errorcluster)  [unwired: 7 in, 1 out]
          }
        }
        n625 = case shown="True" w1439 {
          tunnel: w1436 -> [_ w1450]
          tunnel: w1437 -> [w1445 w1449]
          tunnel: [w1445 w1448] -> w1410
          tunnel: w1426 -> [_ w1446]
          frame False {
          }
          frame True {
            n626 = call "DigitizerConfig.vi"("Config Trigge(T)r:"=FALSE, "error in (no error)"=w1449, "FLImDAQ"=w1450, "IVI Refnum in"=w1446) -> ("error out"=w1448:errorcluster)  [unwired: 6 in, 1 out]
          }
        }
        n627 = call "Digitizer1_FGV.vi"("error in (no error)"=w1410, "Operation"=enum16{"Write", "Read"}."Read") -> ("error out"=w1421:errorcluster, "Read data"=w1422:refnum<k15>)  [unwired: 8 in]
        n628 = call <instrlib>:"niScope Get Session Reference.vi"("instrument handle"=w1422, "error in"=w1421) -> ("session reference"=w1414:refnum<k20>, "error out"=w1412:errorcluster)  [unwired: 11 in, 1 out]
        n629 = call "Digitizer2_FGV.vi"("error in (no error)"=w1412, "Operation"=enum16{"Write", "Read"}."Read") -> ("error out"=w1418:errorcluster, "Read data"=w1419:refnum<k15>)  [unwired: 8 in]
        n630 = call <instrlib>:"niScope Get Session Reference.vi"("instrument handle"=w1419, "error in"=w1418) -> ("session reference"=w1413:refnum<k20>, "error out"=w1411:errorcluster)  [unwired: 11 in, 1 out]
        n631 = Build Array(w1414, w1413) -> (w1417:refnum<k20>[])
        n632 = call <instrlib>:"niTClk Configure For Homogeneous Triggers.vi"("error in (no error)"=w1411, "sessions"=w1417) -> ("error out"=w1416:errorcluster, "sessions out"=w1415:refnum<k20>[])  [unwired: 8 in]
        n633 = call <instrlib>:"niTClk Synchronize.vi"("error in (no error)"=w1416, "sessions"=w1415) -> ("error out"=w1409:errorcluster, "sessions out"=w1406:refnum<k20>[])  [unwired: 8 in]
        n634 = call <userlib>:"Wait (ms)__ogtk.vi"("error in (no error)"=w1409, "milliseconds to wait"=u32 1500) -> ("error out"=w1408:errorcluster)  [unwired: 8 in, 1 out]
        n635 = Unbundle By Name(w1408) -> ("status"=w1433:bool)
        n636 = Not(x=w1433) -> (.not. x?=w1432:bool)
        n637 = Bundle By Name(cluster=w1434, "System Status.Digitizer"=w1432, "niTClk sessions"=w1406) -> (w1435:T16)
        n638 = property on="Digitizer" class="Bool (strict)"(error in=w1408, "Blinking"=FALSE) -> (error out=w1425:errorcluster)  [unwired: 1 in, 1 out]
        n639 = call <vilib>:"Add State(s) to Queue__JKI_lib_State_Machine.vi"("State(s) in (\"\")"=w1444) -> ("States Out"=w1443:string)  [unwired: 14 in]
      }
      frame "Digitizer: Start" {
        # "send trigger to start acquisition loop"
        # "initilize aquisition"
        # "Template Separator\n(You can make a copy of, or modify, this frame)"
        n640 = Unbundle By Name(w1463) -> ("niTClk sessions"=w1462:refnum<k20>[])
        n641 = call <instrlib>:"niTClk Initiate.vi"("error in (no error)"=w1456, "sessions"=w1462) -> ("error out"=w1458:errorcluster)  [unwired: 8 in, 1 out]
        n642 = Generate User Event(priority (normal)=usereventprio."high priority", user event=w1459, event data cluster=TRUE ("event data"), error in=w1458) -> (error out=w1457:errorcluster)  [unwired: 1 out]
        n643 = call <vilib>:"Add State(s) to Queue__JKI_lib_State_Machine.vi"("State(s) in (\"\")"=w1466) -> ("States Out"=w1465:string)  [unwired: 14 in]
      }
      frame "Digitizer: Abort" {
        # "Template Separator\n(You can make a copy of, or modify, this frame)"
        n644 = call "Digitizer1_FGV.vi"("error in (no error)"=w1470, "Operation"=enum16{"Write", "Read"}."Read") -> ("error out"=w1477:errorcluster, "Read data"=w1474:refnum<k15>)  [unwired: 8 in]
        n645 = call "Digitizer2_FGV.vi"("error in (no error)"=w1470, "Operation"=enum16{"Write", "Read"}."Read") -> ("error out"=w1473:errorcluster, "Read data"=w1475:refnum<k15>)  [unwired: 8 in]
        n646 = Bundle By Name(cluster=w1467, "SysRunning?"=FALSE ("System Status")) -> (w1468:T16)
        n647 = call <instrlib>:"niScope Abort.vi"("instrument handle"=w1474, "error in"=w1477) -> ("error out"=w1479:errorcluster)  [unwired: 12 in, 1 out]
        n648 = call <instrlib>:"niScope Abort.vi"("instrument handle"=w1475, "error in"=w1473) -> ("error out"=w1478:errorcluster)  [unwired: 12 in, 1 out]
        n649 = Merge Errors(w1479, w1478) -> (w1471:errorcluster)
        n650 = call <vilib>:"Add State(s) to Queue__JKI_lib_State_Machine.vi"("State(s) in (\"\")"=w1482) -> ("States Out"=w1481:string)  [unwired: 14 in]
      }
      frame "Digitizer: checkTemp" {
        w1486 = enum16{"Write", "Read"}."Read" ("Operation")
        # "Template Separator\n(You can make a copy of, or modify, this frame)"
        n651 = call "Digitizer1_FGV.vi"("Operation"=w1486) -> ("error out"=w1488:errorcluster, "Read data"=w1489:refnum<k15>)  [unwired: 9 in]
        n652 = call "Digitizer2_FGV.vi"("Operation"=w1486) -> ("error out"=w1484:errorcluster, "Read data"=w1485:refnum<k15>)  [unwired: 9 in]
        n653 = property class="niScope"(reference=w1489, error in=w1488) -> ("Device Temperature"=→"Dig1 Temp":dbl)  [unwired: 2 out]
        n654 = property class="niScope"(reference=w1485, error in=w1484) -> ("Device Temperature"=→"Dig2 Temp":dbl)  [unwired: 2 out]
        n655 = call <vilib>:"Add State(s) to Queue__JKI_lib_State_Machine.vi"("State(s) in (\"\")"=w1494) -> ("States Out"=w1493:string)  [unwired: 14 in]
      }
      frame "Digitizer: Close" {
        # "Close Digitizer"
        n656 = call "Digitizer1_FGV.vi"("error in (no error)"=w1500, "Operation"=enum16{"Write", "Read"}."Read") -> ("error out"=w1502:errorcluster, "Read data"=w1506:refnum<k15>)  [unwired: 8 in]
        n657 = call "Digitizer2_FGV.vi"("error in (no error)"=w1500, "Operation"=enum16{"Write", "Read"}."Read") -> ("error out"=w1501:errorcluster, "Read data"=w1504:refnum<k15>)  [unwired: 8 in]
        n658 = call <instrlib>:"niScope Close.vi"("instrument handle"=w1506, "error in"=w1502) -> ("error out"=w1499:errorcluster)  [unwired: 13 in]
        n659 = call <instrlib>:"niScope Close.vi"("instrument handle"=w1504, "error in"=w1501) -> ("error out"=w1498:errorcluster)  [unwired: 13 in]
        n660 = Merge Errors(w1499, w1498) -> (w1497:errorcluster)
        n661 = Unbundle By Name(w1497) -> ("status"=w1496:bool)
        n662 = Bundle By Name(cluster=w1507, "System Status.Digitizer"=w1496) -> (w1508:T16)
        n663 = call <vilib>:"Add State(s) to Queue__JKI_lib_State_Machine.vi"("State(s) in (\"\")"=w1510) -> ("States Out"=w1509:string)  [unwired: 14 in]
      }
      frame "---------- LabJack ----------" {
        # "Template Separator\n(You can make a copy of, or modify, this frame)"
        n664 = call <vilib>:"Add State(s) to Queue__JKI_lib_State_Machine.vi"("State(s) in (\"\")"=w1515) -> ("States Out"=w1514:string)  [unwired: 14 in]
      }
      frame "LabJack: checkPedal" {
        # "Template Separator\n(You can make a copy of, or modify, this frame)"
        n665 = Unbundle By Name(w1516) -> ("LJ Pinout.Foot Pedal"=w1520:string)
        n666 = call "LabJack_FGV.vi"("Operation(Read)"=enum16{"Write", "Read"}."Read" ("Operation"), "error in (no error)"=w1518) -> ("error out"=w1522:errorcluster, "Read data"=w1523:i32)  [unwired: 8 in]
        n667 = call <vilib>:"LJM_eReadName.vi"("Handle In"=w1523, "Name"=w1520, "error in"=w1522) -> ("Value"=w1521:dbl, "error out"=w1519:errorcluster)  [unwired: 10 in, 1 out]
        n668 = case shown="1" w1521 {
          tunnel: w1516 -> [w1528 w1531]
          tunnel: [w1528 w1529] -> w1517
          frame 0, Default {
          }
          frame 1 {
            # "If Pedal pressed"
            n669 = Tick Count (ms)() -> (millisecond timer value=w1535:u32)
            n670 = Unbundle By Name(w1531) -> ("Last Trigger"=w1530:u32)
            n671 = Subtract(x=w1535, y=w1530) -> (x-y=w1534:u32)
            n672 = Greater Or Equal?(x=w1534, y=u32 2000) -> (x >= y?=w1532:bool)
            n673 = case shown="True" w1532 {
              tunnel: w1531 -> [w1536 w1537]
              tunnel: w1530 -> [_ _]
              tunnel: [w1536 w1538] -> w1529
              frame False {
              }
              frame True {
                n674 = Tick Count (ms)() -> (millisecond timer value=w1539:u32)
                n675 = Unbundle By Name(w1537) -> ("SysRunning?"=w1540:bool)
                n676 = case shown="True" w1540 {
                  frame False {
                    n677 = property on="StartButton" class="Bool (strict)"("Val(Sgnl)"=TRUE ("Value (Signaling)")) -> ()  [unwired: 2 in, 2 out]
                  }
                  frame True {
                    n678 = property on="StopButton" class="Bool (strict)"("Val(Sgnl)"=TRUE ("Value (Signaling)")) -> ()  [unwired: 2 in, 2 out]
                  }
                }
                n679 = Bundle By Name(cluster=w1537, "Last Trigger"=w1539) -> (w1538:T16)
              }
            }
          }
        }
        n680 = call <vilib>:"Add State(s) to Queue__JKI_lib_State_Machine.vi"("State(s) in (\"\")"=w1527) -> ("States Out"=w1526:string)  [unwired: 14 in]
      }
      frame "LabJack: ZeroV" {
        # "set bias to 0"
        # "Zero APD bias\n(You can make a copy of, or modify, this frame)"
        n681 = Unbundle By Name(w1558) -> ("LJ Pinout.Ch1 Bias"=w1563:string, "LJ Pinout.Ch2 Bias"=w1562:string, "LJ Pinout.Ch3 Bias"=w1561:string)
        n682 = call "V1FGV.vi"("Error In"=w1552, "action"=enum16{"write", "read"}."write", "V1 in"=0.0) -> ("Error Out"=w1551:errorcluster, "V1 out"=w1545:dbl)  [unwired: 7 in]
        n683 = Build Array(w1563, w1562, w1561) -> (w1560:string[])
        n684 = local write "Gain 1"(w1545) -> ()
        n685 = call "V2FGV.vi"("Error In"=w1551, "action"=enum16{"write", "read"}."write", "V2 in"=0.0) -> ("Error Out"=w1550:errorcluster, "V2 out"=w1544:dbl)  [unwired: 7 in]
        n686 = call "LabJack_FGV.vi"("Operation(Read)"=enum16{"Write", "Read"}."Read" ("Operation"), "error in (no error)"=w1552) -> ("error out"=w1564:errorcluster, "Read data"=w1565:i32)  [unwired: 8 in]
        n687 = local write "Gain 2"(w1544) -> ()
        n688 = call "V3FGV.vi"("Error In"=w1550, "action"=enum16{"write", "read"}."write", "V3 in"=0.0) -> ("Error Out"=w1547:errorcluster, "V3 out"=w1543:dbl)  [unwired: 7 in]
        n689 = call <vilib>:"LJM_eWriteNames.vi"("Handle In"=w1565, "aNames"=w1560, "aValuesIn"=dbl[] [0.0, 0.0, 0.0], "error in"=w1564) -> ("error out"=w1548:errorcluster)  [unwired: 9 in, 2 out]
        n690 = local write "Gain 3"(w1543) -> ()
        n691 = Merge Errors(w1547, w1548) -> (w1549:errorcluster)
        n692 = call <vilib>:"Add State(s) to Queue__JKI_lib_State_Machine.vi"("State(s) in (\"\")"=w1569) -> ("States Out"=w1568:string)  [unwired: 14 in]
      }
      frame "LabJack: Open" {
        # "Initialize LabJack T7\nEstablish connection and initialize pins"
        n693 = call "LJ_Open.vi"("error in"=w1578) -> ("error out"=w1575:errorcluster, "Success?"=w1576:bool, "Handle Out"=w1572:i32)  [unwired: 8 in]
        n694 = call "LabJack_FGV.vi"("Operation(Read)"=enum16{"Write", "Read"}."Write" ("Operation"), "error in (no error)"=w1575, "Write data"=w1572) -> ("error out"=w1571:errorcluster)  [unwired: 7 in, 1 out]
        n695 = Bundle By Name(cluster=w1573, "System Status.Labjack"=w1576) -> (w1577:T16)
        n696 = call <vilib>:"Add State(s) to Queue__JKI_lib_State_Machine.vi"("State(s) in (\"\")"=w1580) -> ("States Out"=w1579:string)  [unwired: 14 in]
      }
      frame "LabJack: SetDefaultSub" {
        w1600 = "_EF_ENABLE" ("string")
        # "1. Disable PWM\n2. Set all V to 0\n3. Set 355 relay to open\n4. Set LED to off"
        # "read once to set DIO to input"
        # "set all initila V to 0. Set footpedal to input. Set PWM to low. Set laser relay to open. Set LEDs to yellow."
        # "Set Labjack to correct input and output state and initial values"
        n697 = Unbundle By Name(w1597) -> ("LJ Pinout.355 PWM"=w1602:string, "LJ Pinout.AimingBeam PWM"=w1601:string, "LJ Pinout.Ch1 Bias"=w1609:string, "LJ Pinout.Ch2 Bias"=w1615:string, "LJ Pinout.Ch3 Bias"=w1614:string, "LJ Pinout.Laser Start/Stop"=w1613:string, "LJ Pinout.Red LED"=w1612:string, "LJ Pinout.Green LED"=w1611:string)
        n698 = call "V1FGV.vi"("Error In"=w1590, "action"=enum16{"write", "read"}."write", "V1 in"=0.0) -> ("Error Out"=w1591:errorcluster, "V1 out"=w1583:dbl)  [unwired: 7 in]
        n699 = call "LabJack_FGV.vi"("Operation(Read)"=enum16{"Write", "Read"}."Read" ("Operation"), "error in (no error)"=w1590) -> ("error out"=w1605:errorcluster, "Read data"=w1606:i32)  [unwired: 8 in]
        n700 = local write "Gain 1"(w1583) -> ()
        n701 = call "V2FGV.vi"("Error In"=w1591, "action"=enum16{"write", "read"}."write", "V2 in"=0.0) -> ("Error Out"=w1587:errorcluster, "V2 out"=w1582:dbl)  [unwired: 7 in]
        n702 = Concatenate Strings(w1602, w1600) -> (w1599:string)
        n703 = Concatenate Strings(w1601, w1600) -> (w1598:string)
        n704 = local write "Gain 2"(w1582) -> ()
        n705 = call "V3FGV.vi"("Error In"=w1587, "action"=enum16{"write", "read"}."write", "V3 in"=0.0) -> ("Error Out"=w1584:errorcluster, "V3 out"=w1581:dbl)  [unwired: 7 in]
        n706 = Build Array(w1599, w1598, w1609, w1615, w1614, w1613, w1612, w1611) -> (w1610:string[])
        n707 = Unbundle By Name(w1597) -> ("LJ Pinout.Foot Pedal"=w1596:string)
        n708 = local write "Gain 3"(w1581) -> ()
        n709 = call <vilib>:"LJM_eWriteNames.vi"("Handle In"=w1606, "aNames"=w1610, "aValuesIn"=dbl[] [0.0, 0.0, 0.0, 0.0, 0.0, 0.0, 0.0, 0.0], "error in"=w1605) -> ("Handle Out"=w1604:i32, "error out"=w1603:errorcluster)  [unwired: 9 in, 1 out]
        n710 = call <vilib>:"LJM_eReadName.vi"("Handle In"=w1604, "Name"=w1596, "error in"=w1603) -> ("error out"=w1586:errorcluster)  [unwired: 10 in, 2 out]
        n711 = Merge Errors(w1586, w1584) -> (w1585:errorcluster)
        n712 = call <vilib>:"Add State(s) to Queue__JKI_lib_State_Machine.vi"("State(s) in (\"\")"=w1618) -> ("States Out"=w1617:string)  [unwired: 14 in]
      }
      frame "LabJack: FootPedalConfig" {
        # "Setup footPedal\n(You can make a copy of, or modify, this frame)"
        n713 = call "LabJack_FGV.vi"("Operation(Read)"=enum16{"Write", "Read"}."Read" ("Operation"), "error in (no error)"=w1620) -> ("error out"=w1624:errorcluster, "Read data"=w1625:i32)  [unwired: 8 in]
        n714 = call <vilib>:"LJM_eWriteName.vi"("Handle In"=w1625, "Name"="DIO15", "Value"=1.0, "error in"=w1624) -> ("error out"=w1621:errorcluster)  [unwired: 10 in, 1 out]
        n715 = call <vilib>:"Add State(s) to Queue__JKI_lib_State_Machine.vi"("State(s) in (\"\")"=w1629) -> ("States Out"=w1628:string)  [unwired: 14 in]
      }
      frame "LabJack: SetDefaultAndClose" {
        # "Template Separator\n(You can make a copy of, or modify, this frame)"
        n716 = call <vilib>:"Add State(s) to Queue__JKI_lib_State_Machine.vi"("State(s) in Front (\"\")"="LabJack: SetDefaultSub\nLabJack: Close" ("State(s) in Front (\"\")"), "State(s) in (\"\")"=w1635) -> ("States Out"=w1634:string)  [unwired: 13 in]
      }
      frame "LabJack: Close" {
        # "Close LabJack Refnum"
        n717 = call "LabJack_FGV.vi"("Operation(Read)"=enum16{"Write", "Read"}."Read" ("Operation"), "error in (no error)"=w1641) -> ("error out"=w1636:errorcluster, "Read data"=w1637:i32)  [unwired: 8 in]
        n718 = Bundle By Name(cluster=w1639, "System Status.Labjack"=FALSE ("System Status.Gain Control")) -> (w1642:T16)
        n719 = call <vilib>:"LJM_Close.vi"("error in"=w1636, "Handle"=w1637) -> ("error out"=w1644:errorcluster)  [unwired: 9 in]
        n720 = call <vilib>:"Add State(s) to Queue__JKI_lib_State_Machine.vi"("State(s) in (\"\")"=w1646) -> ("States Out"=w1645:string)  [unwired: 14 in]
      }
      frame "LabJack: Interlock enable/disable" {
        w1655 = i8 0  # int8
        # "Interlock enable/disable\n(Usage: \"LabJack: Interlock enable/disable >> 1|0\")"
        n721 = Fract/Exp String To Number(string=w1656, default (0 dbl)=w1655) -> (number=w1652:i8)  [unwired: 2 in, 1 out]
        n722 = Unbundle By Name(w1654) -> ("LJ Pinout.Interlock"=w1653:string)
        n723 = call "LabJack_FGV.vi"("Operation(Read)"=enum16{"Write", "Read"}."Read" ("Operation")) -> ("Read data"=w1650:i32)  [unwired: 9 in, 1 out]
        n724 = call <vilib>:"LJM_eWriteName.vi"("Handle In"=w1650, "Name"=w1653, "Value"=w1652, "error in"=w1651) -> ("error out"=w1648:errorcluster)  [unwired: 10 in, 1 out]
        n725 = call <vilib>:"Add State(s) to Queue__JKI_lib_State_Machine.vi"("State(s) in (\"\")"=w1658) -> ("States Out"=w1657:string)  [unwired: 14 in]
      }
      frame "LabJack: 355_PWM_Config" {
        w1660 = 0.0 ("element")
        w1680 = "DIO_EF_CLOCK1_ENABLE"
        # "Config PWM frequency"
        n726 = Unbundle By Name(w1672) -> ("355 PWM setting.DIO_EF_CLOCK1_DIVISOR"=w1671:i16, "355 PWM setting.DIO_EF_CLOCK1_ROLL_VALUE"=w1670:i32, "355 PWM setting.DIO#_EF_INDEX"=w1667:i16, "355 PWM setting.DIO#_EF_OPTIONS"=w1666:i16, "355 PWM setting.DIO#_EF_CONFIG_A"=w1665:i32)
        n727 = Unbundle By Name(w1672) -> ("LJ Pinout.355 PWM"=w1679:string)
        n728 = Concatenate Strings(w1679, "_EF_ENABLE" ("string")) -> (w1675:string)
        n729 = Concatenate Strings(w1679, "_EF_INDEX") -> (w1678:string)
        n730 = Concatenate Strings(w1679, "_EF_OPTIONS") -> (w1677:string)
        n731 = Concatenate Strings(w1679, "_EF_CONFIG_A") -> (w1676:string)
        n732 = call "LabJack_FGV.vi"("Operation(Read)"=enum16{"Write", "Read"}."Read" ("Operation")) -> ("Read data"=w1673:i32)  [unwired: 9 in, 1 out]
        n733 = Build Array(w1660, w1660, w1671, w1670, 1.0 ("element"), 0.0 ("element"), w1667, w1666, w1665) -> (w1664:dbl[])
        n734 = Build Array("DIO_EF_CLOCK0_ENABLE", w1680, "DIO_EF_CLOCK1_DIVISOR", "DIO_EF_CLOCK1_ROLL_VALUE", w1680, w1675, w1678, w1677, w1676) -> (w1674:string[])
        n735 = call <vilib>:"LJM_eWriteNames.vi"("Handle In"=w1673, "aNames"=w1674, "aValuesIn"=w1664, "error in"=w1662) -> ("error out"=w1663:errorcluster)  [unwired: 9 in, 2 out]
        n736 = call <vilib>:"Add State(s) to Queue__JKI_lib_State_Machine.vi"("State(s) in (\"\")"=w1689) -> ("States Out"=w1688:string)  [unwired: 14 in]
      }
      frame "LabJack: AB_PWM_Config" {
        w1691 = 0.0 ("element")
        w1711 = "DIO_EF_CLOCK2_ENABLE"
        # "Config PWM frequency"
        n737 = Unbundle By Name(w1703) -> ("LJ Pinout.AimingBeam PWM"=w1710:string)
        n738 = Unbundle By Name(w1703) -> ("AB PWM setting.DIO_EF_CLOCK1_DIVISOR"=w1702:i16, "AB PWM setting.DIO_EF_CLOCK1_ROLL_VALUE"=w1701:i32, "AB PWM setting.DIO#_EF_INDEX"=w1698:i16, "AB PWM setting.DIO#_EF_OPTIONS"=w1697:i16, "AB PWM setting.DIO#_EF_CONFIG_A"=w1696:i32)
        n739 = Concatenate Strings(w1710, "_EF_ENABLE" ("string")) -> (w1706:string)
        n740 = Concatenate Strings(w1710, "_EF_INDEX") -> (w1709:string)
        n741 = Concatenate Strings(w1710, "_EF_OPTIONS") -> (w1708:string)
        n742 = Concatenate Strings(w1710, "_EF_CONFIG_A") -> (w1707:string)
        n743 = call "LabJack_FGV.vi"("Operation(Read)"=enum16{"Write", "Read"}."Read" ("Operation")) -> ("Read data"=w1704:i32)  [unwired: 9 in, 1 out]
        n744 = Build Array(w1691, w1691, w1702, w1701, 1.0 ("element"), 0.0 ("element"), w1698, w1697, w1696) -> (w1695:dbl[])
        n745 = Build Array("DIO_EF_CLOCK0_ENABLE", w1711, "DIO_EF_CLOCK2_DIVISOR", "DIO_EF_CLOCK2_ROLL_VALUE", w1711, w1706, w1709, w1708, w1707) -> (w1705:string[])
        n746 = call <vilib>:"LJM_eWriteNames.vi"("Handle In"=w1704, "aNames"=w1705, "aValuesIn"=w1695, "error in"=w1693) -> ("error out"=w1694:errorcluster)  [unwired: 9 in, 2 out]
        n747 = call <vilib>:"Add State(s) to Queue__JKI_lib_State_Machine.vi"("State(s) in (\"\")"=w1720) -> ("States Out"=w1719:string)  [unwired: 14 in]
      }
      frame "LabJack: 355_PWM_Start" {
        # "Template Separator\n(You can make a copy of, or modify, this frame)"
        n748 = Unbundle By Name(w1728) -> ("LJ Pinout.355 PWM"=w1727:string)
        n749 = call "LabJack_FGV.vi"("Operation(Read)"=enum16{"Write", "Read"}."Read" ("Operation"), "error in (no error)"=w1722) -> ("error out"=w1729:errorcluster, "Read data"=w1730:i32)  [unwired: 8 in]
        n750 = Concatenate Strings(w1727, "_EF_ENABLE" ("string")) -> (w1725:string)
        n751 = call <vilib>:"LJM_eWriteName.vi"("Handle In"=w1730, "Name"=w1725, "Value"=1.0, "error in"=w1729) -> ("error out"=w1723:errorcluster)  [unwired: 10 in, 1 out]
        n752 = call <vilib>:"Add State(s) to Queue__JKI_lib_State_Machine.vi"("State(s) in (\"\")"=w1733) -> ("States Out"=w1732:string)  [unwired: 14 in]
      }
      frame "LabJack: AB_PWM_Start" {
        # "Template Separator\n(You can make a copy of, or modify, this frame)"
        n753 = Unbundle By Name(w1741) -> ("LJ Pinout.AimingBeam PWM"=w1740:string)
        n754 = call "LabJack_FGV.vi"("Operation(Read)"=enum16{"Write", "Read"}."Read" ("Operation"), "error in (no error)"=w1735) -> ("error out"=w1742:errorcluster, "Read data"=w1743:i32)  [unwired: 8 in]
        n755 = Concatenate Strings(w1740, "_EF_ENABLE" ("string")) -> (w1738:string)
        n756 = call <vilib>:"LJM_eWriteName.vi"("Handle In"=w1743, "Name"=w1738, "Value"=1.0, "error in"=w1742) -> ("error out"=w1736:errorcluster)  [unwired: 10 in, 1 out]
        n757 = call <vilib>:"Add State(s) to Queue__JKI_lib_State_Machine.vi"("State(s) in (\"\")"=w1746) -> ("States Out"=w1745:string)  [unwired: 14 in]
      }
      frame "LabJack: 355_PWM_Stop" {
        # "Template Separator\n(You can make a copy of, or modify, this frame)"
        n758 = Unbundle By Name(w1752) -> ("LJ Pinout.355 PWM"=w1756:string)
        n759 = call "LabJack_FGV.vi"("Operation(Read)"=enum16{"Write", "Read"}."Read" ("Operation"), "error in (no error)"=w1750) -> ("error out"=w1757:errorcluster, "Read data"=w1748:i32)  [unwired: 8 in]
        n760 = Concatenate Strings(w1756, "_EF_ENABLE" ("string")) -> (w1754:string)
        n761 = call <vilib>:"LJM_eWriteName.vi"("Handle In"=w1748, "Name"=w1754, "Value"=0.0, "error in"=w1757) -> ("error out"=w1751:errorcluster)  [unwired: 10 in, 1 out]
        n762 = local write "355nm Laser toggle"(FALSE ("355nm Laser toggle")) -> ()
        n763 = call <vilib>:"Add State(s) to Queue__JKI_lib_State_Machine.vi"("State(s) in (\"\")"=w1760) -> ("States Out"=w1759:string)  [unwired: 14 in]
      }
      frame "LabJack: AB_PWM_Stop" {
        # "Template Separator\n(You can make a copy of, or modify, this frame)"
        n764 = Unbundle By Name(w1765) -> ("LJ Pinout.AimingBeam PWM"=w1769:string)
        n765 = call "LabJack_FGV.vi"("Operation(Read)"=enum16{"Write", "Read"}."Read" ("Operation"), "error in (no error)"=w1763) -> ("error out"=w1770:errorcluster, "Read data"=w1771:i32)  [unwired: 8 in]
        n766 = Concatenate Strings(w1769, "_EF_ENABLE" ("string")) -> (w1767:string)
        n767 = call <vilib>:"LJM_eWriteName.vi"("Handle In"=w1771, "Name"=w1767, "Value"=0.0, "error in"=w1770) -> ("error out"=w1764:errorcluster)  [unwired: 10 in, 1 out]
        n768 = local write "Aiming beam toggle"(FALSE ("Aiming beam toggle")) -> ()
        n769 = call <vilib>:"Add State(s) to Queue__JKI_lib_State_Machine.vi"("State(s) in (\"\")"=w1774) -> ("States Out"=w1773:string)  [unwired: 14 in]
      }
      frame "---------- LED ----------" {
        # "Template Separator\n(You can make a copy of, or modify, this frame)"
        n770 = call <vilib>:"Add State(s) to Queue__JKI_lib_State_Machine.vi"("State(s) in (\"\")"=w1779) -> ("States Out"=w1778:string)  [unwired: 14 in]
      }
      frame "LED: OpenVIRef" {
        w1785 = path "C:/Users/IntuitiveA/Desktop/V6 APD LV/SubVI/LEDBreath.vi"  # vi path
        # "Template Separator\n(You can make a copy of, or modify, this frame)"
        n771 = Open VI Reference(vi path=w1785, error in (no error)=w1780) -> (vi reference=w1782:refnum<vi>, error out=w1781:errorcluster)  [unwired: 4 in]
        n772 = Bundle By Name(cluster=w1783, "LED vi reference"=w1782) -> (w1784:T16)
        n773 = call <vilib>:"Add State(s) to Queue__JKI_lib_State_Machine.vi"("State(s) in (\"\")"=w1788) -> ("States Out"=w1787:string)  [unwired: 14 in]
      }
      frame "LED: CloseVIRef" {
        # "Template Separator\n(You can make a copy of, or modify, this frame)"
        n774 = Unbundle By Name(w1789) -> ("LED vi reference"=w1790:refnum<vi>)
        n775 = Close Reference(reference=w1790, error in (no error)=w1792) -> (error out=w1791:errorcluster)
        n776 = call <vilib>:"Add State(s) to Queue__JKI_lib_State_Machine.vi"("State(s) in (\"\")"=w1795) -> ("States Out"=w1794:string)  [unwired: 14 in]
      }
      frame "LED: Breath" {
        # "Breath system LED\n(LED: Breath >> True/False)"
        n777 = Unbundle By Name(w1800) -> ("LED vi reference"=w1799:refnum<vi>)
        n778 = case shown="\"False\", Default" w1796 {
          tunnel: w1799 -> [w1808 w1812]
          tunnel: [w1806 w1810] -> w1798
          tunnel: w1797 -> [w1807 w1809]
          frame "False", Default {
            n779 = invoke class="VI" method="Ctrl Val.Set"(reference=w1808, error in=w1807, "Control Name"="Stop", "Value"=TRUE) -> (error out=w1806:errorcluster)  [unwired: 1 in, 4 out]
          }
          frame "True" {
            n780 = invoke class="VI" method="Run VI"(reference=w1812, error in=w1809, "Wait until done"=FALSE ("Wait Until Done"), "Auto Dispose Ref"=FALSE ("Auto Dispose Reference")) -> (error out=w1810:errorcluster)  [unwired: 1 in, 4 out]
          }
        }
        n781 = call <vilib>:"Add State(s) to Queue__JKI_lib_State_Machine.vi"("State(s) in (\"\")"=w1803) -> ("States Out"=w1802:string)  [unwired: 14 in]
      }
      frame "LED: Off" {
        # "set LED to red"
        # "Template Separator\n(You can make a copy of, or modify, this frame)"
        n782 = Unbundle By Name(w1816) -> ("LJ Pinout.Red LED"=w1815:string, "LJ Pinout.Green LED"=w1814:string)
        n783 = call "LabJack_FGV.vi"("Operation(Read)"=enum16{"Write", "Read"}."Read" ("Operation"), "error in (no error)"=w1817) -> ("error out"=w1824:errorcluster, "Read data"=w1823:i32)  [unwired: 8 in]
        n784 = call <vilib>:"LJM_eWriteName.vi"("Handle In"=w1823, "Name"=w1815, "Value"=0.0, "error in"=w1824) -> ("Handle Out"=w1821:i32, "error out"=w1820:errorcluster)  [unwired: 10 in]
        n785 = call <vilib>:"LJM_eWriteName.vi"("Handle In"=w1821, "Name"=w1814, "Value"=0.0, "error in"=w1820) -> ("error out"=w1818:errorcluster)  [unwired: 10 in, 1 out]
        n786 = call <vilib>:"Add State(s) to Queue__JKI_lib_State_Machine.vi"("State(s) in (\"\")"=w1828) -> ("States Out"=w1827:string)  [unwired: 14 in]
      }
      frame "LED: Red" {
        # "set LED to red"
        # "Template Separator\n(You can make a copy of, or modify, this frame)"
        n787 = Unbundle By Name(w1831) -> ("LJ Pinout.Red LED"=w1830:string, "LJ Pinout.Green LED"=w1829:string)
        n788 = call "LabJack_FGV.vi"("Operation(Read)"=enum16{"Write", "Read"}."Read" ("Operation"), "error in (no error)"=w1832) -> ("error out"=w1839:errorcluster, "Read data"=w1838:i32)  [unwired: 8 in]
        n789 = call <vilib>:"LJM_eWriteName.vi"("Handle In"=w1838, "Name"=w1830, "Value"=9.0, "error in"=w1839) -> ("Handle Out"=w1836:i32, "error out"=w1835:errorcluster)  [unwired: 10 in]
        n790 = call <vilib>:"LJM_eWriteName.vi"("Handle In"=w1836, "Name"=w1829, "Value"=0.0, "error in"=w1835) -> ("error out"=w1833:errorcluster)  [unwired: 10 in, 1 out]
        n791 = call <vilib>:"Add State(s) to Queue__JKI_lib_State_Machine.vi"("State(s) in (\"\")"=w1843) -> ("States Out"=w1842:string)  [unwired: 14 in]
      }
      frame "LED: Green" {
        # "set LED to green"
        # "Template Separator\n(You can make a copy of, or modify, this frame)"
        n792 = Unbundle By Name(w1847) -> ("LJ Pinout.Red LED"=w1845:string, "LJ Pinout.Green LED"=w1846:string)
        n793 = call "LabJack_FGV.vi"("Operation(Read)"=enum16{"Write", "Read"}."Read" ("Operation"), "error in (no error)"=w1849) -> ("error out"=w1855:errorcluster, "Read data"=w1854:i32)  [unwired: 8 in]
        n794 = call <vilib>:"LJM_eWriteName.vi"("Handle In"=w1854, "Name"=w1845, "Value"=0.0, "error in"=w1855) -> ("Handle Out"=w1852:i32, "error out"=w1851:errorcluster)  [unwired: 10 in]
        n795 = call <vilib>:"LJM_eWriteName.vi"("Handle In"=w1852, "Name"=w1846, "Value"=9.0, "error in"=w1851) -> ("error out"=w1848:errorcluster)  [unwired: 10 in, 1 out]
        n796 = call <vilib>:"Add State(s) to Queue__JKI_lib_State_Machine.vi"("State(s) in (\"\")"=w1858) -> ("States Out"=w1857:string)  [unwired: 14 in]
      }
      frame "LED: Yellow" {
        # "set LED to yellow"
        # "set LED to yellow\n(You can make a copy of, or modify, this frame)"
        n797 = Unbundle By Name(w1862) -> ("LJ Pinout.Red LED"=w1860:string, "LJ Pinout.Green LED"=w1861:string)
        n798 = call "LabJack_FGV.vi"("Operation(Read)"=enum16{"Write", "Read"}."Read" ("Operation"), "error in (no error)"=w1864) -> ("error out"=w1870:errorcluster, "Read data"=w1869:i32)  [unwired: 8 in]
        n799 = call <vilib>:"LJM_eWriteName.vi"("Handle In"=w1869, "Name"=w1860, "Value"=9.0, "error in"=w1870) -> ("Handle Out"=w1867:i32, "error out"=w1866:errorcluster)  [unwired: 10 in]
        n800 = call <vilib>:"LJM_eWriteName.vi"("Handle In"=w1867, "Name"=w1861, "Value"=9.0, "error in"=w1866) -> ("error out"=w1863:errorcluster)  [unwired: 10 in, 1 out]
        n801 = call <vilib>:"Add State(s) to Queue__JKI_lib_State_Machine.vi"("State(s) in (\"\")"=w1873) -> ("States Out"=w1872:string)  [unwired: 14 in]
      }
      frame "---------- Queue ----------" {
        # "Template Separator\n(You can make a copy of, or modify, this frame)"
        n802 = call <vilib>:"Add State(s) to Queue__JKI_lib_State_Machine.vi"("State(s) in (\"\")"=w1878) -> ("States Out"=w1877:string)  [unwired: 14 in]
      }
      frame "Queue: Create" {
        # "Template Separator\n(You can make a copy of, or modify, this frame)"
        n803 = call <vilib>:"Add State(s) to Queue__JKI_lib_State_Machine.vi"("State(s) in (\"\")"=w1883) -> ("States Out"=w1882:string)  [unwired: 14 in]
      }
      frame "Queue: Flash" {
        # "Clear queue contnet\n(clear queue content by flash it)"
        n804 = Flush Queue(queue=w1887, error in (no error)=w1886) -> (error out=w1885:errorcluster)  [unwired: 2 out]
        n805 = Flush Queue(queue=w1888, error in (no error)=w1885) -> (error out=w1884:errorcluster)  [unwired: 2 out]
        n806 = call <vilib>:"Add State(s) to Queue__JKI_lib_State_Machine.vi"("State(s) in (\"\")"=w1892) -> ("States Out"=w1891:string)  [unwired: 14 in]
      }
      frame "Queue: Destory" {
        # "Destory Data Queue\nDistory data queue ref so the aquisition loop stop"
        n807 = Release Queue(queue=w1898, error in (no error)=w1894) -> (error out=w1901:errorcluster)  [unwired: 1 in, 2 out]
        n808 = Release Queue(queue=w1897, error in (no error)=w1894) -> (error out=w1900:errorcluster)  [unwired: 1 in, 2 out]
        n809 = Release Queue(queue=w1895, error in (no error)=w1894) -> (error out=w1893:errorcluster)  [unwired: 1 in, 2 out]
        n810 = Merge Errors(w1901, w1900, w1893) -> (w1899:errorcluster)
        n811 = call <vilib>:"Simple Error Handler.vi"("error in (no error)"=w1899) -> ()  [unwired: 4 in, 5 out]
        n812 = call <vilib>:"Add State(s) to Queue__JKI_lib_State_Machine.vi"("State(s) in (\"\")"=w1904) -> ("States Out"=w1903:string)  [unwired: 14 in]
      }
      frame "---------- Run ----------" {
        # "Template Separator\n(You can make a copy of, or modify, this frame)"
        n813 = call <vilib>:"Add State(s) to Queue__JKI_lib_State_Machine.vi"("State(s) in (\"\")"=w1909) -> ("States Out"=w1908:string)  [unwired: 14 in]
      }
      frame "Run: CaliIncrement" {
        # "Increment Calibration #\n(You can make a copy of, or modify, this frame)"
        n814 = Unbundle By Name(w1911) -> ("IDs.Cali ID"=w1913:i8)
        n815 = Increment(x=w1913) -> (x+1=w1910:i8)
        n816 = Bundle By Name(cluster=w1911, "IDs.Cali ID"=w1910) -> (w1912:T16)
        n817 = call <vilib>:"Add State(s) to Queue__JKI_lib_State_Machine.vi"("State(s) in (\"\")"=w1917) -> ("States Out"=w1916:string)  [unwired: 14 in]
      }
      frame "Run: BGIncrement" {
        # "Increment BG #\n(You can make a copy of, or modify, this frame)"
        n818 = Unbundle By Name(w1918) -> ("IDs.BG ID"=w1921:i8)
        n819 = Increment(x=w1921) -> (x+1=w1920:i8)
        n820 = Bundle By Name(cluster=w1918, "IDs.BG ID"=w1920) -> (w1919:T16)
        n821 = call <vilib>:"Add State(s) to Queue__JKI_lib_State_Machine.vi"("State(s) in (\"\")"=w1925) -> ("States Out"=w1924:string)  [unwired: 14 in]
      }
      frame "Run: Increment" {
        # "Increase Run# by 1"
        n822 = Unbundle By Name(w1928) -> ("IDs.RunID"=w1930:i8)
        n823 = Increment(x=w1930) -> (x+1=w1927:i8)
        n824 = Bundle By Name(cluster=w1928, "IDs.RunID"=w1927) -> (w1929:T16)
        n825 = call <vilib>:"Add State(s) to Queue__JKI_lib_State_Machine.vi"("State(s) in (\"\")"=w1933) -> ("States Out"=w1932:string)  [unwired: 14 in]
      }
      frame "Run: Decrement" {
        # "Increase Run# by 1"
        n826 = Unbundle By Name(w1936) -> ("IDs.RunID"=w1938:i8)
        n827 = Decrement(x=w1938) -> (x-1=w1935:i8)
        n828 = Bundle By Name(cluster=w1936, "IDs.RunID"=w1935) -> (w1937:T16)
        n829 = call <vilib>:"Add State(s) to Queue__JKI_lib_State_Machine.vi"("State(s) in (\"\")"=w1941) -> ("States Out"=w1940:string)  [unwired: 14 in]
      }
      frame "---------- SysConfig ----------" {
        # "Template Separator\n(You can make a copy of, or modify, this frame)"
        n830 = call <vilib>:"Add State(s) to Queue__JKI_lib_State_Machine.vi"("State(s) in (\"\")"=w1946) -> ("States Out"=w1945:string)  [unwired: 14 in]
      }
      frame "SysConfig: Load Sys Config" {
        # "Load System config"
        # "Load system configuration\n(Load both hardware and DAQ config)"
        n831 = call "LoadSysConfig.vi"("Error In"=w1949, "Enum"=enum16{"LastUse", "Default"}."LastUse") -> ("Error Out"=w1948:errorcluster, "SysConfigCluster"=w1951:T3)  [unwired: 8 in]
        "SysConfigCluster" <- w1951
        n832 = Bundle By Name(cluster=w1952, "SysConfigCluster"=w1951) -> (w1953:T16)
        n833 = call <vilib>:"Add State(s) to Queue__JKI_lib_State_Machine.vi"("State(s) in (\"\")"=w1955) -> ("States Out"=w1954:string)  [unwired: 14 in]
      }
      frame "SysConfig: Load Digitizer Setting" {
        w1962 = enum16{"Write", "Read"}."Write" ("Operation")
        # "Load DAQ config\nSave to FGV"
        # "Template Separator\n(You can make a copy of, or modify, this frame)"
        n834 = call <userlib>:"Current VIs Parent Directory__ogtk.vi"() -> ("Parent Directory (+ Relative)"=w1969:path)  [unwired: 5 in]
        n835 = Build Path(base path=w1969, name or relative path="SubVI\\DigitizerConfiguration\\V6_Scope_last_use.config") -> (appended path=w1970:path)
        n836 = call "ReadDigitizerConfig(SubVI).vi"("error in (no error)"=w1967, "appended path"=w1970) -> ("error out"=w1961:errorcluster, "FLImDAQ"=w1959:T5)  [unwired: 8 in]
        n837 = call "FLImDAQ_FGV.vi"(6:w1962, "error in (no error)"=w1961, "Write data"=w1959) -> ("error out"=w1965:errorcluster)  [unwired: 7 in, 1 out]
        n838 = Bundle By Name(cluster=w1957, "FLImDAQ"=w1959) -> (w1958:T16)
        n839 = Unbundle By Name(w1959) -> ("Digitizer 1"=w1963:refnum<k15>, "Digitizer 2"=w1964:refnum<k15>)
        n840 = call "Digitizer1_FGV.vi"("error in (no error)"=w1965, "Operation"=w1962, "Write data"=w1963) -> ("error out"=w1966:errorcluster)  [unwired: 7 in, 1 out]
        n841 = call "Digitizer2_FGV.vi"("error in (no error)"=w1966, "Operation"=w1962, "Write data"=w1964) -> ("error out"=w1960:errorcluster)  [unwired: 7 in, 1 out]
        n842 = call <vilib>:"Add State(s) to Queue__JKI_lib_State_Machine.vi"("State(s) in (\"\")"=w1972) -> ("States Out"=w1971:string)  [unwired: 14 in]
      }
      frame "SysConfig: Load LJ Pinout" {
        # "Template Separator\n(You can make a copy of, or modify, this frame)"
        n843 = call <userlib>:"Current VIs Parent Directory__ogtk.vi"() -> ("Parent Directory (+ Relative)"=w1986:path)  [unwired: 5 in]
        n844 = Build Path(base path=w1986, name or relative path="SubVI\\LabJack\\LJ_pin_setting.config") -> (appended path=w1984:path)
        n845 = call "ReadLabjackConfig(SubVI).vi"("error in (no error)"=w1982, "appended path"=w1984) -> ("error out"=w1983:errorcluster, "Utility"=w1980:T4)  [unwired: 8 in]
        n846 = Unbundle By Name(w1980) -> ("Ch1 Bias"=w1979:string, "Ch2 Bias"=w1978:string, "Ch3 Bias"=w1977:string, "Red LED"=w1974:string, "Green LED"=w1973:string)
        n847 = global write "GlobalVariables.vi" "LED Green pin"(w1973) -> ()
        n848 = global write "GlobalVariables.vi" "LED Red pin"(w1974) -> ()
        n849 = global write "GlobalVariables.vi" "Ch1 LJ pin"(w1979) -> ()
        n850 = global write "GlobalVariables.vi" "Ch2 LJ pin"(w1978) -> ()
        n851 = global write "GlobalVariables.vi" "Ch3 LJ pin"(w1977) -> ()
        n852 = Bundle By Name(cluster=w1975, "LJ Pinout"=w1980) -> (w1981:T16)
        n853 = call <vilib>:"Add State(s) to Queue__JKI_lib_State_Machine.vi"("State(s) in (\"\")"=w1988) -> ("States Out"=w1987:string)  [unwired: 14 in]
      }
      frame "SysConfig: Load 355 PWM" {
        # "Template Separator\n(You can make a copy of, or modify, this frame)"
        n854 = call <userlib>:"Current VIs Parent Directory__ogtk.vi"() -> ("Parent Directory (+ Relative)"=w2006:path)  [unwired: 5 in]
        n855 = Build Path(base path=w2006, name or relative path="SubVI\\LabJack\\PWM_setting_355.config") -> (appended path=w2004:path)
        n856 = call "ReadPWMConfig(SubVI).vi"("error in (no error)"=w2001, "appended path"=w2004) -> ("error out"=w2002:errorcluster, "PWM Setting"=w2000:T27)  [unwired: 8 in]
        n857 = Unbundle By Name(w2000) -> ("DIO_EF_CLOCK1_DIVISOR"=w1997:i16, "DIO_EF_CLOCK1_ROLL_VALUE"=w1996:i32)
        n858 = Multiply(x=w1997, y=w1996) -> (x*y=w1998:i32)
        n859 = Bundle By Name(cluster=w2003, "355 PWM setting"=w2000) -> (w1990:T16)
        n860 = Divide(x=80000000.0, y=w1998) -> (x/y=w1995:dbl)
        n861 = Number To Decimal String(number=w1995) -> (decimal integer string=w1994:string)  [unwired: 1 in]
        n862 = Concatenate Strings("355nm " ("string"), w1994, "Hz" ("string")) -> (w1992:string)
        n863 = property on="355nm Laser toggle" class="Bool (strict)"("Caption.Text"=w1992) -> ()  [unwired: 2 in, 2 out]
        n864 = call <vilib>:"Add State(s) to Queue__JKI_lib_State_Machine.vi"("State(s) in (\"\")"=w2008) -> ("States Out"=w2007:string)  [unwired: 14 in]
      }
      frame "SysConfig: Load AB PWM" {
        # "Template Separator\n(You can make a copy of, or modify, this frame)"
        n865 = call <userlib>:"Current VIs Parent Directory__ogtk.vi"() -> ("Parent Directory (+ Relative)"=w2027:path)  [unwired: 5 in]
        n866 = Build Path(base path=w2027, name or relative path="SubVI\\LabJack\\PWM_setting_AB.config") -> (appended path=w2025:path)
        n867 = call "ReadPWMConfig(SubVI).vi"("error in (no error)"=w2022, "appended path"=w2025) -> ("error out"=w2023:errorcluster, "PWM Setting"=w2021:T27)  [unwired: 8 in]
        n868 = Unbundle By Name(w2021) -> ("DIO_EF_CLOCK1_DIVISOR"=w2018:i16, "DIO_EF_CLOCK1_ROLL_VALUE"=w2017:i32)
        n869 = Multiply(x=w2018, y=w2017) -> (x*y=w2019:i32)
        n870 = Bundle By Name(cluster=w2011, "AB PWM setting"=w2021) -> (w2024:T16)
        n871 = Divide(x=80000000.0, y=w2019) -> (x/y=w2016:dbl)
        n872 = Number To Decimal String(number=w2016, width (-)=i16 2) -> (decimal integer string=w2015:string)
        n873 = Concatenate Strings("445nm " ("string"), w2015, "Hz " ("string")) -> (w2013:string)
        n874 = property on="Aiming beam toggle" class="Bool (strict)"("Caption.Text"=w2013) -> ()  [unwired: 2 in, 2 out]
        n875 = call <vilib>:"Add State(s) to Queue__JKI_lib_State_Machine.vi"("State(s) in (\"\")"=w2029) -> ("States Out"=w2028:string)  [unwired: 14 in]
      }
      frame "SysConfig: Load AB setting" {
        # "Template Separator\n(You can make a copy of, or modify, this frame)"
        n876 = call "ReadAimingBeamSetting.vi"("error in (no error)"=w2031) -> ("error out"=w2032:errorcluster, "Aiming Beam Setting"=w2033:T28)  [unwired: 9 in]
        n877 = Bundle By Name(cluster=w2034, "AB Cluster"=w2033) -> (w2035:T16)
        n878 = call <vilib>:"Add State(s) to Queue__JKI_lib_State_Machine.vi"("State(s) in (\"\")"=w2037) -> ("States Out"=w2036:string)  [unwired: 14 in]
      }
      frame "---------- SystemStatus ----------" {
        # "Template Separator\n(You can make a copy of, or modify, this frame)"
        n879 = call <vilib>:"Add State(s) to Queue__JKI_lib_State_Machine.vi"("State(s) in (\"\")"=w2042) -> ("States Out"=w2041:string)  [unwired: 14 in]
      }
      frame "SystemStatus: SlowSysStatusMacro" {
        # "store system check time"
        # "Template Separator\n(You can make a copy of, or modify, this frame)"
        n880 = Tick Count (ms)() -> (millisecond timer value=w2045:u32)
        n881 = Bundle By Name(cluster=w2043, "SlowTimer"=w2045) -> (w2044:T16)
        n882 = call <vilib>:"Add State(s) to Queue__JKI_lib_State_Machine.vi"("State(s) in Front (\"\")"="Digitizer: checkTemp\nTCP: CheckConnection" ("State(s) in Front (\"\")"), "State(s) in (\"\")"=w2050) -> ("States Out"=w2049:string)  [unwired: 13 in]
      }
      frame "SystemStatus: FastSysStatusMacro" {
        # "store system check time"
        # "Template Separator\n(You can make a copy of, or modify, this frame)"
        n883 = Tick Count (ms)() -> (millisecond timer value=w2053:u32)
        n884 = Bundle By Name(cluster=w2051, "FastTimer"=w2053) -> (w2052:T16)
        n885 = call <vilib>:"Add State(s) to Queue__JKI_lib_State_Machine.vi"("State(s) in Front (\"\")"="355 Laser: CheckPWMStatus\nAimingBeam: GetPWMStatus\n" ("State(s) in Front (\"\")"), "State(s) in (\"\")"=w2058) -> ("States Out"=w2057:string)  [unwired: 13 in]
      }
      frame "---------- TCP ----------" {
        # "Template Separator\n(You can make a copy of, or modify, this frame)"
        n886 = call <vilib>:"Add State(s) to Queue__JKI_lib_State_Machine.vi"("State(s) in (\"\")"=w2063) -> ("States Out"=w2062:string)  [unwired: 14 in]
      }
      frame "TCP: Initialize" {
        # "Initialize TCP connection to aimging beam computer\n(You can make a copy of, or modify, this frame)"
        n887 = call <vilib>:"TCP Listen.vi"("error in (no error)"=w2087, "timeout ms (wait forever: -1)"=1000, "port"=u16 2100, "service name"="RTLT") -> ("error out"=w2082:errorcluster, "connection ID"=w2083:refnum<k5>, "listener ID"=w2064:refnum<k5>)  [unwired: 3 in, 2 out]
        n888 = TCP Read(connection ID=w2083, bytes to read=512, error in (no error)=w2082, 7:T15."CRLF" ("mode (standard)"), 9:10000 ("timeout ms (25000)")) -> (connection ID out=w2072:refnum<k5>, data out=w2079:string, error out=w2073:errorcluster)
        n889 = Concatenate Strings("alive" ("string"), "\r\n") -> (w2076:string)
        n890 = Equal?(x=w2079, y=w2076) -> (x = y?=w2074:bool)
        n891 = case shown="True" w2074 {
          tunnel: w2073 -> [w2091 w2112]
          tunnel: w2072 -> [_ w2106]
          tunnel: [w2092 w2110] -> w2071
          tunnel: w2069 -> [w2098 _]
          tunnel: [w2094 0] -> w2068
          tunnel: [w2093 ""] -> w2066
          tunnel: [FALSE TRUE] -> w2065
          frame False {
            # "if unsuccessful and count <10, increament count \nand try again"
            n892 = Unbundle By Name(w2098) -> ("TCP attempt count"=w2095:i32)
            n893 = Less?(x=w2095, y=1) -> (x < y?=w2096:bool)
            n894 = case shown="True" w2096 {
              tunnel: w2095 -> [w2101 w2105]
              tunnel: [w2101 w2104] -> w2094
              tunnel: ["" "TCP: Initialize"] -> w2093
              tunnel: [errorcluster {"status"=TRUE, "code"=5001, "source"="TCP/IP"} ("error in (no error)") errorcluster {"status"=FALSE, "code"=5001, "source"=""} ("error in (no error)")] -> w2092
              tunnel: w2091 -> [_ _]
              frame False {
                # "send error and shut down"
              }
              frame True {
                # "try again until 10th"
                n895 = Increment(x=w2105) -> (x+1=w2104:i32)
              }
            }
          }
          frame True {
            # "if connection is successful\nwrite TCP FVG"
            n896 = call "TcpIDFGV.vi"("Error In"=w2112, "action"=enum16{"write", "read"}."write", "connection ID in"=w2106) -> ("Error Out"=w2110:errorcluster)  [unwired: 7 in, 1 out]
          }
        }
        n897 = Bundle By Name(cluster=w2069, "TCP attempt count"=w2068, "System Status.TCP/IP"=w2065, "listener ID"=w2064) -> (w2070:T16)
        n898 = global write "GlobalVariables.vi" "TCP connected?"(w2065) -> ()
        n899 = call <vilib>:"Add State(s) to Queue__JKI_lib_State_Machine.vi"("State(s) in Front (\"\")"=w2066, "State(s) in (\"\")"=w2089) -> ("States Out"=w2088:string)  [unwired: 13 in]
      }
      frame "TCP: SyncTime" {
        # "Template Separator\n(You can make a copy of, or modify, this frame)"
        n900 = call "TcpIDFGV.vi"("Error In"=w2117, "action"=enum16{"write", "read"}."read") -> ("Error Out"=w2116:errorcluster, "connection ID out"=w2114:refnum<k5>)  [unwired: 8 in]
        n901 = call <userlib>:"Tick Count (ms)__ogtk.vi"("error in (no error)"=w2116) -> ("error out"=w2115:errorcluster, "millisecond timer value"=w2113:u32)  [unwired: 9 in]
        n902 = while {
          tunnel: w2115 -> [w2141]
          tunnel: w2114 -> [w2140]
          tunnel: w2113 -> [w2129]
          stop <- w2124 stop-if-true
          n903 = Concatenate Strings("latencycheck" ("string"), "\r\n") -> (w2136:string)
          n904 = TCP Read(connection ID=w2140, bytes to read=512, error in (no error)=w2141, 7:T15."CRLF" ("mode (standard)"), 9:2000 ("timeout ms (25000)")) -> (connection ID out=w2133:refnum<k5>, data out=w2131:string, error out=w2123:errorcluster)
          n905 = Tick Count (ms)() -> (millisecond timer value=w2130:u32)
          n906 = Subtract(x=w2130, y=w2129) -> (x-y=w2128:u32)
          n907 = Equal?(x=w2131, y=w2136) -> (x = y?=w2132:bool)
          n908 = case shown="False" w2132 {
            tunnel: w2133 -> [_ w2154]
            tunnel: w2131 -> [w2146 _]
            tunnel: [w2142 FALSE] -> w2126
            tunnel: w2123 -> [_ w2148]
            frame False {
              n909 = Concatenate Strings("synctimer" ("string"), "\r\n") -> (w2143:string)
              n910 = Equal?(x=w2146, y=w2143) -> (x = y?=w2142:bool)
              "Sync Success?" <- w2142
            }
            frame True {
              n911 = Concatenate Strings("latencycheck:" ("string"), "\r\n") -> (w2153:string)
              n912 = TCP Write(connection ID=w2154, data in=w2153, error in (no error)=w2148, 9:1000 ("timeout ms (25000)")) -> (error out=w2147:errorcluster)  [unwired: 2 out]
              n913 = call <vilib>:"Clear Errors.vi"("error in (no error)"=w2147) -> ()  [unwired: 5 in, 2 out]
            }
          }
          n914 = Greater?(x=w2128, y=u32 10000 ("x-y")) -> (0:w2125:bool)
          n915 = Or(x=w2126, y=w2125) -> (x .or. y?=w2124:bool)
        }
        n916 = call <vilib>:"Add State(s) to Queue__JKI_lib_State_Machine.vi"("State(s) in (\"\")"=w2122) -> ("States Out"=w2121:string)  [unwired: 14 in]
      }
      frame "TCP: SendSettingMacro" {
        # "Template Separator\n(You can make a copy of, or modify, this frame)"
        n917 = Unbundle By Name(w2158) -> ("CaseID"=w2157:string, "System Status.TCP/IP"=w2156:bool)
        n918 = case shown="True" w2156 {
          tunnel: w2157 -> [_ _]
          tunnel: ["" "TCP: sendSubjectID\nTCP: sendScaleBarSetting\nTCP: sendScaleMaxMin\nTCP: sendDeconChannel\nTCP: sendANSI\nTCP: sendRadius\nTCP: send3Dsetting\nTCP: sendFirefly\nTCP: sendPenrero"] -> w2155
          frame False {
          }
          frame True {
          }
        }
        n919 = call <vilib>:"Add State(s) to Queue__JKI_lib_State_Machine.vi"("State(s) in Front (\"\")"=w2155, "State(s) in (\"\")"=w2162) -> ("States Out"=w2161:string)  [unwired: 13 in]
      }
      frame "TCP: sendRunNum" {
        # "Template Separator\n(You can make a copy of, or modify, this frame)"
        n920 = Unbundle By Name(w2168) -> ("IDs.RunID"=w2175:i8)
        n921 = Number To Decimal String(number=w2175, width (-)=i16 3) -> (decimal integer string=w2170:string)
        n922 = call "TcpIDFGV.vi"("Error In"=w2165, "action"=enum16{"write", "read"}."read") -> ("Error Out"=w2167:errorcluster, "connection ID out"=w2172:refnum<k5>)  [unwired: 8 in]
        n923 = Concatenate Strings("!run:", w2170) -> (w2169:string)
        n924 = call "TCP_WriteRead.vi"("error in (no error)"=w2167, "data in"=w2169, "connectin ID in"=w2172) -> ("error out"=w2166:errorcluster)  [unwired: 4 in, 2 out]
        n925 = call <vilib>:"Add State(s) to Queue__JKI_lib_State_Machine.vi"("State(s) in (\"\")"=w2178) -> ("States Out"=w2177:string)  [unwired: 14 in]
      }
      frame "TCP: sendVideoSource" {
        # "Send video source \n(You can make a copy of, or modify, this frame)"
        n926 = call "TcpIDFGV.vi"("Error In"=w2179, "action"=enum16{"write", "read"}."read") -> ("Error Out"=w2181:errorcluster, "connection ID out"=w2187:refnum<k5>)  [unwired: 8 in]
        n927 = case shown="\"FrameGrabber\"" "Video Source" {
          tunnel: [0 1] -> w2185
          frame "Camera", Default {
          }
          frame "FrameGrabber" {
          }
        }
        n928 = Number To Decimal String(number=w2185) -> (decimal integer string=w2183:string)  [unwired: 1 in]
        n929 = Concatenate Strings("!invivo:" ("data in"), w2183) -> (w2182:string)
        n930 = call "TCP_WriteRead.vi"("error in (no error)"=w2181, "data in"=w2182, "connectin ID in"=w2187) -> ("error out"=w2180:errorcluster)  [unwired: 4 in, 2 out]
        n931 = call <vilib>:"Add State(s) to Queue__JKI_lib_State_Machine.vi"("State(s) in (\"\")"=w2192) -> ("States Out"=w2191:string)  [unwired: 14 in]
      }
      frame "TCP: startRun" {
        # "Template Separator\n(You can make a copy of, or modify, this frame)"
        n932 = call "TcpIDFGV.vi"("Error In"=w2195, "action"=enum16{"write", "read"}."read") -> ("Error Out"=w2197:errorcluster, "connection ID out"=w2198:refnum<k5>)  [unwired: 8 in]
        n933 = call "TCP_WriteRead.vi"("error in (no error)"=w2197, "data in"="!acquire:1", "connectin ID in"=w2198) -> ("error out"=w2196:errorcluster)  [unwired: 4 in, 2 out]
        n934 = call <vilib>:"Add State(s) to Queue__JKI_lib_State_Machine.vi"("State(s) in (\"\")"=w2204) -> ("States Out"=w2203:string)  [unwired: 14 in]
      }
      frame "TCP: stopRun" {
        # "Template Separator\n(You can make a copy of, or modify, this frame)"
        n935 = call "TcpIDFGV.vi"("Error In"=w2205, "action"=enum16{"write", "read"}."read") -> ("Error Out"=w2207:errorcluster, "connection ID out"=w2209:refnum<k5>)  [unwired: 8 in]
        n936 = call "TCP_WriteRead.vi"("error in (no error)"=w2207, "data in"="!acquire:0", "connectin ID in"=w2209) -> ("error out"=w2206:errorcluster)  [unwired: 4 in, 2 out]
        n937 = call <vilib>:"Add State(s) to Queue__JKI_lib_State_Machine.vi"("State(s) in (\"\")"=w2214) -> ("States Out"=w2213:string)  [unwired: 14 in]
      }
      frame "TCP: SyncTimer" {
        # "Template Separator\n(You can make a copy of, or modify, this frame)"
        n938 = call "TcpIDFGV.vi"("Error In"=w2220, "action"=enum16{"write", "read"}."read") -> ("Error Out"=w2221:errorcluster, "connection ID out"=w2222:refnum<k5>)  [unwired: 8 in]
        n939 = while {
          tunnel: w2222 -> [w2241]
          shift-right: [w2236] -> w2216
          shift-left: w2221 -> [w2237]
          tunnel: [w2228] -> w2219
          i -> [w2233]
          stop <- w2231 stop-if-true
          n940 = TCP Read(connection ID=w2241, bytes to read=512, error in (no error)=w2237, 7:T15."CRLF" ("mode (standard)"), 9:1000 ("timeout ms (25000)")) -> (connection ID out=w2228:refnum<k5>, data out=w2235:string, error out=w2236:errorcluster)
          "syctimer data out" <- w2235
          n941 = Equal?(x="!synctimer:", y=w2235) -> (x = y?=w2230:bool)
          n942 = Greater?(x=w2233, y=10000) -> (0:w2229:bool)
          n943 = Or(x=w2230, y=w2229) -> (x .or. y?=w2231:bool)
        }
        n944 = TCP Write(connection ID=w2219, data in="!synctimer:", error in (no error)=w2216, 9:1000 ("timeout ms (25000)")) -> (error out=w2215:errorcluster)  [unwired: 2 out]
        n945 = call <vilib>:"Add State(s) to Queue__JKI_lib_State_Machine.vi"("State(s) in (\"\")"=w2227) -> ("States Out"=w2226:string)  [unwired: 14 in]
      }
      frame "TCP: CheckConnection" {
        # "Check TCP/IP connection statuse\n(If connection is lost, throw error)"
        n946 = Unbundle By Name(w2243) -> ("System Status.TCP/IP"=w2242:bool)
        n947 = case shown="True" w2242 {
          frame False {
          }
          frame True {
            # "If TCP/IP is true check, otherwise skip"
          }
        }
        n948 = call <vilib>:"Add State(s) to Queue__JKI_lib_State_Machine.vi"("State(s) in (\"\")"=w2247) -> ("States Out"=w2246:string)  [unwired: 14 in]
      }
      frame "TCP: Close" {
        # "Close TCP connection\n()"
        n949 = call "TcpIDFGV.vi"("Error In"=w2252, "action"=enum16{"write", "read"}."read") -> ("Error Out"=w2254:errorcluster, "connection ID out"=w2255:refnum<k5>)  [unwired: 8 in]
        n950 = TCP Close Connection(connection ID=w2255, error in (no error)=w2254) -> (error out=w2248:errorcluster)  [unwired: 1 in, 1 out]
        n951 = case shown="No Error" w2248 {
          tunnel: [w2260 w2261] -> w2250
          tunnel: w2249 -> [w2259 w2261]
          frame No Error {
            w2258 = FALSE ("System Status.TCP/IP")
            n952 = Bundle By Name(cluster=w2259, "System Status.TCP/IP"=w2258) -> (w2260:T16)
            n953 = global write "GlobalVariables.vi" "TCP connected?"(w2258) -> ()
          }
          frame Error {
          }
        }
        n954 = call <vilib>:"Add State(s) to Queue__JKI_lib_State_Machine.vi"("State(s) in (\"\")"=w2257) -> ("States Out"=w2256:string)  [unwired: 14 in]
      }
      frame "TCP: sendSubjectID" {
        # "Send subject ID"
        n955 = Unbundle By Name(w2269) -> ("CaseID"=w2268:string)
        n956 = Concatenate Strings("!subject:", w2268) -> (w2265:string)
        n957 = call "TcpIDFGV.vi"("Error In"=w2262, "action"=enum16{"write", "read"}."read") -> ("Error Out"=w2264:errorcluster, "connection ID out"=w2266:refnum<k5>)  [unwired: 8 in]
        n958 = call "TCP_WriteRead.vi"("error in (no error)"=w2264, "data in"=w2265, "connectin ID in"=w2266) -> ("error out"=w2263:errorcluster)  [unwired: 4 in, 2 out]
        n959 = call <vilib>:"Add State(s) to Queue__JKI_lib_State_Machine.vi"("State(s) in (\"\")"=w2273) -> ("States Out"=w2272:string)  [unwired: 14 in]
      }
      frame "TCP: sendScaleBarSetting" {
        # "Template Separator\n(You can make a copy of, or modify, this frame)"
        n960 = call "TcpIDFGV.vi"("Error In"=w2274, "action"=enum16{"write", "read"}."read") -> ("Error Out"=w2276:errorcluster, "connection ID out"=w2278:refnum<k5>)  [unwired: 8 in]
        n961 = call "TCP_WriteRead.vi"("error in (no error)"=w2276, "data in"="!autocolor:0", "connectin ID in"=w2278) -> ("error out"=w2275:errorcluster)  [unwired: 4 in, 2 out]
        n962 = call <vilib>:"Add State(s) to Queue__JKI_lib_State_Machine.vi"("State(s) in (\"\")"=w2283) -> ("States Out"=w2282:string)  [unwired: 14 in]
      }
      frame "TCP: sendScaleMaxMin" {
        # "Template Separator\n(You can make a copy of, or modify, this frame)"
        n963 = call "TcpIDFGV.vi"("Error In"=w2285, "action"=enum16{"write", "read"}."read") -> ("Error Out"=w2287:errorcluster, "connection ID out"=w2288:refnum<k5>)  [unwired: 8 in]
        n964 = call "TCP_WriteRead.vi"("error in (no error)"=w2287, "data in"="!color:3;6", "connectin ID in"=w2288) -> ("error out"=w2286:errorcluster)  [unwired: 4 in, 2 out]
        n965 = call <vilib>:"Add State(s) to Queue__JKI_lib_State_Machine.vi"("State(s) in (\"\")"=w2293) -> ("States Out"=w2292:string)  [unwired: 14 in]
      }
      frame "TCP: sendDeconChannel" {
        # "Send Decon channel\n(You can make a copy of, or modify, this frame)"
        n966 = local read "Radio Buttons"() -> (w2296:enum32{"No Selection", "Ch1", "Ch2", "Ch3"})
        n967 = Increment(x=w2296) -> (x+1=w2295:enum32{"No Selection", "Ch1", "Ch2", "Ch3"})
        n968 = Number To Decimal String(number=w2295) -> (decimal integer string=w2294:string)  [unwired: 1 in]
        n969 = call "TcpIDFGV.vi"("Error In"=w2297, "action"=enum16{"write", "read"}."read") -> ("Error Out"=w2299:errorcluster, "connection ID out"=w2302:refnum<k5>)  [unwired: 8 in]
        n970 = Concatenate Strings("!channel:", w2294) -> (w2300:string)
        n971 = call "TCP_WriteRead.vi"("error in (no error)"=w2299, "data in"=w2300, "connectin ID in"=w2302) -> ("error out"=w2298:errorcluster)  [unwired: 4 in, 2 out]
        n972 = call <vilib>:"Add State(s) to Queue__JKI_lib_State_Machine.vi"("State(s) in (\"\")"=w2307) -> ("States Out"=w2306:string)  [unwired: 14 in]
      }
      frame "TCP: sendANSI" {
        # "Template Separator\n(You can make a copy of, or modify, this frame)"
        n973 = call "TcpIDFGV.vi"("Error In"=w2308, "action"=enum16{"write", "read"}."read") -> ("Error Out"=w2311:errorcluster, "connection ID out"=w2312:refnum<k5>)  [unwired: 8 in]
        n974 = call "TCP_WriteRead.vi"("error in (no error)"=w2311, "data in"="!ansi:20", "connectin ID in"=w2312) -> ("error out"=w2309:errorcluster)  [unwired: 4 in, 2 out]
        n975 = call <vilib>:"Add State(s) to Queue__JKI_lib_State_Machine.vi"("State(s) in (\"\")"=w2317) -> ("States Out"=w2316:string)  [unwired: 14 in]
      }
      frame "TCP: sendRadius" {
        # "Template Separator\n(You can make a copy of, or modify, this frame)"
        n976 = call "TcpIDFGV.vi"("Error In"=w2319, "action"=enum16{"write", "read"}."read") -> ("Error Out"=w2321:errorcluster, "connection ID out"=w2322:refnum<k5>)  [unwired: 8 in]
        n977 = call "TCP_WriteRead.vi"("error in (no error)"=w2321, "data in"="!radius:1.0", "connectin ID in"=w2322) -> ("error out"=w2320:errorcluster)  [unwired: 4 in, 2 out]
        n978 = call <vilib>:"Add State(s) to Queue__JKI_lib_State_Machine.vi"("State(s) in (\"\")"=w2327) -> ("States Out"=w2326:string)  [unwired: 14 in]
      }
      frame "TCP: send3Dsetting" {
        # "Template Separator\n(You can make a copy of, or modify, this frame)"
        n979 = call "TcpIDFGV.vi"("Error In"=w2328, "action"=enum16{"write", "read"}."read") -> ("Error Out"=w2330:errorcluster, "connection ID out"=w2332:refnum<k5>)  [unwired: 8 in]
        n980 = call "TCP_WriteRead.vi"("error in (no error)"=w2330, "data in"="!3dset:0", "connectin ID in"=w2332) -> ("error out"=w2329:errorcluster)  [unwired: 4 in, 2 out]
        n981 = call <vilib>:"Add State(s) to Queue__JKI_lib_State_Machine.vi"("State(s) in (\"\")"=w2337) -> ("States Out"=w2336:string)  [unwired: 14 in]
      }
      frame "TCP: sendFirefly" {
        # "Template Separator\n(You can make a copy of, or modify, this frame)"
        n982 = call "TcpIDFGV.vi"("Error In"=w2338, "action"=enum16{"write", "read"}."read") -> ("Error Out"=w2340:errorcluster, "connection ID out"=w2342:refnum<k5>)  [unwired: 8 in]
        n983 = call "TCP_WriteRead.vi"("error in (no error)"=w2340, "data in"="!firefly:1", "connectin ID in"=w2342) -> ("error out"=w2339:errorcluster)  [unwired: 4 in, 2 out]
        n984 = call <vilib>:"Add State(s) to Queue__JKI_lib_State_Machine.vi"("State(s) in (\"\")"=w2347) -> ("States Out"=w2346:string)  [unwired: 14 in]
      }
      frame "TCP: sendPenrero" {
        # "Template Separator\n(You can make a copy of, or modify, this frame)"
        n985 = call "TcpIDFGV.vi"("Error In"=w2348, "action"=enum16{"write", "read"}."read") -> ("Error Out"=w2350:errorcluster, "connection ID out"=w2352:refnum<k5>)  [unwired: 8 in]
        n986 = call "TCP_WriteRead.vi"("error in (no error)"=w2350, "data in"="!pentero:0", "connectin ID in"=w2352) -> ("error out"=w2349:errorcluster)  [unwired: 4 in, 2 out]
        n987 = call <vilib>:"Add State(s) to Queue__JKI_lib_State_Machine.vi"("State(s) in (\"\")"=w2357) -> ("States Out"=w2356:string)  [unwired: 14 in]
      }
      frame "---------- UI ----------" {
        # "Do not put any code in this frame.\n(It is a separator no-op. You can make a copy of this frame to create a new UI frame)"
        n988 = call <vilib>:"Add State(s) to Queue__JKI_lib_State_Machine.vi"("State(s) in (\"\")"=w2362) -> ("States Out"=w2361:string)  [unwired: 14 in]
      }
      frame "UI: BGLoaded" {
        # "Do not put any code in this frame.\n(It is a separator no-op. You can make a copy of this frame to create a new UI frame)"
        n989 = property on="Background" class="Bool (strict)"("BoolText.Text"="Loaded!" ("Boolean Text.Text"), "Colors [4]"=cluster{u32, u32}[] [{15764023, 15764023}, {16711680, 16711680}]) -> ()  [unwired: 2 in, 2 out]
        n990 = call <vilib>:"Add State(s) to Queue__JKI_lib_State_Machine.vi"("State(s) in (\"\")"=w2369) -> ("States Out"=w2368:string)  [unwired: 14 in]
      }
      frame "UI: CaliAndiRFLoaded" {
        # "Do not put any code in this frame.\n(It is a separator no-op. You can make a copy of this frame to create a new UI frame)"
        n991 = property on="Cali&iRF alignment" class="Bool (strict)"("BoolText.Text"="Loaded!" ("Boolean Text.Text"), "Colors [4]"=cluster{u32, u32}[] [{15764023, 15764023}, {16711680, 16711680}]) -> ()  [unwired: 2 in, 2 out]
        n992 = call <vilib>:"Add State(s) to Queue__JKI_lib_State_Machine.vi"("State(s) in (\"\")"=w2376) -> ("States Out"=w2375:string)  [unwired: 14 in]
      }
      frame "UI: WFAutoScale" {
        # "Set graph auto scale.\n(UI: WFAutoScale >> T/F)"
        n993 = Equal?(x=w2377, y="F") -> (x = y?=w2378:bool)
        n994 = Equal?(x=w2377, y="T") -> (x = y?=w2380:bool)
        n995 = case shown="True" w2378 {
          frame False {
          }
          frame True {
            w2393 = 0.0 ("Y Scale.Range:Maximum")
            w2394 = 2.0 ("Y Scale.Range:Maximum")
            w2395 = u8 0 ("Y Scale.Scale Fit")
            n996 = property on="Channel 1" class="WFGraph (strict)"("YScale.ScaleFit"=w2395) -> (error out=w2392:errorcluster)  [unwired: 2 in, 1 out]
            n997 = property on="Channel 2" class="WFGraph (strict)"("YScale.ScaleFit"=w2395) -> (error out=w2391:errorcluster)  [unwired: 2 in, 1 out]
            n998 = property on="Channel 3" class="WFGraph (strict)"("YScale.ScaleFit"=w2395) -> (error out=w2390:errorcluster)  [unwired: 2 in, 1 out]
            n999 = property on="Channel 1" class="WFGraph (strict)"(error in=w2392, "YScale.Maximum"=w2394) -> (error out=w2389:errorcluster)  [unwired: 1 in, 1 out]
            n1000 = property on="Channel 2" class="WFGraph (strict)"(error in=w2391, "YScale.Maximum"=w2394) -> (error out=w2388:errorcluster)  [unwired: 1 in, 1 out]
            n1001 = property on="Channel 3" class="WFGraph (strict)"(error in=w2390, "YScale.Maximum"=w2394) -> (error out=w2387:errorcluster)  [unwired: 1 in, 1 out]
            n1002 = property on="Channel 1" class="WFGraph (strict)"(error in=w2389, "YScale.Minimum"=w2393) -> ()  [unwired: 1 in, 2 out]
            n1003 = property on="Channel 2" class="WFGraph (strict)"(error in=w2388, "YScale.Minimum"=w2393) -> ()  [unwired: 1 in, 2 out]
            n1004 = property on="Channel 3" class="WFGraph (strict)"(error in=w2387, "YScale.Minimum"=w2393) -> ()  [unwired: 1 in, 2 out]
          }
        }
        n1005 = case shown="True" w2380 {
          frame False {
          }
          frame True {
            w2396 = u8 2 ("Y Scale.Scale Fit")
            n1006 = property on="Channel 1" class="WFGraph (strict)"("YScale.ScaleFit"=w2396) -> ()  [unwired: 2 in, 2 out]
            n1007 = property on="Channel 2" class="WFGraph (strict)"("YScale.ScaleFit"=w2396) -> ()  [unwired: 2 in, 2 out]
            n1008 = property on="Channel 3" class="WFGraph (strict)"("YScale.ScaleFit"=w2396) -> ()  [unwired: 2 in, 2 out]
          }
        }
        n1009 = call <vilib>:"Add State(s) to Queue__JKI_lib_State_Machine.vi"("State(s) in (\"\")"=w2386) -> ("States Out"=w2385:string)  [unwired: 14 in]
      }
      frame "UI: Initialize" {
        w2397 = T29 {"Minimum"=0.0, "Maximum"=4.6, "Increment"=0.1} ("Data Entry Limits")
        w2399 = T10."Disabled and Grayed Out" ("Disabled")
        # "Disable all button on startup"
        # "Initialize the User Interface, here.\n(this is called automatically, by the Macro: Init)"
        n1010 = property on="Gain 1" class="DigNum (strict)"("DisabledEnum"=w2399) -> ()  [unwired: 2 in, 2 out]
        n1011 = property on="Gain 2" class="DigNum (strict)"("DisabledEnum"=w2399) -> ()  [unwired: 2 in, 2 out]
        n1012 = property on="StopButton" class="Bool (strict)"("DisabledEnum"=w2399) -> ()  [unwired: 2 in, 2 out]
        n1013 = property on="Sys Reconfig" class="Bool"("DisabledEnum"=w2399) -> ()  [unwired: 2 in, 2 out]
        n1014 = property on="StartButton" class="Bool (strict)"("DisabledEnum"=w2399) -> ()  [unwired: 2 in, 2 out]
        n1015 = property on="355nm Laser toggle" class="Bool (strict)"("DisabledEnum"=w2399) -> ()  [unwired: 2 in, 2 out]
        n1016 = property on="Aiming beam toggle" class="Bool (strict)"("DisabledEnum"=w2399) -> ()  [unwired: 2 in, 2 out]
        n1017 = property on="Background" class="Bool (strict)"("DisabledEnum"=w2399) -> ()  [unwired: 2 in, 2 out]
        n1018 = property on="Cali&iRF alignment" class="Bool (strict)"("DisabledEnum"=w2399) -> ()  [unwired: 2 in, 2 out]
        n1019 = property on="Gain 3" class="DigNum (strict)"("DisabledEnum"=w2399) -> ()  [unwired: 2 in, 2 out]
        n1020 = property on="Gain 1" class="DigNum (strict)"("Data Range"=w2397) -> ()  [unwired: 2 in, 2 out]
        n1021 = property on="Gain 2" class="DigNum (strict)"("Data Range"=w2397) -> ()  [unwired: 2 in, 2 out]
        n1022 = property on="Gain 3" class="DigNum (strict)"("Data Range"=w2397) -> ()  [unwired: 2 in, 2 out]
        n1023 = call <vilib>:"Add State(s) to Queue__JKI_lib_State_Machine.vi"("State(s) in Front (\"\")"="UI: CaliAndiRFNotReady" ("State(s) in Front (\"\")"), "State(s) in (\"\")"=w2404) -> ("States Out"=w2403:string)  [unwired: 13 in]
      }
      frame "UI: showDisclaimer" {
        # "Show disclamer window.\n(It is a separator no-op. You can make a copy of this frame to create a new UI frame)"
        n1024 = call <vilib>:"Application Directory.vi"() -> ("Application Directory"=w2417:path)
        n1025 = Build Path(base path=w2417, name or relative path="Disclamer.png") -> (appended path=w2415:path)
        n1026 = disable-structure shown="Disabled" {
          frame Disabled {
            n1027 = flat-sequence {
              frame #0 {
                n1028 = call "disclaimer.vi"() -> ()  [unwired: 12 in]
              }
              frame #1 {
                n1029 = Wait (ms)(milliseconds to wait=u32 250) -> ()  [unwired: 1 out]
              }
              frame #2 {
                n1030 = call "SoftwareNote.vi"() -> ()  [unwired: 12 in]
              }
            }
          }
          frame Enabled {
          }
        }
        n1031 = property on="Disclamer" class="Pict"() -> ("Draw Area Size"=w2413:T30)  [unwired: 2 in, 2 out]
        n1032 = call <vilib>:"Read PNG File.vi"("path to PNG file"=w2415) -> ("image data"=w2412:T31)  [unwired: 8 in, 2 out]
        n1033 = Unbundle By Name(w2412) -> ("Rectangle.right"=w2410:i16, "Rectangle.bottom"=w2408:i16)
        n1034 = Unbundle By Name(w2413) -> ("Width"=w2411:u32, "Height"=w2409:u32)
        n1035 = call <vilib>:"Draw Flattened Pixmap.vi"("image data"=w2412) -> ("new picture"=→"Disclamer":picture)  [unwired: 8 in]
        n1036 = Divide(x=w2411, y=w2410) -> (x/y=w2407:dbl)
        n1037 = Divide(x=w2409, y=w2408) -> (x/y=w2406:dbl)
        n1038 = Max & Min(x=w2407, y=w2406) -> (min(x,y)=w2405:dbl)  [unwired: 1 out]
        n1039 = property on="Disclamer" class="Pict"("ZoomFactor"=w2405) -> ()  [unwired: 2 in, 2 out]
        n1040 = call <vilib>:"Add State(s) to Queue__JKI_lib_State_Machine.vi"("State(s) in (\"\")"=w2422) -> ("States Out"=w2421:string)  [unwired: 14 in]
      }
      frame "UI: CaliAndiRFNotReady" {
        # "Do not put any code in this frame.\n(It is a separator no-op. You can make a copy of this frame to create a new UI frame)"
        n1041 = property on="Cali&iRF alignment" class="Bool (strict)"("BoolText.Text"="No Info" ("Boolean Text.Text"), "Colors [4]"=cluster{u32, u32}[] [{13816530, 13816530}, {16711680, 16711680}]) -> ()  [unwired: 2 in, 2 out]
        n1042 = call <vilib>:"Add State(s) to Queue__JKI_lib_State_Machine.vi"("State(s) in (\"\")"=w2430) -> ("States Out"=w2429:string)  [unwired: 14 in]
      }
      frame "UI: BGnotReady" {
        # "Do not put any code in this frame.\n(It is a separator no-op. You can make a copy of this frame to create a new UI frame)"
        n1043 = property on="Background" class="Bool (strict)"("BoolText.Text"="No Info" ("Boolean Text.Text"), "Colors [4]"=cluster{u32, u32}[] [{13816530, 13816530}, {16711680, 16711680}]) -> ()  [unwired: 2 in, 2 out]
        n1044 = call <vilib>:"Add State(s) to Queue__JKI_lib_State_Machine.vi"("State(s) in (\"\")"=w2437) -> ("States Out"=w2436:string)  [unwired: 14 in]
      }
      frame "UI: Reset" {
        w2439 = cluster{u32, u32}[] [{13816530, 13816530}, {13816530, 13816530}] ("Colors [4]")
        # "Do not put any code in this frame.\n(It is a separator no-op. You can make a copy of this frame to create a new UI frame)"
        n1045 = property on="Cali&iRF alignment" class="Bool (strict)"("BoolText.Text"="No Info" ("Boolean Text.Text"), "Colors [4]"=w2439) -> ()  [unwired: 2 in, 2 out]
        n1046 = property on="Background" class="Bool (strict)"("BoolText.Text"="No Info" ("Boolean Text.Text"), "Colors [4]"=w2439) -> ()  [unwired: 2 in, 2 out]
        n1047 = call <vilib>:"Add State(s) to Queue__JKI_lib_State_Machine.vi"("State(s) in (\"\")"=w2445) -> ("States Out"=w2444:string)  [unwired: 14 in]
      }
      frame "UI: SetButtonText" {
        # "Set button text of 355nm laser and aiming beam."
        n1048 = call <vilib>:"Add State(s) to Queue__JKI_lib_State_Machine.vi"("State(s) in (\"\")"=w2450) -> ("States Out"=w2449:string)  [unwired: 14 in]
      }
      frame "UI: DuringAquisition" {
        w2451 = T10."Disabled and Grayed Out" ("Disabled")
        # "Do not put any code in this frame.\n(It is a separator no-op. You can make a copy of this frame to create a new UI frame)"
        n1049 = property on="StopButton" class="Bool (strict)"("DisabledEnum"=T10."Enabled" ("Disabled")) -> ()  [unwired: 2 in, 2 out]
        n1050 = property on="StartButton" class="Bool (strict)"("DisabledEnum"=w2451) -> ()  [unwired: 2 in, 2 out]
        n1051 = property on="Sys Reconfig" class="Bool"("DisabledEnum"=w2451) -> ()  [unwired: 2 in, 2 out]
        n1052 = property on="355nm Laser toggle" class="Bool (strict)"("DisabledEnum"=w2451) -> ()  [unwired: 2 in, 2 out]
        n1053 = property on="Aiming beam toggle" class="Bool (strict)"("DisabledEnum"=w2451) -> ()  [unwired: 2 in, 2 out]
        n1054 = property on="Background" class="Bool (strict)"("DisabledEnum"=w2451) -> ()  [unwired: 2 in, 2 out]
        n1055 = property on="Cali&iRF alignment" class="Bool (strict)"("DisabledEnum"=w2451) -> ()  [unwired: 2 in, 2 out]
        n1056 = property on="Radio Buttons" class="RadioBtnsControl (strict)"("DisabledEnum"=w2451) -> ()  [unwired: 2 in, 2 out]
        n1057 = property on="Video Source" class="RadioBtnsControl (strict)"("DisabledEnum"=w2451) -> ()  [unwired: 2 in, 2 out]
        n1058 = property on="Quit" class="Bool"("DisabledEnum"=w2451) -> ()  [unwired: 2 in, 2 out]
        n1059 = call <vilib>:"Add State(s) to Queue__JKI_lib_State_Machine.vi"("State(s) in (\"\")"=w2457) -> ("States Out"=w2456:string)  [unwired: 14 in]
      }
      frame "UI: duringIRFAlign" {
        w2458 = T10."Disabled and Grayed Out" ("Disabled")
        # "Set UI to during iRF alignment\n(It is a separator no-op. You can make a copy of this frame to create a new UI frame)"
        n1060 = property on="StartButton" class="Bool (strict)"("DisabledEnum"=w2458) -> ()  [unwired: 2 in, 2 out]
        n1061 = property on="Sys Reconfig" class="Bool"("DisabledEnum"=w2458) -> ()  [unwired: 2 in, 2 out]
        n1062 = property on="355nm Laser toggle" class="Bool (strict)"("DisabledEnum"=w2458) -> ()  [unwired: 2 in, 2 out]
        n1063 = property on="Aiming beam toggle" class="Bool (strict)"("DisabledEnum"=w2458) -> ()  [unwired: 2 in, 2 out]
        n1064 = property on="Background" class="Bool (strict)"("DisabledEnum"=w2458) -> ()  [unwired: 2 in, 2 out]
        n1065 = property on="StopButton" class="Bool (strict)"("DisabledEnum"=w2458) -> ()  [unwired: 2 in, 2 out]
        n1066 = call <vilib>:"Add State(s) to Queue__JKI_lib_State_Machine.vi"("State(s) in (\"\")"=w2463) -> ("States Out"=w2462:string)  [unwired: 14 in]
      }
      frame "UI: duringBGAcquire" {
        w2464 = T10."Disabled and Grayed Out" ("Disabled")
        # "Do not put any code in this frame.\n(It is a separator no-op. You can make a copy of this frame to create a new UI frame)"
        n1067 = property on="StartButton" class="Bool (strict)"("DisabledEnum"=w2464) -> ()  [unwired: 2 in, 2 out]
        n1068 = property on="StopButton" class="Bool (strict)"("DisabledEnum"=w2464) -> ()  [unwired: 2 in, 2 out]
        n1069 = property on="Sys Reconfig" class="Bool"("DisabledEnum"=w2464) -> ()  [unwired: 2 in, 2 out]
        n1070 = property on="355nm Laser toggle" class="Bool (strict)"("DisabledEnum"=w2464) -> ()  [unwired: 2 in, 2 out]
        n1071 = property on="Aiming beam toggle" class="Bool (strict)"("DisabledEnum"=w2464) -> ()  [unwired: 2 in, 2 out]
        n1072 = property on="Cali&iRF alignment" class="Bool (strict)"("DisabledEnum"=w2464) -> ()  [unwired: 2 in, 2 out]
        n1073 = call <vilib>:"Add State(s) to Queue__JKI_lib_State_Machine.vi"("State(s) in (\"\")"=w2469) -> ("States Out"=w2468:string)  [unwired: 14 in]
      }
      frame "UI: ReadyForAquisition" {
        w2470 = T10."Enabled" ("Disabled")
        # "Do not put any code in this frame.\n(It is a separator no-op. You can make a copy of this frame to create a new UI frame)"
        n1074 = property on="StopButton" class="Bool (strict)"("DisabledEnum"=T10."Disabled and Grayed Out" ("Disabled")) -> ()  [unwired: 2 in, 2 out]
        n1075 = property on="StartButton" class="Bool (strict)"("DisabledEnum"=w2470) -> ()  [unwired: 2 in, 2 out]
        n1076 = property on="Sys Reconfig" class="Bool"("DisabledEnum"=w2470) -> ()  [unwired: 2 in, 2 out]
        n1077 = property on="355nm Laser toggle" class="Bool (strict)"("DisabledEnum"=w2470) -> ()  [unwired: 2 in, 2 out]
        n1078 = property on="Aiming beam toggle" class="Bool (strict)"("DisabledEnum"=w2470) -> ()  [unwired: 2 in, 2 out]
        n1079 = property on="Cali&iRF alignment" class="Bool (strict)"("DisabledEnum"=w2470) -> ()  [unwired: 2 in, 2 out]
        n1080 = property on="Video Source" class="RadioBtnsControl (strict)"("DisabledEnum"=w2470) -> ()  [unwired: 2 in, 2 out]
        n1081 = property on="Background" class="Bool (strict)"("DisabledEnum"=w2470) -> ()  [unwired: 2 in, 2 out]
        n1082 = property on="Quit" class="Bool"("DisabledEnum"=w2470) -> ()  [unwired: 2 in, 2 out]
        n1083 = property on="Radio Buttons" class="RadioBtnsControl (strict)"("DisabledEnum"=w2470) -> ()  [unwired: 2 in, 2 out]
        n1084 = call <vilib>:"Add State(s) to Queue__JKI_lib_State_Machine.vi"("State(s) in Front (\"\")"="LED: Green" ("State(s) in Front (\"\")"), "State(s) in (\"\")"=w2477) -> ("States Out"=w2476:string)  [unwired: 13 in]
      }
      frame "UI: Update" {
        # "Do not put any code in this frame.\n(It is a separator no-op. You can make a copy of this frame to create a new UI frame)"
        n1085 = Unbundle By Name(w2487) -> ("System Status"=→"System Hardware Connection Status":T1, "IDs.RunID"=→"Run #":i8, "CaseID"=→"Case #":string, "FLImDAQ"=→"FLImDAQ":T22, "SysRunning?"=→"Aquisition Status:":bool, "LJ Pinout"=→"LJ Pinout":T4, "IDs.BG ID"=→"BG #":i8, "IDs.Cali ID"=→"Calibration #":i8)
        n1086 = call <vilib>:"Add State(s) to Queue__JKI_lib_State_Machine.vi"("State(s) in (\"\")"=w2490) -> ("States Out"=w2489:string)  [unwired: 14 in]
      }
      frame "UI: Cursor Set" {
        # "Argument"
        # "Set and Unset Cursor Busy.\n(Usage: \"UI: Cursor Set >> Busy|Idle\")"
        n1087 = case shown="\"Idle\", Default" w2492 {
          tunnel: w2494 -> [w2499 w2501]
          tunnel: [w2498 w2500] -> w2493
          frame "Idle", Default {
            n1088 = call <vilib>:"Unset Busy.vi"("error in (no error)"=w2499) -> ("error out"=w2498:errorcluster)  [unwired: 10 in]
          }
          frame "Busy" {
            n1089 = call <vilib>:"Set Busy.vi"("error in (no error)"=w2501) -> ("error out"=w2500:errorcluster)  [unwired: 9 in, 1 out]
          }
        }
        n1090 = call <vilib>:"Add State(s) to Queue__JKI_lib_State_Machine.vi"("State(s) in (\"\")"=w2497) -> ("States Out"=w2496:string)  [unwired: 14 in]
      }
      frame "UI: Front Panel State" {
        # "Argument"
        # "Set Front Panel Open or Closed\n(Usage: \"UI: Front Panel State >> Open|Close\")"
        n1091 = Unbundle By Name(w2505) -> ("Core.Current VI Reference"=w2504:refnum<vi>)
        n1092 = case shown="\"Open\", \"Standard\", Default" w2503 {
          tunnel: w2507 -> [w2515 w2530 w2541 w2554 w2567]
          tunnel: [w2517 w2531 w2543 w2556 w2569] -> w2506
          tunnel: w2504 -> [w2516 w2528 w2542 w2555 w2568]
          frame "Open", "Standard", Default {
            w2510 = T12."Standard" ("State")
            n1093 = property class="VI"(reference=w2516, error in=w2515) -> (reference out=w2513:refnum<vi>, error out=w2514:errorcluster, "FP.State"=w2512:T12)
            n1094 = Not Equal?(x=w2512, y=w2510) -> (x != y?=w2511:bool)
            n1095 = case shown="True" w2511 {
              tunnel: [w2521 w2523] -> w2517
              tunnel: w2514 -> [w2520 w2523]
              tunnel: w2513 -> [w2519 _]
              tunnel: w2510 -> [w2518 _]
              frame True {
                n1096 = invoke class="VI" method="FP.Open"(reference=w2519, error in=w2520, "Activate"=TRUE, "State"=w2518) -> (error out=w2521:errorcluster)  [unwired: 1 in, 4 out]
              }
              frame False {
              }
            }
          }
          frame "Close", "Closed" {
            n1097 = property class="VI"(reference=w2528, error in=w2530) -> (reference out=w2527:refnum<vi>, error out=w2529:errorcluster, "FP.State"=w2525:T12)
            n1098 = Not Equal?(x=w2525, y=T12."Closed" ("Front Panel Window:State")) -> (x != y?=w2524:bool)
            n1099 = case shown="True" w2524 {
              tunnel: [w2532 w2535] -> w2531
              tunnel: w2529 -> [w2532 w2534]
              tunnel: w2527 -> [_ w2533]
              frame False {
              }
              frame True {
                n1100 = invoke class="VI" method="FP.Close"(reference=w2533, error in=w2534) -> (error out=w2535:errorcluster)  [unwired: 1 in, 2 out]
              }
            }
          }
          frame "Hidden", "Hide" {
            w2536 = T12."Hidden" ("State")
            n1101 = property class="VI"(reference=w2542, error in=w2541) -> (reference out=w2539:refnum<vi>, error out=w2540:errorcluster, "FP.State"=w2538:T12)
            n1102 = Not Equal?(x=w2538, y=w2536) -> (x != y?=w2537:bool)
            n1103 = case shown="True" w2537 {
              tunnel: [w2547 w2548] -> w2543
              tunnel: w2540 -> [w2546 w2548]
              tunnel: w2539 -> [w2545 _]
              tunnel: w2536 -> [w2544 _]
              frame True {
                n1104 = invoke class="VI" method="FP.Open"(reference=w2545, error in=w2546, "State"=w2544) -> (error out=w2547:errorcluster)  [unwired: 2 in, 4 out]
              }
              frame False {
              }
            }
          }
          frame "Minimize", "Minimized" {
            w2549 = T12."Minimized" ("State")
            n1105 = property class="VI"(reference=w2555, error in=w2554) -> (reference out=w2552:refnum<vi>, error out=w2553:errorcluster, "FP.State"=w2551:T12)
            n1106 = Not Equal?(x=w2551, y=w2549) -> (x != y?=w2550:bool)
            n1107 = case shown="True" w2550 {
              tunnel: [w2560 w2561] -> w2556
              tunnel: w2553 -> [w2559 w2561]
              tunnel: w2552 -> [w2558 _]
              tunnel: w2549 -> [w2557 _]
              frame True {
                n1108 = invoke class="VI" method="FP.Open"(reference=w2558, error in=w2559, "State"=w2557) -> (error out=w2560:errorcluster)  [unwired: 2 in, 4 out]
              }
              frame False {
              }
            }
          }
          frame "Maximize", "Maximized" {
            w2562 = T12."Maximized" ("State")
            n1109 = property class="VI"(reference=w2568, error in=w2567) -> (reference out=w2565:refnum<vi>, error out=w2566:errorcluster, "FP.State"=w2564:T12)
            n1110 = Not Equal?(x=w2564, y=w2562) -> (x != y?=w2563:bool)
            n1111 = case shown="True" w2563 {
              tunnel: [w2573 w2574] -> w2569
              tunnel: w2566 -> [w2572 w2574]
              tunnel: w2565 -> [w2571 _]
              tunnel: w2562 -> [w2570 _]
              frame True {
                n1112 = invoke class="VI" method="FP.Open"(reference=w2571, error in=w2572, "State"=w2570) -> (error out=w2573:errorcluster)  [unwired: 2 in, 4 out]
              }
              frame False {
              }
            }
          }
        }
        n1113 = call <vilib>:"Add State(s) to Queue__JKI_lib_State_Machine.vi"("State(s) in (\"\")"=w2509) -> ("States Out"=w2508:string)  [unwired: 14 in]
      }
      frame "---------- 355 Laser ----------" {
        # "Template Separator\n(You can make a copy of, or modify, this frame)"
        n1114 = call <vilib>:"Add State(s) to Queue__JKI_lib_State_Machine.vi"("State(s) in (\"\")"=w2579) -> ("States Out"=w2578:string)  [unwired: 14 in]
      }
      frame "355 Laser: Check Dewelling" {
        # "if time laser start time is less than 7.5s before, wait 250ms then check again."
        # "Template Separator\n(You can make a copy of, or modify, this frame)"
        n1115 = Unbundle By Name(w2587) -> ("Laser start tic"=w2584:u32)
        n1116 = Tick Count (ms)() -> (millisecond timer value=w2585:u32)
        n1117 = Subtract(x=w2585, y=w2584) -> (x-y=w2583:u32)
        n1118 = Greater?(x=w2583, y=u32 5000) -> (0:w2581:bool)
        n1119 = case shown="False" w2581 {
          tunnel: ["355 Laser: Check Dewelling" ""] -> w2580
          frame False {
            n1120 = Wait (ms)(milliseconds to wait=u32 250) -> ()  [unwired: 1 out]
          }
          frame True {
          }
        }
        n1121 = call <vilib>:"Add State(s) to Queue__JKI_lib_State_Machine.vi"("State(s) in Front (\"\")"=w2580, "State(s) in (\"\")"=w2590) -> ("States Out"=w2589:string)  [unwired: 13 in]
      }
      frame "355 Laser: Laser enable/disable" {
        # "Laser enable/disable\n(Usage: \"LabJack: Laser enable/disable >> 1|0\")"
        n1122 = Unbundle By Name(w2595) -> ("LJ Pinout.Laser Start/Stop"=w2603:string)
        n1123 = call "LabJack_FGV.vi"("Operation(Read)"=enum16{"Write", "Read"}."Read" ("Operation")) -> ("Read data"=w2605:i32)  [unwired: 9 in, 1 out]
        n1124 = call <vilib>:"LJM_eWriteName.vi"("Handle In"=w2605, "Name"=w2603, "Value"=1.0, "error in"=w2609) -> ("Handle Out"=w2604:i32, "error out"=w2602:errorcluster)  [unwired: 10 in]
        n1125 = call <userlib>:"Wait (ms)__ogtk.vi"("error in (no error)"=w2602, "milliseconds to wait"=u32 250) -> ("error out"=w2601:errorcluster)  [unwired: 8 in, 1 out]
        n1126 = call <vilib>:"LJM_eWriteName.vi"("Handle In"=w2604, "Name"=w2603, "Value"=0.0, "error in"=w2601) -> ("error out"=w2598:errorcluster)  [unwired: 10 in, 1 out]
        n1127 = call <userlib>:"Tick Count (ms)__ogtk.vi"("error in (no error)"=w2598) -> ("error out"=w2597:errorcluster, "millisecond timer value"=w2594:u32)  [unwired: 9 in]
        n1128 = Bundle By Name(cluster=w2595, "Laser start tic"=w2594) -> (w2596:T16)
        n1129 = call <vilib>:"Add State(s) to Queue__JKI_lib_State_Machine.vi"("State(s) in (\"\")"=w2611) -> ("States Out"=w2610:string)  [unwired: 14 in]
      }
      frame "355 Laser: Dewelling" {
        # "Wait some time (ms)\n(355 Laser: Dewelling >> #)"
        n1130 = Fract/Exp String To Number(string=w2615, default (0 dbl)=0) -> (number=w2613:i32)  [unwired: 2 in, 1 out]
        n1131 = Wait (ms)(milliseconds to wait=w2613) -> ()  [unwired: 1 out]
        n1132 = call <vilib>:"Add State(s) to Queue__JKI_lib_State_Machine.vi"("State(s) in (\"\")"=w2619) -> ("States Out"=w2618:string)  [unwired: 14 in]
      }
      frame "355 Laser: Init" {
        # "Initilize 355nm laser\n(Start laser, enable interlock)"
        n1133 = call <vilib>:"Add State(s) to Queue__JKI_lib_State_Machine.vi"("State(s) in Front (\"\")"="355 Laser: CheckControllerStatus", "State(s) in (\"\")"=w2625) -> ("States Out"=w2624:string)  [unwired: 13 in]
      }
      frame "355 Laser: Close" {
        # "Template Separator\n(You can make a copy of, or modify, this frame)"
        n1134 = call <vilib>:"Add State(s) to Queue__JKI_lib_State_Machine.vi"("State(s) in Front (\"\")"="355 Laser: Laser enable/disable\n355 Laser: Dewelling >>1000", "State(s) in (\"\")"=w2631) -> ("States Out"=w2630:string)  [unwired: 13 in]
      }
      frame "355 Laser: CheckControllerStatus" {
        # "if average < 1, laser on\nif average > 9, laser off\nif 1<average<9, interlock open, blink indicator"
        # "take 10 measuremt and look at average"
        # "Check 355 laser controller status\nBy probing Emisison Lamp negative terminal voltage"
        n1135 = Unbundle By Name(w2639) -> ("LJ Pinout.Laser Ready"=w2642:string)
        n1136 = call "LabJack_FGV.vi"("Operation(Read)"=enum16{"Write", "Read"}."Read" ("Operation")) -> ("Read data"=w2643:i32)  [unwired: 9 in, 1 out]
        n1137 = for {
          N: 10 -> [_]
          tunnel: w2643 -> [w2677]
          tunnel: w2642 -> [w2676]
          shift-right: [w2675] -> w2634
          shift-left: w2641 -> [w2674]
          tunnel: [w2672] -> w2632 mode=indexing
          n1138 = call <vilib>:"LJM_eReadName.vi"("Handle In"=w2677, "Name"=w2676, "error in"=w2674) -> ("Value"=w2672:dbl, "error out"=w2675:errorcluster)  [unwired: 10 in, 1 out]
          n1139 = Wait (ms)(milliseconds to wait=u32 50) -> ()  [unwired: 1 out]
        }
        n1140 = case shown="No Error" w2634 {
          selector: w2634 -> [w2651 w2670]
          tunnel: [w2653 FALSE] -> w2636
          tunnel: [w2652 w2670] -> w2635
          tunnel: [w2647 nan] -> w2633
          tunnel: w2632 -> [w2649 _]
          frame No Error {
            n1141 = call-poly <vilib>:"Mean.vi"("X"=w2649) -> ("mean"=w2647:dbl)  [unwired: 1 out]
            n1142 = Less?(x=w2647, y=2.0) -> (x < y?=w2648:bool)
            n1143 = case shown="False" w2648 {
              tunnel: [w2656 TRUE] -> w2653
              tunnel: w2647 -> [w2659 _]
              tunnel: w2651 -> [w2655 w2666]
              tunnel: [w2654 w2666] -> w2652
              frame False {
                n1144 = Greater?(x=w2659, y=9.0) -> (0:w2657:bool)
                n1145 = case shown="False" w2657 {
                  tunnel: [FALSE FALSE] -> w2656
                  tunnel: w2655 -> [_ w2663]
                  tunnel: [errorcluster {"status"=TRUE, "code"=5002, "source"="355 Laser"} ("error out") w2663] -> w2654
                  frame False {
                    n1146 = property on="355 Laser" class="Bool (strict)"("Blinking"=FALSE) -> ()  [unwired: 2 in, 2 out]
                  }
                  frame True {
                    n1147 = property on="355 Laser" class="Bool (strict)"("Blinking"=FALSE) -> ()  [unwired: 2 in, 2 out]
                  }
                }
              }
              frame True {
                n1148 = property on="355 Laser" class="Bool (strict)"("Blinking"=FALSE) -> ()  [unwired: 2 in, 2 out]
              }
            }
          }
          frame Error {
          }
        }
        "laser EM lamp V" <- w2633
        n1149 = Bundle By Name(cluster=w2639, "System Status.355 Laser"=w2636) -> (w2640:T16)
        n1150 = call <vilib>:"Add State(s) to Queue__JKI_lib_State_Machine.vi"("State(s) in (\"\")"=w2646) -> ("States Out"=w2645:string)  [unwired: 14 in]
      }
      frame "355 Laser: CheckPWMStatus" {
        # "Check 355 laser PWM status\n(Read LJ DIO#EF_ENABLE register to determine PWM status)"
        n1151 = Unbundle By Name(w2687) -> ("LJ Pinout.355 PWM"=w2686:string)
        n1152 = call "LabJack_FGV.vi"("Operation(Read)"=enum16{"Write", "Read"}."Read" ("Operation"), "error in (no error)"=w2680) -> ("error out"=w2683:errorcluster, "Read data"=w2684:i32)  [unwired: 8 in]
        n1153 = Concatenate Strings(w2686, "_EF_ENABLE" ("string")) -> (w2682:string)
        n1154 = call <vilib>:"LJM_eReadName.vi"("Handle In"=w2684, "Name"=w2682, "error in"=w2683) -> ("Value"=w2679:dbl, "error out"=w2681:errorcluster)  [unwired: 10 in, 1 out]
        n1155 = Greater Than 0?(x=w2679) -> (x > 0?=w2678:bool)
        n1156 = case shown="True" w2678 {
          frame False {
            # "PWM is off\nset color to dark green"
            n1157 = local write "355nm Laser toggle"(FALSE ("355nm Laser")) -> ()
          }
          frame True {
            # "PWM is on\nset color to light green"
            n1158 = local write "355nm Laser toggle"(TRUE ("355nm Laser")) -> ()
          }
        }
        n1159 = call <vilib>:"Add State(s) to Queue__JKI_lib_State_Machine.vi"("State(s) in (\"\")"=w2691) -> ("States Out"=w2690:string)  [unwired: 14 in]
      }
      frame "355 Laser: Start" {
        # "Template Separator\n(You can make a copy of, or modify, this frame)"
        n1160 = call <vilib>:"Add State(s) to Queue__JKI_lib_State_Machine.vi"("State(s) in Front (\"\")"="LabJack: 355_PWM_Start", "State(s) in (\"\")"=w2699) -> ("States Out"=w2698:string)  [unwired: 13 in]
      }
      frame "355 Laser: Stop" {
        # "Template Separator\n(You can make a copy of, or modify, this frame)"
        n1161 = call <vilib>:"Add State(s) to Queue__JKI_lib_State_Machine.vi"("State(s) in Front (\"\")"="LabJack: 355_PWM_Stop", "State(s) in (\"\")"=w2705) -> ("States Out"=w2704:string)  [unwired: 13 in]
      }
      frame "---------- Utility ----------" {
        # "Template Separator\n(You can make a copy of, or modify, this frame)"
        n1162 = call <vilib>:"Add State(s) to Queue__JKI_lib_State_Machine.vi"("State(s) in (\"\")"=w2710) -> ("States Out"=w2709:string)  [unwired: 14 in]
      }
      frame "Utility: RestoreDeConChan" {
        # "Template Separator\n(You can make a copy of, or modify, this frame)"
        n1163 = global read "GlobalVariables.vi" "DeconChan Temp"() -> (w2711:enum32{"No Selection", "Ch1", "Ch2", "Ch3"})
        n1164 = local write "Radio Buttons"(w2711) -> ()
        n1165 = call <vilib>:"Add State(s) to Queue__JKI_lib_State_Machine.vi"("State(s) in (\"\")"=w2716) -> ("States Out"=w2715:string)  [unwired: 14 in]
      }
      frame "Utility: SaveDeconChan" {
        # "Save Decon Channel to global temp\n(You can make a copy of, or modify, this frame)"
        n1166 = flat-sequence {
          frame #0 {
          }
          frame #1 {
            (unwired) enum32{"No Selection", "Ch1", "Ch2", "Ch3"}."No Selection" ("Radio Buttons")
          }
        }
        n1167 = flat-sequence {
          frame #0 {
            n1168 = local read "Radio Buttons"() -> (w2722:enum32{"No Selection", "Ch1", "Ch2", "Ch3"})
            n1169 = global write "GlobalVariables.vi" "DeconChan Temp"(w2722) -> ()
          }
          frame #1 {
            n1170 = local write "Radio Buttons"(enum32{"No Selection", "Ch1", "Ch2", "Ch3"}."No Selection" ("Radio Buttons")) -> ()
          }
        }
        n1171 = call <vilib>:"Add State(s) to Queue__JKI_lib_State_Machine.vi"("State(s) in (\"\")"=w2721) -> ("States Out"=w2720:string)  [unwired: 14 in]
      }
      frame "Utility: Dewelling" {
        # "Main loop dewell\n(Dewelling >> #)"
        n1172 = Fract/Exp String To Number(string=w2726, default (0 dbl)=0) -> (number=w2724:i32)  [unwired: 2 in, 1 out]
        n1173 = Wait (ms)(milliseconds to wait=w2724) -> ()  [unwired: 1 out]
        n1174 = call <vilib>:"Add State(s) to Queue__JKI_lib_State_Machine.vi"("State(s) in (\"\")"=w2731) -> ("States Out"=w2730:string)  [unwired: 14 in]
      }
      frame "Utility: SetAllChanManualGain" {
        # "Template Separator\n(You can make a copy of, or modify, this frame)"
        n1175 = property on="Auto gain ch1" class="Bool (strict)"("Val(Sgnl)"=FALSE ("Value (Signaling)")) -> ()  [unwired: 2 in, 2 out]
        n1176 = property on="Auto gain ch2" class="Bool (strict)"("Val(Sgnl)"=FALSE ("Value (Signaling)")) -> ()  [unwired: 2 in, 2 out]
        n1177 = property on="Auto gain ch3" class="Bool (strict)"("Val(Sgnl)"=FALSE ("Value (Signaling)")) -> ()  [unwired: 2 in, 2 out]
        n1178 = call <vilib>:"Add State(s) to Queue__JKI_lib_State_Machine.vi"("State(s) in (\"\")"=w2739) -> ("States Out"=w2738:string)  [unwired: 14 in]
      }
      frame "Utility: SetAllChanAutoGain" {
        # "Template Separator\n(You can make a copy of, or modify, this frame)"
        n1179 = property on="Auto gain ch1" class="Bool (strict)"("Val(Sgnl)"=TRUE ("Value (Signaling)")) -> ()  [unwired: 2 in, 2 out]
        n1180 = property on="Auto gain ch2" class="Bool (strict)"("Val(Sgnl)"=TRUE ("Value (Signaling)")) -> ()  [unwired: 2 in, 2 out]
        n1181 = property on="Auto gain ch3" class="Bool (strict)"("Val(Sgnl)"=TRUE ("Value (Signaling)")) -> ()  [unwired: 2 in, 2 out]
        n1182 = call <vilib>:"Add State(s) to Queue__JKI_lib_State_Machine.vi"("State(s) in (\"\")"=w2747) -> ("States Out"=w2746:string)  [unwired: 14 in]
      }
      frame "---------- SysLog ----------" {
        # "Template Separator\n(You can make a copy of, or modify, this frame)"
        n1183 = call <vilib>:"Add State(s) to Queue__JKI_lib_State_Machine.vi"("State(s) in (\"\")"=w2752) -> ("States Out"=w2751:string)  [unwired: 14 in]
      }
      frame "SysLog: OpenLogFile" {
        # "Template Separator\n(You can make a copy of, or modify, this frame)"
        n1184 = call <vilib>:"Add State(s) to Queue__JKI_lib_State_Machine.vi"("State(s) in (\"\")"=w2757) -> ("States Out"=w2756:string)  [unwired: 14 in]
      }
      frame "---------- Graph ----------" {
        # "Template Separator\n(You can make a copy of, or modify, this frame)"
        n1185 = call <vilib>:"Add State(s) to Queue__JKI_lib_State_Machine.vi"("State(s) in (\"\")"=w2762) -> ("States Out"=w2761:string)  [unwired: 14 in]
      }
      frame "Graph: AddCursors" {
        # "Add BG and DC cursor to all graphs\n(You can make a copy of, or modify, this frame)"
        n1186 = property on="Channel 2" class="WFGraph (strict)"() -> ("CrsrList"=w2766:T17)  [unwired: 2 in, 2 out]
        n1187 = property on="Channel 3" class="WFGraph (strict)"() -> ("CrsrList"=w2765:T17)  [unwired: 2 in, 2 out]
        n1188 = property on="Channel 1" class="WFGraph (strict)"() -> ("CrsrList"=w2770:T17)  [unwired: 2 in, 2 out]
        n1189 = for {
          tunnel: w2770 -> [w2783] mode=indexing
          tunnel: u32[] [200, 220, 10, 25] -> [w2779] mode=indexing
          tunnel: [w2782] -> w2768 mode=indexing
          tunnel: u32[] [6618880, 6618880, 16711680, 16711680] -> [w2778] mode=indexing
          tunnel: w2766 -> [w2781] mode=indexing
          tunnel: w2765 -> [w2780] mode=indexing
          tunnel: [w2777] -> w2764 mode=indexing
          tunnel: [w2776] -> w2763 mode=indexing
          n1190 = Bundle By Name(cluster=w2783, "Position.X"=w2779, "Color"=w2778) -> (w2782:T18)
          n1191 = Bundle By Name(cluster=w2781, "Position.X"=w2779, "Color"=w2778) -> (w2777:T18)
          n1192 = Bundle By Name(cluster=w2780, "Position.X"=w2779, "Color"=w2778) -> (w2776:T18)
        }
        n1193 = property on="Channel 1" class="WFGraph (strict)"("CrsrList"=w2768) -> ()  [unwired: 2 in, 2 out]
        n1194 = property on="Channel 2" class="WFGraph (strict)"("CrsrList"=w2764) -> ()  [unwired: 2 in, 2 out]
        n1195 = property on="Channel 3" class="WFGraph (strict)"("CrsrList"=w2763) -> ()  [unwired: 2 in, 2 out]
        n1196 = call <vilib>:"Add State(s) to Queue__JKI_lib_State_Machine.vi"("State(s) in (\"\")"=w2775) -> ("States Out"=w2774:string)  [unwired: 14 in]
      }
      frame "---------- Temp ----------" {
        # "Template Separator\n(You can make a copy of, or modify, this frame)"
        n1197 = call <vilib>:"Add State(s) to Queue__JKI_lib_State_Machine.vi"("State(s) in (\"\")"=w2788) -> ("States Out"=w2787:string)  [unwired: 14 in]
      }
    }
    n1198 = Not(x=w270) -> (.not. x?=w269:bool)
    n1199 = local write "ML?"(w269) -> ()
    "ML?" <- TRUE ("main loop running?")
  }
  n1200 = while {
    tunnel: w43 -> [w2801]
    tunnel: w32 -> [w2800]
    tunnel: [w2799] -> w41
    tunnel: w26 -> [w2798]
    tunnel: [w2797] -> w37
    tunnel: w8 -> [w2795]
    tunnel: w19 -> [w2794]
    tunnel: w3 -> [w2789]
    stop <- w2792 stop-if-true
    # "Data Aquisition Loop"
    n1201 = event shown="[1] <Start digitizer>: User Event" {
      selector: w2800 -> [_ _]
      dyn-events: [_ _] -> w2799
      timeout: 20 -> [_ _]
      tunnel: w2801 -> [w2807 w2812]
      tunnel: [w2802 _] -> w2792
      tunnel: w2798 -> [w2806 w2819]
      tunnel: [w2806 w2818] -> w2797
      tunnel: w2795 -> [_ w2816]
      tunnel: w2794 -> [w2805 w2811]
      tunnel: w2789 -> [_ w2808]
      event Timeout {
        # "use queue to stop data loop\nwhen queue ref is released, error will stop this loop"
        n1202 = event-data() -> ()  [unwired: 1 in, 3 out]
        n1203 = Get Queue Status(queue=w2805) -> (error out=w2803:errorcluster)  [unwired: 2 in, 7 out]
        n1204 = Get Queue Status(queue=w2807) -> (error out=w2804:errorcluster)  [unwired: 2 in, 7 out]
        n1205 = Merge Errors(w2804, w2803) -> (w2802:errorcluster)
      }
      event User Event {
        w2817 = enum16{"Write", "Read"}."Read" ("Operation")
        n1206 = event-data() -> ()  [unwired: 1 in, 4 out]
        n1207 = call "FLImDAQ_FGV.vi"() -> ("Read data"=w2814:T5)  [unwired: 10 in, 1 out]
        n1208 = Unbundle By Name(w2814) -> ("Waveform to Avg"=w2813:i32)
        n1209 = call "Digitizer1_FGV.vi"("Operation"=w2817) -> ("Read data"=w2809:refnum<k15>)  [unwired: 9 in, 1 out]
        n1210 = call "Digitizer2_FGV.vi"("Operation"=w2817) -> ("Read data"=w2815:refnum<k15>)  [unwired: 9 in, 1 out]
        n1211 = while {
          tunnel: w2819 -> [w2866]
          tunnel: [w2865] -> w2818
          tunnel: w2815 -> [w2859]
          tunnel: w2809 -> [w2858]
          tunnel: w2816 -> [w2856]
          shift-right: [w2845] -> _
          shift-left: u32 0 ("millisecond timer value") -> [w2844]
          tunnel: w2813 -> [w2841]
          tunnel: w2812 -> [w2838]
          tunnel: w2811 -> [w2836]
          tunnel: w2808 -> [w2823]
          i -> [w2840]
          stop <- w2831 stop-if-true
          w2828 = enum16{"write", "read"}."read" ("action")
          w2846 = 65536
          # "send data for processing"
          # "acquire data and send it to processing loop"
          n1212 = Tick Count (ms)() -> (millisecond timer value=w2845:u32)
          n1213 = Multiply(x=w2841, y=w2840) -> (x*y=w2820:i32)
          "Fetch Record #" <- w2820
          n1214 = Subtract(x=w2845, y=w2844) -> (x-y=→"Aquisition loop timing(ms)":u32)
          n1215 = property class="niScope"(reference=w2858, "Fetch Record Number"=w2820) -> (reference out=w2870:refnum<k15>, error out=w2869:errorcluster, "Records Done"=w2821:i32, "Vertical Range"=w2854:dbl, "Vertical Offset"=w2852:dbl)  [unwired: 1 in]
          n1216 = call-poly <instrlib>:"niScope Fetch (poly).vi"("timeout"=1.0, "error in"=w2869, "channels"="0,1", "instrument handle"=w2870) -> ("error out"=w2857:errorcluster, "wfm"=w2842:i16[][])  [unwired: 4 in, 2 out]
          "error out" <- w2857
          n1217 = property class="niScope"(reference=w2859, error in=w2857, "Fetch Record Number"=w2820) -> (reference out=w2863:refnum<k15>, error out=w2860:errorcluster, "Vertical Range"=w2848:dbl, "Vertical Offset"=w2847:dbl)
          n1218 = Divide(x=w2842, y=w2846) -> (x/y=w2855:dbl[][])
          n1219 = Subtract(x=w2821, y=w2820) -> (x-y=→"Record Backlog":i32)
          n1220 = Multiply(x=w2855, y=w2854) -> (x*y=w2853:dbl[][])
          n1221 = call "V1FGV.vi"("action"=w2828) -> ("Error Out"=w2830:errorcluster, "V1 out"=w2827:dbl)  [unwired: 9 in]
          n1222 = call-poly <instrlib>:"niScope Fetch (poly).vi"("timeout"=1.0, "error in"=w2860, "channels"="0,1", "instrument handle"=w2863) -> ("error out"=w2834:errorcluster, "wfm"=w2849:i16[][])  [unwired: 4 in, 2 out]
          "error out 2" <- w2834
          n1223 = call "V2FGV.vi"("Error In"=w2830, "action"=w2828) -> ("Error Out"=w2829:errorcluster, "V2 out"=w2826:dbl)  [unwired: 8 in]
          n1224 = Add(x=w2853, y=w2852) -> (x+y=w2837:dbl[][])
          n1225 = call "V3FGV.vi"("Error In"=w2829, "action"=w2828) -> ("V3 out"=w2825:dbl)  [unwired: 8 in, 1 out]
          n1226 = Divide(x=w2849, y=w2846) -> (x/y=w2851:dbl[][])
          n1227 = Enqueue Element(queue=w2838, element=w2837) -> (error out=w2833:errorcluster)  [unwired: 2 in, 2 out]
          n1228 = Bundle("V1 out"=w2827, "V2 out"=w2826, "V3 out"=w2825) -> (w2824:T32)  [unwired: 1 in]
          n1229 = Multiply(x=w2851, y=w2848) -> (x*y=w2850:dbl[][])
          n1230 = Add(x=w2850, y=w2847) -> (x+y=w2835:dbl[][])
          n1231 = Enqueue Element(queue=w2823, element=w2824) -> (error out=w2822:errorcluster)  [unwired: 2 in, 2 out]
          n1232 = Enqueue Element(queue=w2836, element=w2835) -> (error out=w2832:errorcluster)  [unwired: 2 in, 2 out]
          n1233 = Bundle(w2840, w2837, w2835) -> (w2839:cluster{i32, dbl[][], dbl[][]})  [unwired: 1 in]
          n1234 = Merge Errors(w2822, w2832, w2833, w2834) -> (w2831:errorcluster)
          "aquisition loop Error Out" <- w2831
          n1235 = Send Notification(notification=w2839, notifier=w2866) -> (notifier out=w2865:refnum<notifier>)  [unwired: 1 in, 1 out]
          n1236 = case shown="Error .." w2831 {
            tunnel: w2856 -> [_ w2873]
            frame No Error {
            }
            frame Error {
              # "Send user event to signal aquisition has stoped"
              n1237 = Generate User Event(priority (normal)=usereventprio."high priority", user event=w2873, event data cluster=TRUE ("event data")) -> ()  [unwired: 1 in, 2 out]
            }
          }
        }
      }
    }
    n1238 = Unbundle By Name(w2792) -> ("status"=w2791:bool)
    n1239 = Not(x=w2791) -> (.not. x?=w2790:bool)
    n1240 = local write "Aq L?"(w2790) -> ()
    "Aq L?" <- TRUE ("Aq L?")
  }
  n1241 = Control Help Window(0:w1, 1:TRUE ("Show")) -> ()
  n1242 = Unregister For Events(event registration refnum=w17, error in=w28) -> (error out=w29:errorcluster)
  n1243 = Destroy User Event(user event=w8, error in=w29) -> ()  [unwired: 1 out]
  n1244 = Release Notifier(notifier=w37, error in (no error)=w36) -> (error out=w35:errorcluster)  [unwired: 1 in, 2 out]
  n1245 = Unregister For Events(event registration refnum=w41, error in=w39) -> (error out=w40:errorcluster)
  n1246 = Release Notifier(notifier=w22, error in (no error)=w20) -> (error out=w21:errorcluster)  [unwired: 1 in, 2 out]
  n1247 = Release Notifier(notifier=w13, error in (no error)=w7) -> (error out=w12:errorcluster)  [unwired: 1 in, 2 out]
  n1248 = call <vilib>:"Simple Error Handler.vi"("error in (no error)"=w35) -> ()  [unwired: 4 in, 5 out]
  n1249 = Destroy User Event(user event=w30, error in=w40) -> ()  [unwired: 1 out]
  n1250 = call <vilib>:"Simple Error Handler.vi"("error in (no error)"=w21) -> ()  [unwired: 4 in, 5 out]
  n1251 = call <vilib>:"Simple Error Handler.vi"("error in (no error)"=w12) -> ()  [unwired: 4 in, 5 out]
  n1252 = disable-structure shown="Disabled" {
    frame Disabled {
      n1253 = flat-sequence {
        tunnel: _ -> [w2874]
        tunnel: _ -> [w2879]
        frame #0 {
          n1254 = Two Button Dialog(message="Save data?", 1:"No" ("F button name (\"Cancel\")"), 2:"Yes" ("T button name (\"OK\")")) -> (T button?=w2875:bool)
          n1255 = case shown="True" w2875 {
            tunnel: w2879 -> [_ w2881]
            tunnel: w2874 -> [_ w2880]
            frame False {
            }
            frame True {
              n1256 = flat-sequence {
                tunnel: w2881 -> [w2882]
                tunnel: w2880 -> [w2884]
                frame #0 {
                  n1257 = call-poly <vilib>:"Write Delimited Spreadsheet.vi"("format (%.3f)"="%.6f", "2D data"=w2882) -> ()  [unwired: 12 in, 2 out]
                }
                frame #1 {
                  n1258 = call-poly <vilib>:"Write Delimited Spreadsheet.vi"("format (%.3f)"="%.6f", "1D data"=w2884, "delimiter (\\t)"="\r\n") -> ()  [unwired: 11 in, 2 out]
                }
              }
            }
          }
        }
      }
    }
    frame Enabled {
    }
  }
